vi "UHR-Fleezers Control (host) - 9.1.vi"() -> ()   [LabVIEW 2009]
uses:
  <vilib>/Utility/miscctls.llb/LVPoint32TypeDef.ctl
  <vilib>/Utility/miscctls.llb/LVMinMaxIncTypeDef.ctl
  <vilib>/userDefined/High Color/nirio_resource_hc.ctl
  <vilib>/Instr/_visa.llb/VISA Configure Serial Port (Instr).vi
  <vilib>/Platform/TimedLoop/XDataNode/XDataNode.xnode
  <vilib>/Platform/TimedLoop/XDataNode/loadlvalarms.vi
  <vilib>/Platform/TimedLoop/XDataNode/timing_clust.ctl
  <vilib>/Platform/TimedLoop/XDataNode/nitl_modes.ctl
  <vilib>/Platform/TimedLoop/XDataNode/wakeup.ctl
  <vilib>/rvi/interface/nirviOpenFPGA/nirviOpenFPGA.xnode
  FPGA Bitfiles/UHR-Fleezers Instr~3C_FPGA Target_UHR-Fleezers Contr~E1.lvbitx
  UHR-Fleezers Control (fpga) - 9.0.vi
  <vilib>/FPGAPlugInAG/PCIe-7852R/nirviIntfOpen_PCIe-7852R.vi
  <vilib>/rvi/interface/nirviMethod/nirviMethod.xnode
  <vilib>/Utility/error.llb/Merge Errors.vi
  <vilib>/LabVIEW Targets/FPGA/Rio/nirio_HostInterface/nirio_Reset.vi
  <vilib>/LabVIEW Targets/FPGA/Rio/nirio_HostInterface/nirio_DMAStopAll.vi
  <vilib>/rvi/interface/common/niFpgaNodeNameForErrorReporting.ctl
  <vilib>/rvi/errors/niLvFpgaWhatHappensToTopLevelVI.ctl
  <vilib>/LabVIEW Targets/FPGA/Rio/nirio_HostInterface/nirio_DisableInterrupts.vi
  <vilib>/Utility/error.llb/Error Cluster From Error Code.vi
  <vilib>/rvi/errors/niLvFpgaAdjustHostInterfaceError.vi
  <vilib>/rvi/interface/nirviReadWriteControl/nirviReadWriteControl.xnode
  <vilib>/LabVIEW Targets/FPGA/Rio/nirio_HostInterface/nirio_WriteBig.vi
  <vilib>/LabVIEW Targets/FPGA/Rio/nirio_HostInterface/nirio_DMAConfigure.vi
  <vilib>/LabVIEW Targets/FPGA/Rio/nirio_HostInterface/nirio_DMAStop.vi
  <vilib>/RVI Host/nirviSupport.llb/nirviErrorClusterFromErrorCode.vi
  <vilib>/LabVIEW Targets/FPGA/Rio/nirio_HostInterface/nirio_EnableInterrupts.vi
  <vilib>/rvi/errors/niLvFpgaReportInternalErrorWithAdditionalInfo.vi
  <vilib>/express/express analysis/Spectral/XNode/ExpressSpectralMeasurementsBlockNode.xnode
  <vilib>/express/express analysis/Spectral/Block/exnSpectralBlock spectral measurements PSD poly.vi
  <vilib>/express/express analysis/Spectral/Block/exnSpectralBlock spectral measurements PSD WFM.vi
  <vilib>/Waveform/WDTOps.llb/WDT Append Waveforms DBL.vi
  <vilib>/LabVIEW Targets/FPGA/Rio/nirio_HostInterface/nirio_ReadBig.vi
  <vilib>/vision/Avi1.llb/AviRefnum.ctl
  <vilib>/rvi/interface/nirviCloseFPGA/nirviCloseFPGA.xnode
  <vilib>/FPGAPlugInAG/PCIe-7852R/nirviIntfClose_PCIe-7852R.vi
  <vilib>/Analysis/NI_AALBase.lvlib
  <vilib>/Platform/TimedLoop/XDataNode/XDNodeRunTimeDep.lvlib
  openfpgaref.8.6.ctl
  NiRioSrv.dll
panel:
  in  "Total Volume\nFlushed (uL)":dbl
  in  "Flush Center Channel":bool
  in  "Inject Bottom Channel":bool
  in  "Inject Top Channel":bool
  out "Messages":string
  in  "APD Ave N":dbl=10.0
  out "Int. Time (s)":dbl
  in  "Stop All":bool
  out "sigma/mean":dbl
  out "Rate sigma (Hz)":dbl format="%0.2f"
  out "Current Stage  Position":cluster{dbl, dbl, dbl}
  in  "Index":dbl=1.0 caption="Save File Index" min=1.0 step=1.0
  in  "Tab Control 6":T1(tab)
  out "All Signals":waveform(dbl)[](graph)
  in  "Signals to Plot":i32(listbox)
  out "Trap Disp. Freq. (Hz)":dbl caption="Freq. (Hz)" format="%#_6p"
  out "Display Period (s)":dbl caption="Period (s)" format="%#_6p"
  in  "Trap Disp. Downsample":dbl=5000.0 caption="Downsample"
  in  "APD Disp. Scale":dbl=0.1 caption="Scale (Divide,\nfor above plot only)"
  in  "APD Disp. Downsample":dbl=30.0 caption="Integrate" min=1.0 step=1.0
  out "APD Display Freq. (Hz)":dbl caption="Freq. (Hz)"
  out "APD Display Period (s)":dbl caption="Period (s)"
  out "RMS (Ang)":dbl format="%_2g"
  in  "Bead Sep. Int. Time (s)":dbl=5.0 caption="Int. Time (s)"
  in  "Below (kHz)":dbl=1.0
  in  "Above (kHz)":dbl=4.0
  in  "Adjust Scale\nto Mean":bool
  in  "Rescale on Mean":bool
  in  "Offset (nm)":dbl
  out "Mean":dbl caption="Mean (pN)" format="%#_4g"
  out "Force":waveform(dbl)[](graph)
  out "APD 1 Chart":waveform(dbl)(graph)
  in  "Calibration":u16(ring)=2 items=["None", "Position", "Force"]
  out "T1 X":dbl caption="T1 X (pN)" format="%0.2f"
  out "T2 X":dbl caption="T2 X (pN)" format="%0.2f"
  out "Bead Separation":waveform(dbl)(graph)
  in  "Amplitude (nm)":dbl=1.0
  out "Bead Mean (nm)":dbl caption="Mean (nm)" format="%0.2f"
  out "Difference":dbl caption="Difference (pN)" format="%#_3g"
  out "FFT 1":cluster{"f0":dbl, "df":dbl, "magnitude":dbl[]}[](graph)
  out "FFT 2":cluster{"f0":dbl, "df":dbl, "magnitude":dbl[]}[](graph)
  in  "FFT 1 Choice 1":u16(ring) items=["T1 Y", "T1 X", "T1 Sum", "T2 Y", "T2 X", "T2 Sum", "T1 FB X", "T1 FB Sum", "T2 FB X", "T2 FB Sum", "PSD Y", "PSD X", "PSD Y Sum", "none"]
  in  "FFT 2 Choice 1":u16(ring)=13 items=["T1 Y", "T1 X", "T1 Sum", "T2 Y", "T2 X", "T2 Sum", "T1 FB X", "T1 FB Sum", "T2 FB X", "T2 FB Sum", "PSD Y", "PSD X", "PSD Y Sum", "none"]
  in  "FFT 1 Choice 2":u16(ring)=1 items=["T1 Y", "T1 X", "T1 Sum", "T2 Y", "T2 X", "T2 Sum", "T1 FB X", "T1 FB Sum", "T2 FB X", "T2 FB Sum", "PSD Y", "PSD X", "PSD Y Sum", "none"]
  in  "FFT 2 Choice 2":u16(ring)=13 items=["T1 Y", "T1 X", "T1 Sum", "T2 Y", "T2 X", "T2 Sum", "T1 FB X", "T1 FB Sum", "T2 FB X", "T2 FB Sum", "PSD Y", "PSD X", "PSD Y Sum", "none"]
  in  "Compute FFT":bool
  in  "Reset FFT":bool
  in  "# Spectra to Ave.":dbl=10.0
  out "Ave. Time (s)":dbl
  out "1 Channel":waveform(dbl)(graph)
  out "Slow mean":dbl format="%0.2f"
  in  "Slow mean N ave.":dbl=1.0 min=1.0 step=1.0
  out "Mean Intensity":dbl
  out "Sigma":dbl
  out "Sigma/Mean":dbl
  in  "Subtract mean":bool
  in  "High Res. Display":u16(ring) items=["T1 Y", "T1 X", "T1 Sum", "T2 Y", "T2 X", "T2 Sum", "T1 FB X", "T1 FB Sum", "T2 FB X", "T2 FB Sum", "PSD Y", "PSD X", "PSD Y Sum"]
  out "APD 1 Rate (Hz)":dbl format="%#_3p"
  out "Image":u32[][](graph)
  in  "Tab Control":T2(tab)=enum."Sample Stage"
  in  "Read Cal":bool
  out "Tether":bool
  in  "Tether Alarm?":bool=TRUE
  in  "Move to Delta (MHz)":dbl=15.6
  in  "Then...":string(combo)="2"
  in  "Data Acq. Spot":bool
  out "Fl. High":bool
  out "Waiting":bool
  in  "Yank to Freq. (MHz)":dbl
  in  "Fl. Threshold (kHz)":dbl
  in  "Fl. Triggered...":bool
  in  "Confocal Linescan":bool
  in  "Speed (nm/s)":dbl=100.0
  in  "Stop F (pN)":dbl=4.0
  in  "Furthest Withdraw (MHz)":dbl=15.0
  in  "Closest Delta (MHz)":dbl=10.0 step=0.25
  in  "Fish for Tether":bool
  in  "Confocal Image":bool
  in  "Round T1 X":bool caption="Round"
  in  "T1 offset_x (mV)":dbl=-26.302542012392074 format="%#_2g"
  in  "T1 kappa_x (pN/nm)":dbl=0.22546432407642192 min=0.0 step=0.001 format="%#_2g"
  out "Time (s)":dbl
  out "Total Time (s)":dbl
  in  "Start Saving":bool
  in  "Limits Enable":bool=TRUE caption="Enable"
  in  "Limit Max (MHz)":dbl=16.0 caption="Max (MHz)"
  in  "Limit Min (MHz)":dbl=10.0 caption="Min (MHz)"
  in  "Cal sets to save":u32=50 min=1 step=1
  in  "Comment (data description)":string="testing confocal setup"
  out "Calibrating Trap...":bool
  in  "Trap 2 (ON/OFF)":bool
  in  "Trap 1 (ON/OFF)":bool
  in  "Save Calibration":bool
  in  "N sets to save":u32=200 caption="N Sets"
  in  "Save N Sets":bool
  out "Save file name":path
  in  "Save ave N":dbl=250.0 caption="Averaging Factor"
  out "Saving...":bool
  in  "Stop Saving":bool
  out "Progress":u16(slide) scale=0.0..100.0
  out "Manipulating Trap":bool
  out "Buffer Status":dbl(slide) scale=0.0..1.0
  out "Overflow (data lost)":bool
  in  "Reset":bool
  out "Data Rate (Hz)":dbl caption="Trap Data Rate (Hz)" format="%#_3p"
  out "Data Period (s)":dbl caption="Trap Data Period (s)" format="%#_6p"
  out "Save Data Rate (Hz)":dbl caption="Rate (Hz)" format="%#_6p"
  out "Save Data Period (s)":dbl caption="Period (s)" format="%#_6p"
  in  "T1 alpha_x (nm/V)":dbl=630.439304367558 step=10.0 format="%#_3g"
  in  "T2 alpha_x (nm/V)":dbl=704.7738222964198 step=10.0 format="%#_3g"
  in  "T2 kappa_x (pN/nm)":dbl=0.2030110880477556 min=0.0 step=0.001 format="%#_2g"
  in  "T2 offset_x (mV)":dbl=-26.67973517613748 format="%#_2g"
  in  "BD 1 Frequency 1 (MHz)":dbl=69.4 caption="T1 X (MHz)" min=60.0 max=90.0 step=1.0 format="%#_6p"
  in  "BD 1 Frequency 2 (MHz)":dbl=85.0 caption="T2 X (MHz)" min=60.0 max=90.0 step=1.0 format="%#_6p"
  in  "Green Laser ON/Interlacing":bool
  in  "Round T2 X":bool caption="Round"
  in  "AO1":dbl(slide)=4.8 caption="Confocal Y (V)" min=0.0 max=10.0 step=0.01 scale=0.0..10.0 scale format="%_1f"
  in  "AO2":dbl(slide)=3.2 caption="Confocal X (V)" min=0.0 max=10.0 step=0.01 scale=0.0..10.0 scale format="%_1f"
  in  "Upper Cap.":bool
  in  "Lower Cap.":bool
  in  "Trap Raster Scan":bool
  out "Raster Scanning...":bool
  in  "Trap Delta (MHz)":dbl=15.599999999999994
  in  "Action":string(combo)="Alarm"
  in  "Dump Beads":bool
  out "Duration (s)":dbl
  out "Stage Moving":bool
  in  "Wait Before Save (s)":u32=1
  out "Attempts":dbl
  in  "Attempt Limit":dbl=20.0 caption="Limit"
  in  "z nudge increment (um)":dbl=0.5
  in  "+z":bool
  in  "Saved Stage Positions":T3={"Position 1"={1.03657, -0.89848, 0.0}, "Position 2"={0.0, 0.0, 0.0}, "Position 3"={2.01196, -0.50288, 0.0}, "Position 4"={2.01196, 0.31084, 0.0}} {"Position 1"."?" min=-0.1 max=0.1 step=0.1; "Position 2"."?" min=-0.1 max=0.1 step=0.1; "Position 3"."?" min=-0.1 max=0.1 step=0.1; "Position 4"."?" min=-0.1 max=0.1 step=0.1}
  in  "Position 1 Label":string="Upper capillary"
  in  "Set Position 1":bool
  in  "Set Position 2":bool
  in  "Set Position 3":bool
  in  "Set Position 4":bool
  in  "Move to Position 3":bool
  in  "Move to Position 4":bool
  in  "Move to Position 2":bool
  in  "Move to Position 1":bool
  in  "Position 2 Label":string="Lower capillary"
  in  "Position 3 Label":string="Measurement Spot"
  in  "Position 4 Label":string="Dump beads"
  in  "-z":bool
  in  "Top Ch Inject Rate (ul/h)":dbl=10.0
  in  "Pump write delay (ms)":dbl=300.0
  in  "All Pump Parameters":T4={"Pump 1"={"Diameter (mm)"=4.61, "Units"=3.0, "Volume"=100.0, "Rate"=100.0}, "Pump 2"={"Diameter (mm)"=4.61, "Units"=3.0, "Volume"=100.0, "Rate"=100.0}, "Pump 3"={"Diameter (mm)"=4.61, "Units"=3.0, "Volume"=100.0, "Rate"=100.0}}
  in  "Top Ch Inject Volume (uL)":dbl=100.0
  in  "Pump pause delay (ms)":u32
  in  "Bottom Ch Inject Volume (uL)":dbl=100.0
  in  "Bottom Ch Inject Rate (ul/h)":dbl=10.0
  in  "Flush Center Ch Volume (uL)":dbl=15.0
  in  "Flush Center Ch Rate (ul/m)":dbl=100.0
  in  "Tab Control 2":T5(tab)=enum."Feedback on BD 1 Amp to Control AI2"
  out "Total Counts (ticks)":u32
  in  "Trap ON/OFF X or Y Amp?":bool=TRUE
  in  "Oscillate Set 1":bool
  in  "Trap 1 ON":bool
  in  "Number Interlace Sets":u8=3 min=1 max=3
  in  "DIO count 3 (ticks)":u32=200
  in  "DIO count 2 (ticks)":u32=200
  in  "DIO count 1 (ticks)":u32=200
  in  "BD 2 Amplitude 3 (%)":dbl min=0.0 max=50.0 step=1.0
  in  "BD 2 Amplitude 2 (%)":dbl min=0.0 max=50.0 step=1.0
  in  "BD 2 Amplitude 1 (%)":dbl min=0.0 max=50.0 step=1.0
  in  "BD 1 Amplitude 3 (%)":dbl min=0.0 max=50.0 step=1.0
  in  "BD 1 Amplitude 2 (%)":dbl=35.0 min=0.0 max=50.0 step=1.0
  in  "BD 1 Amplitude 1 (%)":dbl=10.0 min=0.0 max=50.0 step=1.0
  in  "BD 2 Frequency 3 (MHz)":dbl=26.0 min=0.0 max=40.0 step=1.0 format="%#_6p"
  in  "BD 1 Frequency 3 (MHz)":dbl=70.0 min=60.0 max=90.0 step=1.0 format="%#_6p"
  in  "BD 2 Frequency 2 (MHz)":dbl=26.0 min=0.0 max=40.0 step=1.0 format="%#_6p"
  in  "BD 2 Frequency 1 (MHz)":dbl=26.0 min=0.0 max=40.0 step=1.0 format="%#_6p"
  in  "Not-Interlacing Set":enum32{"Set 1", "Set 2", "Set 3"}(radio)
  in  "Interlace":bool=TRUE
  in  "Trap 2 ON":bool
  in  "Trap 3 ON":bool
  in  "Scan axis 2":bool=TRUE
  in  "Osc. freq. (Hz)":dbl=0.25
  in  "Osc. amp. (MHz)":dbl=2.0
  out "Coords":T6
  in  "Manipulation Scaling":cluster{"Horizontal":dbl, "Vertical":dbl}={"Horizontal"=0.075, "Vertical"=0.01}
  in  "Freq or Amp switch first":bool=TRUE
  in  "Swap F1 and F2":bool
  in  "Freq switch delay":u16
  in  "Amp switch delay":u16=5
  in  "MCL Step Increment (V_int)":dbl=3.0
  out "Time to Finish All (min)":dbl format="%#_2p"
  in  "Scan Speed (nm/s)":dbl=100.0
  in  "Scan Range (nm)":dbl=750.0
  in  "Step Size (nm)":dbl=1.0
  in  "MCL/AOM Scale Tweak":dbl=1.0
  in  "MCL Step Position Ratio":dbl=0.5
  in  "Move MCL Also?":bool=TRUE
  out "Final sep (nm)":dbl
  out "Initial sep (nm)":dbl
  out "Save index":dbl
  out "Final delta (MHz)":dbl
  out "Initial delta (MHz)":dbl
  out "Final freq. (MHz)":dbl
  out "Initial freq. (MHz)":dbl
  in  "Saved AOD Raster Scan Parameter Sets":T7(array[cluster])=[{"Scan Range AOD (nm) 2"=500.0, "Step Size AOD (nm) 2"=1.0, "Scan Speed AOD (nm/s) 2"=200.0, "Number of scans (AOD) 2"=1, "Label"=""}, {"Scan Range AOD (nm) 2"=1000.0, "Step Size AOD (nm) 2"=1.0, "Scan Speed AOD (nm/s) 2"=200.0, "Number of scans (AOD) 2"=5, "Label"="wide offset scan"}, {"Scan Range AOD (nm) 2"=20.0, "Step Size AOD (nm) 2"=0.68, "Scan Speed AOD (nm/s) 2"=0.68, "Number of scans (AOD) 2"=1, "Label"="2 bp steps"}]
  in  "Load parameters":bool
  out "Scan Range (MHz)":dbl=10.0
  in  "Restart DMA? (AOD)":bool=TRUE caption="Restart DMA?"
  out "Incr. int (AOD)":i64
  out "Time/Scan (s) (AOD)":dbl format="%#_2p"
  out "Data points/scans":dbl
  out "Data points/scan (f/b)":dbl
  in  "Save scans":bool=TRUE
  out "AOD Scan I":u64 caption="Scan I"
  in  "Continuous AOD Scanning":bool caption="Continuous Scanning"
  in  "Abort AOD Scan":bool caption="Abort Scan"
  in  "Scan BD":bool=TRUE
  out "Cycles/step (AOD)":u64=400 format="%.0p"
  in  "Number of F/B Scans (AOD)":u16=3 min=1
  out "Scan steps (AOD)":u64=1000
  out "Scan Increment (MHz)":dbl=0.2
  out "AOD Scanning":bool caption="Scanning"
  in  "Start AOD Scan":bool caption="Start Scan"
  out "N sets should be saved":dbl
  out "Progress 2":u16(slide) caption="Progress" scale=0.0..100.0
  in  "Abort save 2":bool caption="Abort save"
  in  "Trap 1 Bead Size (nm)":dbl=860.0
  in  "Trap 2 Bead Size (nm)":dbl=790.0
  out "MCL Count":dbl
  in  "All FB On/Off":bool=TRUE
  in  "AI2 to Setpoint":cluster{"Set 1":bool, "Set 2":bool}
  out "AI2 (V)":cluster{"Set 1":dbl, "Set 2":dbl}
  in  "Reset Feedback":cluster{"Set 1":bool, "Set 2":bool}
  in  "PID Gains":T8={"Set 1"={"proportional gain (Kc)"=0, "integral gain (Kc*Ts/Ti)"=5, "derivative gain (Kc*Td/Ts)"=0}, "Set 2"={"proportional gain (Kc)"=0, "integral gain (Kc*Ts/Ti)"=5, "derivative gain (Kc*Td/Ts)"=0}}
  in  "Setpoints (V)":cluster{"Set 1":dbl, "Set 2":dbl}={"Set 1"=7.0, "Set 2"=7.0}
  in  "Feedback On/Off":cluster{"Set 1":bool, "Set 2":bool}={"Set 1"=TRUE, "Set 2"=TRUE}
  in  "Tab Control 3":enum32{"Timing", "MCL Scan", "Analog Out"}(tab)
  out "APD Gate Late Counter":u32
  in  "- phase (APD Gate)":bool
  in  "+ phase (APD Gate)":bool
  out "APD Gate Relative Phase":i16
  in  "Phase Adj. (APD Gate)":i16=20
  in  "Initial Phase Adjustment (APD Gate)":i16=95
  in  "Save APD Data\nwith Trap Data":bool=TRUE
  out "APD FIFO Elements Remaining":u32
  in  "- phase (APD Acq)":bool
  in  "+ phase (APD Acq)":bool
  out "APD Acq Late Counter":u32
  out "APD Acq Relative Phase":i16
  in  "Phase Adj. (APD Acq)":i16=20
  in  "Initial Phase Adjustment (APD Acq)":i16
  in  "Invert APD Gate":bool caption="Invert Gate"
  in  "APD Gate OFF Count":u32=450 caption="Gate OFF Count"
  in  "APD Gate ON Count":u32=150 caption="Gate ON Count"
  in  "APD Gate":enum32{"ON", "OFF", "Interlace"}(radio)=enum."Interlace"
  in  "APD Integration Time (s)":dbl=0.01 caption="Integration Time (s)"
  out "APD Acq Rate (Hz)":dbl=20000000.0 caption="Rate (Hz)"
  out "APD Samples/FIFO Acq.":dbl
  out "APD Elements/DMA read":u32
  out "APD Int. Count":u32 format="%.0p"
  in  "Tab Control 8":enum32{"APD 1 Image", "APD 1 Line Scan"}(tab)
  out "APD 1 map":dbl[][](graph)
  out "Waveform Graph":dbl[](graph)
  in  "Tab Control 5":enum32{"PSD X", "PSD Y", "Other Data Channel"}(tab)
  out "PSD X map":dbl[][](graph)
  out "PSD Y map":dbl[][](graph)
  out "Data map":dbl[][](graph)
  in  "Channel":i32=4
  in  "Abort MCL Scan":bool
  out "MCL Scan I":u64
  out "MCL Scanning":bool
  in  "Start MCL Scan":bool
  out "wait to reset values":bool
  in  "Tab Control 4":enum32{"Scan Settings", "MCL FPGA Loop Timing"}(tab)
  out "Total Time (s)":dbl
  in  "Scan lines":u64=10
  in  "Fast Scan Dir":bool=TRUE
  in  "2D or 1D Scan":bool=TRUE
  out "Initial X":dbl
  out "Initial Y":dbl
  out "Time/f+b scan (s) (MCL)":dbl caption="Time/scan (s)"
  in  "Number of scans (MCL)":u64=1 caption="Scans"
  in  "Scan steps (MCL)":u64=20 caption="Scan steps"
  in  "N APD Samp/step":dbl=6.0
  in  "Scan Range (V)":dbl=3.0
  in  "Restart DMA? (MCL)":bool=TRUE caption="Restart DMA?"
  in  "Continuous MCL Scanning":bool caption="Cont. Scanning"
  in  "Center Scan":bool=TRUE
  in  "Save Data (MCL)":bool=TRUE caption="Save Data"
  out "Incr. int (MCL)":i16 caption="Incr. int"
  out "Actual incr":dbl
  out "Scan Increment (V)":dbl
  out "N sets should be saved (MCL)":dbl caption="N sets should be saved"
  out "Data points/scans (MCL)":dbl caption="Data points/scans"
  out "Data points/scan (f+b)":dbl caption="points/scan (f+b)"
  out "Cycles/step (MCL)":u64 caption="Cycles/step" format="%.0p"
  in  "Phase adjust (MCL)":i16 caption="Phase adjust"
  out "Relative Phase (MCL)":i16 caption="Relative Phase"
  in  "Initial Phase Adj. (MCL)":i16 caption="Initial Phase Adj."
  in  "Update Count (MCL)":u32=800
  in  "+ phase (MCL)":bool
  in  "- phase (MCL)":bool
  out "MCL Late Counter":u32
  in  "APD 1 AO Mult.":i16=1 min=1
  in  "APD 2 AO Mult.":i16=1 min=1
  in  "APD 1 AO offset":i16
  in  "APD 2 AO offset":i16
  in  "Tab Control 7":enum32{"Green FB Signals", "Slow MCL Scan"}(tab)
  out "Green FB Plot":dbl(graph)
  out "MCL Scan 2":cluster{"Begin (V)":dbl, dbl, dbl[]}(graph)
  out "MCL Scan":cluster{"Begin (V)":dbl, dbl, dbl[]}(graph)
  in  "Green laser mode":enum32{"Laser ON", "Laser OFF", "Interlace"}(radio)=enum."Interlace"
  in  "GI Frequency, ON count":u32=150 min=1 step=1
  in  "Invert GI":bool
  out "GI Late Counter":u32
  in  "Phase adj. (GI)":i16=5
  out "GI relative phase":i16
  in  "+ phase (GI)":bool
  in  "Initial Phase Adjustment (GI)":i16=15
  in  "GI Frequency, OFF count":u32=450 min=1 step=1
  in  "- phase (GI)":bool
  out "Green FB Signals (V)":cluster{"Y":dbl, "X":dbl, "Sum":dbl}
  out "Relative phase (Green FB)":i16
  in  "+ phase (Green FB)":bool
  in  "- phase (Green FB)":bool
  in  "Green FB Count":u32=600
  in  "Phase adj. (Green FB)":i16=10
  in  "Initial Phase Adjustment (Green FB)":i16=50
  in  "Green FB On/Off":bool=TRUE
  in  "Current When FB OFF (%)":dbl=65.0 min=0.0 max=100.0 step=1.0
  in  "Green int current ON count adj":u32=150
  in  "Green FB Gains":T9={"proportional gain (Kc)"=10, "integral gain (Kc*Ts/Ti)"=5, "derivative gain (Kc*Td/Ts)"=0}
  in  "Green FB Setpoint (mV)":dbl=125.0
  in  "- phase (GI) 2":bool
  in  "Initial Phase Adjustment (GI) 2":i16=-100
  in  "+ phase (GI) 2":bool
  out "GI relative phase 2":i16
  in  "Phase adj. (GI) 2":i16=20
  out "GI Late Counter 2":u32
  in  "# Samples/trap":dbl=10000.0 format="%#_6p"
  out "Elements/DMA read":u32 format="%.0p"
  out "Ave. Rate (Hz)":dbl format="%#_6p"
  out "FIFO El. Rem.":u32 format="%.0p"
  in  "Phase adj. (AI1)":i16=15
  out "Relative phase (AI1)":i16
  in  "+ phase (AI1)":bool
  in  "- phase (AI1)":bool
  out "Late Counter (AI1)":u32
  in  "Initial Phase Adjustment (AI1)":i16=220
  out "AI rate (Hz)":dbl=50000.0 format="%#_6p"
  in  "AI Count (ticks)":u32=800
  out "# Samples/channel":u32=20000 format="%.0p"
  in  "FIFO Depth":u32=600000 format="%.0p"
  in  "Detector Type":string(combo)="IR-QPD + PSD + FB-QPD X position"
  in  "N Acq Sets (Traps)":i16=3
  in  "Sets to FIFO (Traps)":T10={"Set 1"=TRUE, "Set 2"=TRUE, "Set 3"=FALSE}
  in  "FPGA Ave.":dbl=1.0 min=1.0 step=1.0
  out "Ave. Period (s)":dbl format="%#_6p"
  out "DMA Update Period (s)":dbl
  out "FPGA Averaging":bool
  out "Trap Sets":i16
  out "Counts/DMA":dbl format="%#_6p"
  in  "Video Capture Rate (Hz)":dbl=30.0
  in  "Video Index":dbl=1.0 min=1.0 step=1.0
  in  "New Video File":bool
  in  "Capture Video":bool
  in  "Reset Averaging":bool
  in  "Averaging":bool
  in  "Capture and Save Image":bool
  in  "Image Index":dbl=1.0 min=1.0
  out "Path Out":path
  out "error out":errorcluster
  out "error out 2":errorcluster
  in  "Lost Tether Alarm Threshold (pN)":dbl=0.5
  in  "AOM X Cal (nm/MHz)":dbl=123.0
  in  "MCL X Cal (nm/V)":dbl=1070.0
  out "X RF Amplitude Limits (%)":T11={"Minimum"=0.0, "Maximum"=50.0, "Increment"=1.0}
  out "X RF Frequency Limits (MHz)":T11={"Minimum"=60.0, "Maximum"=90.0, "Increment"=1.0}
  out "Y RF Frequency Limits (MHz)":T11={"Minimum"=60.0, "Maximum"=90.0, "Increment"=1.0}
  out "Y RF Amplitude Limits (%)":T11={"Minimum"=0.0, "Maximum"=50.0, "Increment"=1.0}
  in  "Manip. X?":bool=TRUE
  in  "Manip. Y?":bool
  in  "Force Manip Abort":bool
  out "Read cal error":errorcluster
  in  "DAQ Delay (ms)":u32=1000
  in  "Start Scan":bool
  in  "Scan axis":bool=TRUE
  in  "Osc. amp. (V)":dbl=5.0
  in  "Osc. center (V)":dbl=5.0
  in  "Osc. freq. (Hz) 2":dbl=1.0
  in  "MCL Mode":u16(ring) items=["Manual Positioning", "Sinusoidal Wave", "Linear Scan"]
  in  "Begin (V)":dbl
  in  "End (V)":dbl=10.0
  in  "N Points":dbl=20.0
  in  "Delay to Interlace (s)":dbl
  in  "Delayed Interlace Start":bool
  in  "Read Lateness and Rel Phase":bool
  out "Vec Mean of T1 T2":dbl[](array[numeric])
  in  "Cal read wait (s)":u32=5
  out "Time tether formed":timestamp
  in  "Sample Chamber Stage Serial Port":refnum<visa-resource-name>="COM5"
  in  "Syringe Pump Serial Port":refnum<visa-resource-name>="COM3"
  # "Trap Display:"
  # "APD Display:"
  # "DAQ"
  # "Move Stage and Take Action"
  # "Trap Manipulation"
  # "Data Saving"
  # "Bead Calibration"
  # "Trap Position Difference Limits"
  # "Center channel"
  # "Units: \n1 = ml/m\n2 = ml/h\n3 = ul/m\n4 = ul/h"
  # "Rate param is ul/h\nVolume param is ul"
  # "X"
  # "Y"
  # "Oscillate Set 1 freq. (debugging)"
  # "BD 1"
  # "BD 2"
  # "AOD Raster Scan"
  # "Approx. trap separations"
  # "X"
  # "Y"
  # "Gate"
  # "X"
  # "2D"
  # "Y"
  # "1D"
  # "Green Laser Interlacing"
  # "Green FB Measurement"
  # "Digital Gate"
  # "Current Analog Control"
  # "Total AI Rates (NOT rates/trap)"
  # "(Samples/trap x Trap Sets)"
  # "(Samples/channel x\n8 if averaging (8 channels)\n4 if no averaging)"
  # "Trap 1"
  # "Trap 2"
  # "Flour./Trap 3"
  # "MCL Position Debugging"
  # "Temporary Control Storage\n(these used to be somewhere else, still want to keep them)"
  # "Y"
  # "X"
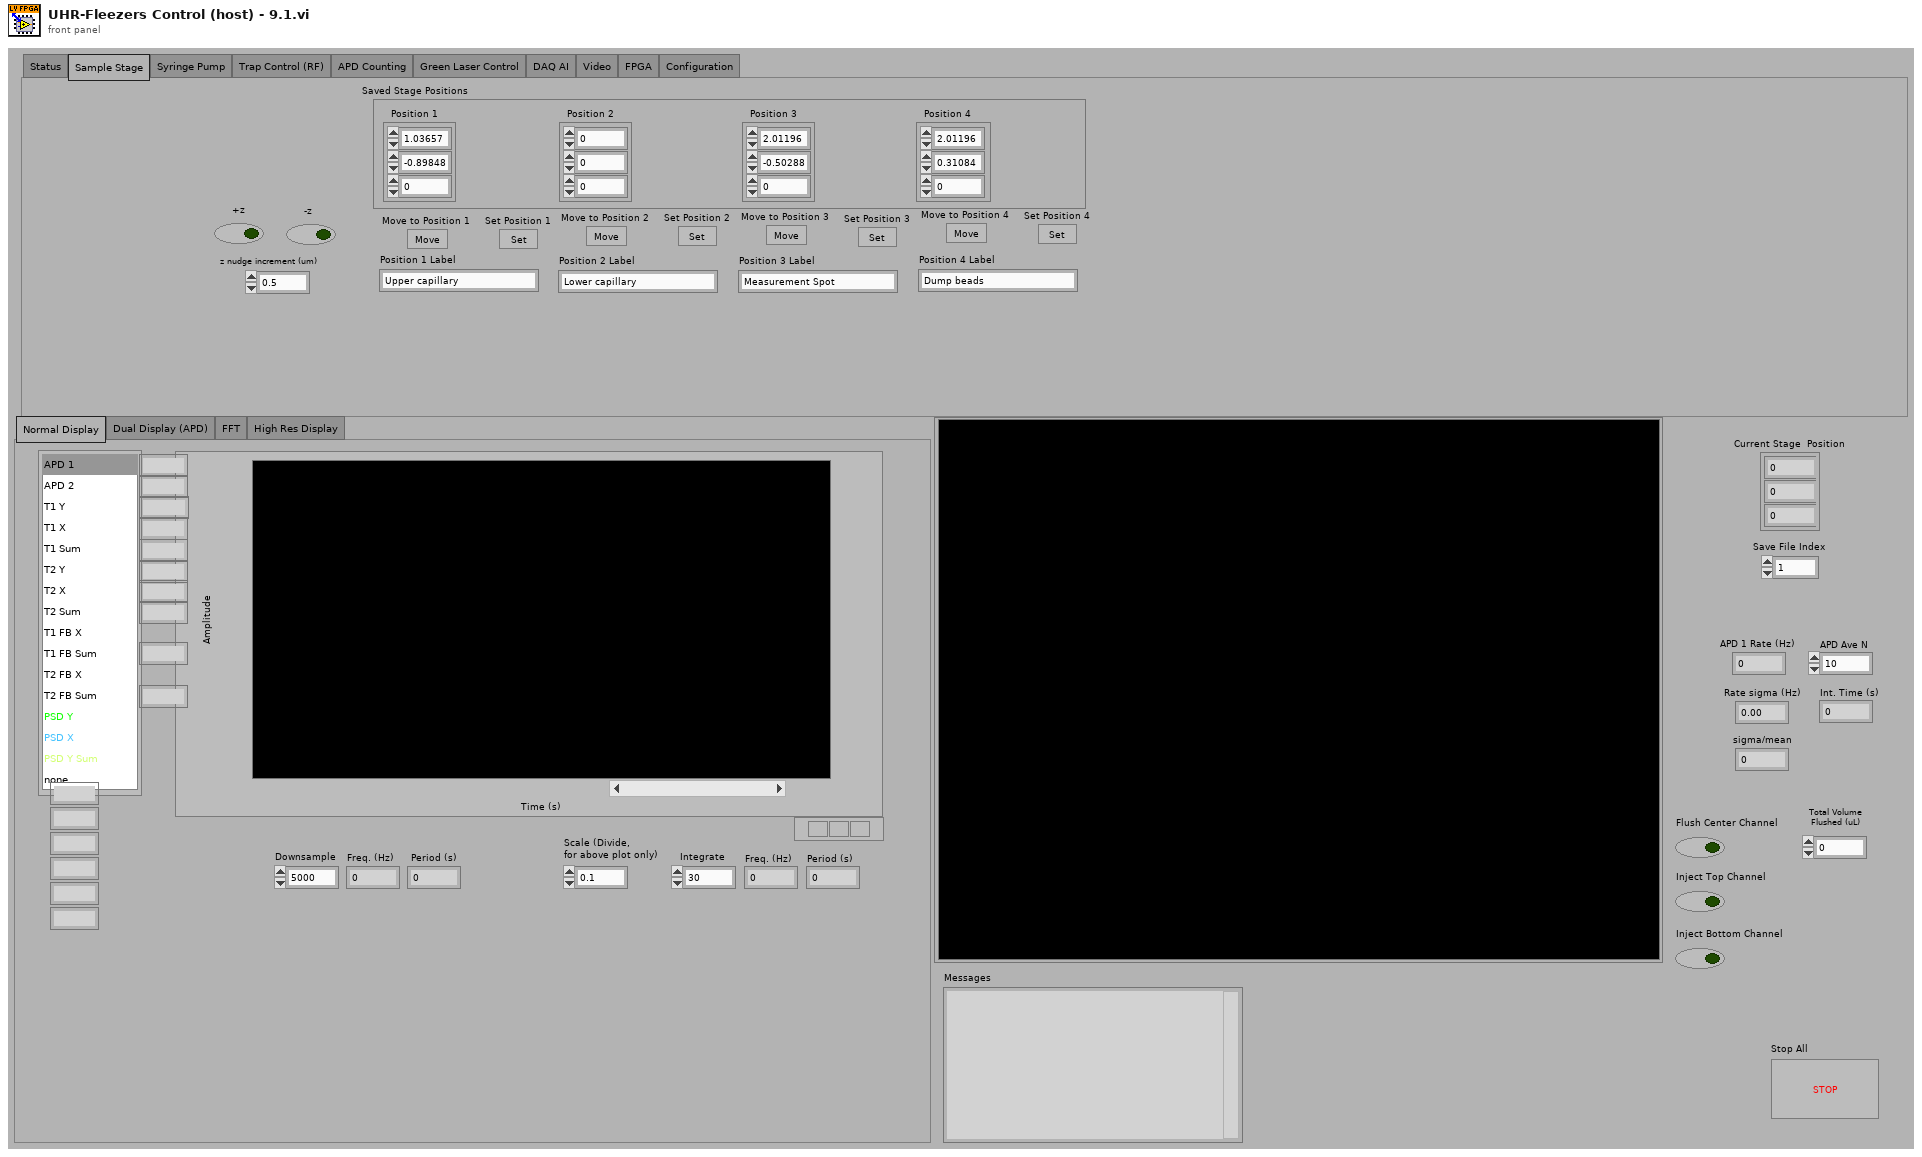
[diagram p1: front panel]
types:
  T1 = enum32{"Normal Display", "Dual Display (APD)", "FFT", "High Res Display"}
  T2 = enum32{"Status", "Sample Stage", "Syringe Pump", "Trap Control (RF)", "APD Counting", "Green Laser Control", "DAQ AI", "Video", "FPGA", "Configuration"}
  T3 = cluster{"Position 1":cluster{dbl, dbl, dbl}, "Position 2":cluster{dbl, dbl, dbl}, "Position 3":cluster{dbl, dbl, dbl}, "Position 4":cluster{dbl, dbl, dbl}}
  T4 = cluster{"Pump 1":cluster{"Diameter (mm)":dbl, "Units":dbl, "Volume":dbl, "Rate":dbl}, "Pump 2":cluster{"Diameter (mm)":dbl, "Units":dbl, "Volume":dbl, "Rate":dbl}, "Pump 3":cluster{"Diameter (mm)":dbl, "Units":dbl, "Volume":dbl, "Rate":dbl}}
  T5 = enum32{"IR Laser Interlacing (Direct RF Board Control Method)", "AOD Raster Scan", "Feedback on BD 1 Amp to Control AI2"}
  T6 = typedef "LVPoint32TypeDef.ctl" = cluster{"Horizontal":i32, "Vertical":i32}
  T7 = cluster{"Scan Range AOD (nm) 2":dbl, "Step Size AOD (nm) 2":dbl, "Scan Speed AOD (nm/s) 2":dbl, "Number of scans (AOD) 2":u16, "Label":string}[]
  T8 = cluster{"Set 1":cluster{"proportional gain (Kc)":i16, "integral gain (Kc*Ts/Ti)":i16, "derivative gain (Kc*Td/Ts)":i16}, "Set 2":cluster{"proportional gain (Kc)":i16, "integral gain (Kc*Ts/Ti)":i16, "derivative gain (Kc*Td/Ts)":i16}}
  T9 = cluster{"proportional gain (Kc)":i16, "integral gain (Kc*Ts/Ti)":i16, "derivative gain (Kc*Td/Ts)":i16}
  T10 = cluster{"Set 1":bool, "Set 2":bool, "Set 3":bool}
  T11 = typedef "LVMinMaxIncTypeDef.ctl" = cluster{"Minimum":dbl, "Maximum":dbl, "Increment":dbl}
  T12 = typedef "nirio_resource_hc.ctl" = tag
  T13 = typedef "openfpgaref.8.6.ctl" = refnum<k20>
  T14 = typedef "niFpgaNodeNameForErrorReporting.ctl" = enum16{"Open FPGA VI Reference", "Read/Write Control", "Invoke Method: Abort", "Invoke Method: Acknowledge IRQ", "Invoke Method: Download", "Invoke Method: FIFO.Configure", "Invoke Method: FIFO.Read", "Invoke Method: FIFO.Start", "Invoke Method: FIFO.Stop", "Invoke Method: FIFO.Write", "Invoke Method: Reset", "Invoke Method: Run", "Invoke Method: Wait on IRQ", "Close FPGA VI Reference"}
  T15 = typedef "niLvFpgaWhatHappensToTopLevelVI.ctl" = enum16{"top level VI scripted behind XNode", "top level VI inlined behind XNode"}
  T16 = typedef "XDNodeRunTimeDep.lvlib/timing_clust.ctl" = cluster{"Expected End [f-1]":u64, "Actual End [f-1]":u64, "Finished Late? [f-1]":bool, "Expected End [i-1]":u64, "Actual End [i-1]":u64, "Finished Late? [i-1]":bool, "Expected Start [i]":u64, "Actual Start [i]":u64, "Expected Start [f]":u64, "Actual Start [f]":u64, "Source Name":string, "Structure Name":string, "Period":i64, "Deadline":i64, "Offset":i64, "Start":i64, "Priority":i32, "Timeout":i32, "Mode":T17, "Wakeup Reason":T18, "Error":errorcluster, "Source Type":string, "Secondary Source Type":string, "Global End Time":u64, "Global Start Time":u64, "Frame Duration":u64, "Iteration Duration":u64, "Assigned CPU":i32, "I/O Scan Engine Mode":u32}
  T17 = typedef "XDNodeRunTimeDep.lvlib/nitl_modes.ctl" = enum32{"No Change", "Process missed periods, maintain original phase", "Discard missed periods, maintain original phase", "Process missed periods, ignore original phase", "Discard missed periods, ignore original phase"}
  T18 = typedef "XDNodeRunTimeDep.lvlib/wakeup.ctl" = enum32{"Normal", "Aborted", "Asynchronous wakeup", "Timing source error", "Timed loop error", "Timeout"}
  T19 = enum16{"big-endian, network order", "native, host order", "little-endian"}
  T20 = enum16{"open", "replace", "create", "open or create", "replace or create", "replace or create with confirmation"}
  T21 = cluster{"Scan Range AOD (nm) 2":dbl, "Step Size AOD (nm) 2":dbl, "Scan Speed AOD (nm/s) 2":dbl, "Number of scans (AOD) 2":u16, "Label":string}
  T22 = cluster{"[0]":dbl, "[1]":dbl, "[2]":dbl, "[3]":dbl, "[4]":dbl, "[5]":dbl}
  T23 = cluster{"Diameter (mm)":dbl, "Units":dbl, "Volume":dbl, "Rate":dbl}
  T24 = enum32{"setting", "request", "request control", "info", "statistics", "system settings", "I/O sub system", "HRT control", "camera descriptions", "device specific data", "event sub system settings", "event sub system results", "image memory manager"}
  T25 = typedef "AviRefnum.ctl" = refnum<k1>
  T26 = typedef "Image Type" = u32
  T27 = typedef "IMAQ Image.ctl" = refnum<image>
  T28 = typedef "imagedata.ctl" = cluster{"image type":i32, "image depth":i32, "image":u8[], "mask":u8[], "colors":u32[], "Rectangle":cluster{"left":i16, "top":i16, "right":i16, "bottom":i16}}
  T29 = cluster{"averaging mode":u16, "weighting mode":u16, "number of averages":u32}
  T30 = cluster{"dB On (F)":bool, "unwrap phase (F)":bool, "convert to degree (F)":bool}
  T31 = cluster{"Green FB Ch 0":i16, "Green FB Ch 1":i16, "Green FB Ch 2":i16}
  T32 = cluster{string, string, string, string, string, string, string, string}
  T33 = cluster{string, string, string, string, string, string, string, string, string, string, string, string}
  T34 = cluster{string, string, string, string, string, string, string, string, string, string, string, string, string}
  T35 = cluster{string, string, string, string, string, string, string, string, string, string, string, string, string, string}
  T36 = cluster{"f0":dbl, "df":dbl, "magnitude":dbl[]}[][]
  T37 = cluster{"Green FB Ch 0":dbl, "Green FB Ch 1":dbl, "Green FB Ch 2":dbl}
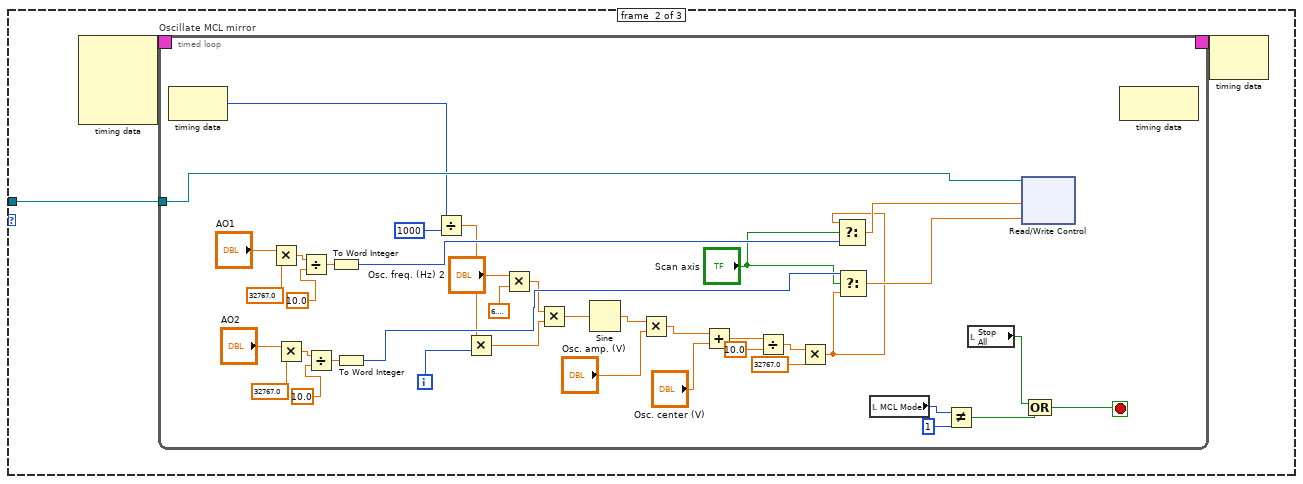
[diagram p2: hidden frame]
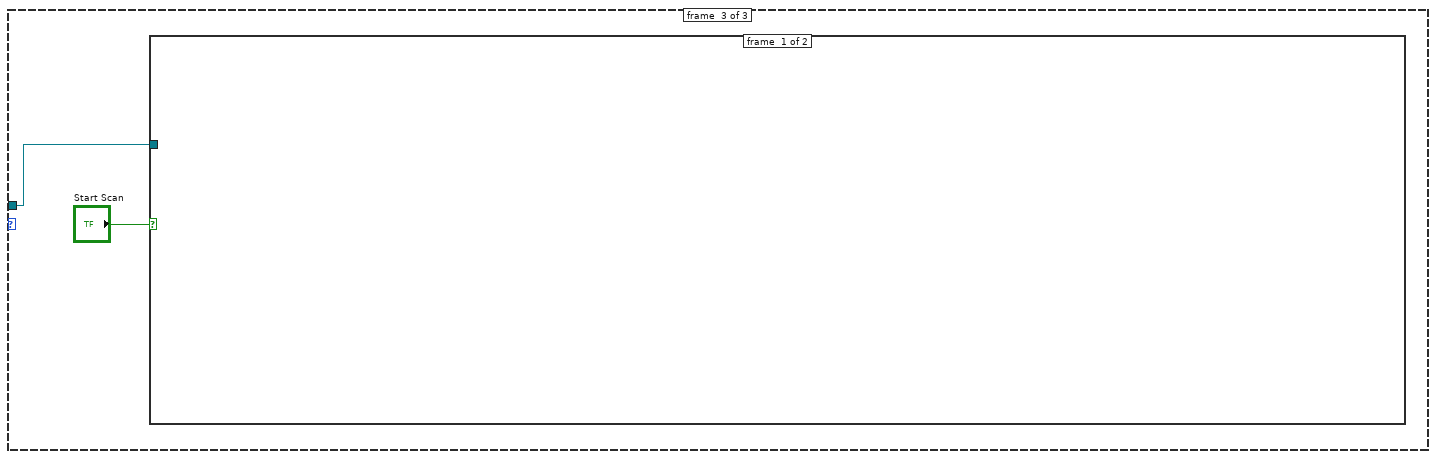
[diagram p3: hidden frame]
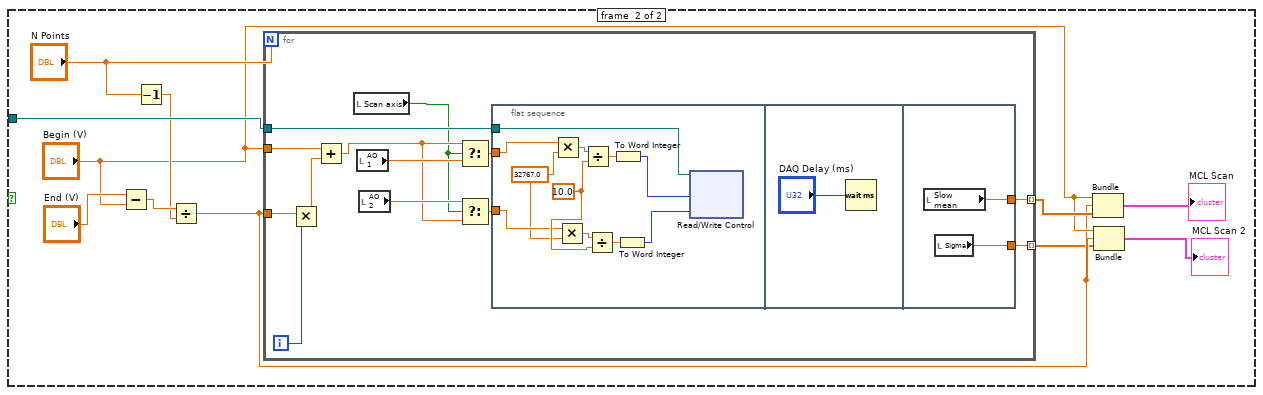
[diagram p4: hidden frame]
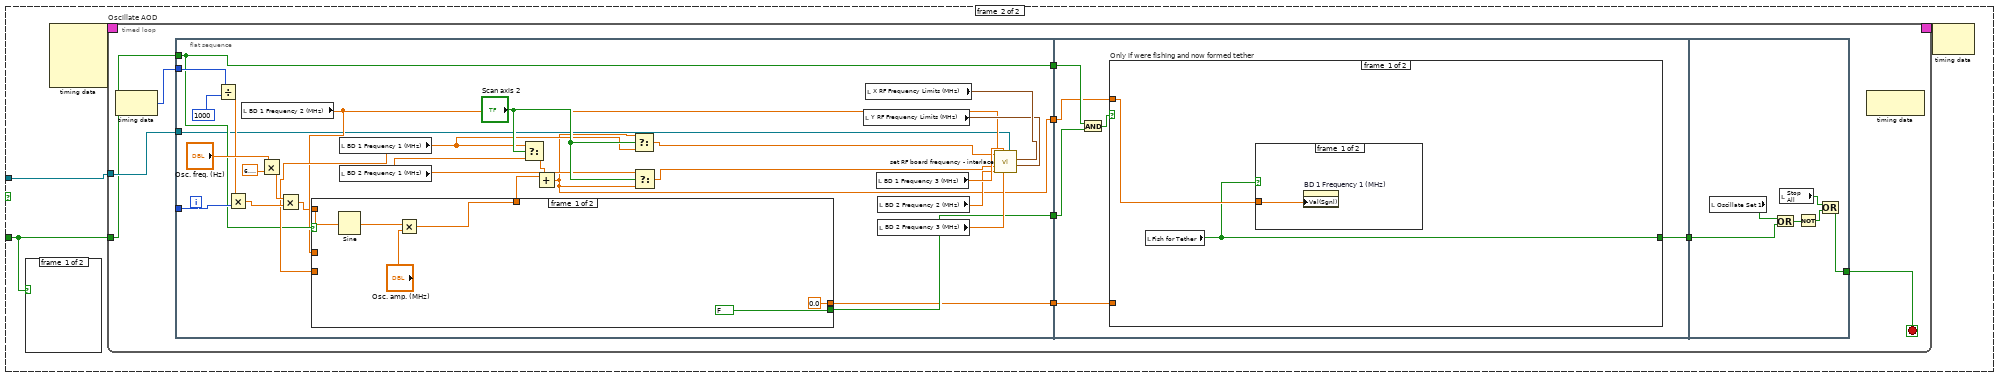
[diagram p5: hidden frame]
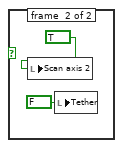
[diagram p6: hidden frame]
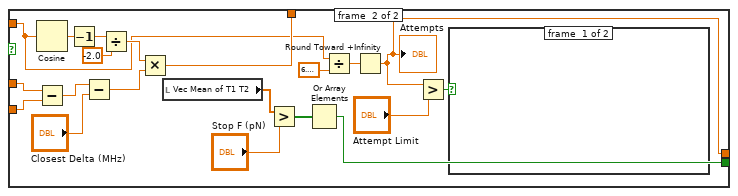
[diagram p7: hidden frame]
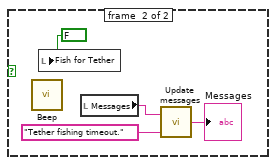
[diagram p8: hidden frame]
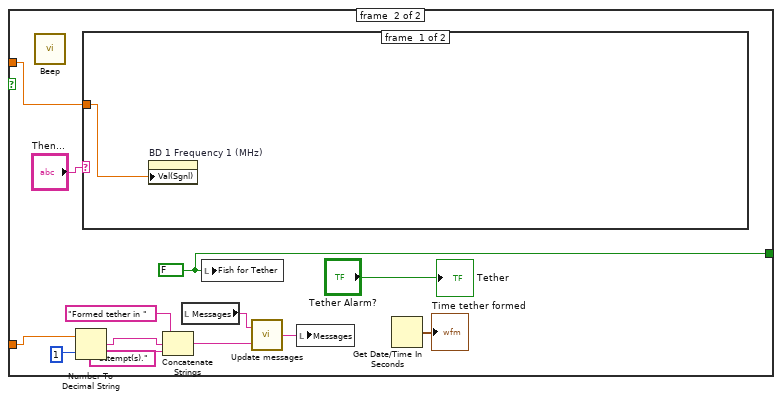
[diagram p10: hidden frame]
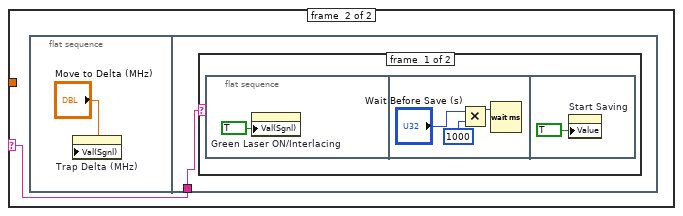
[diagram p11: hidden frame]
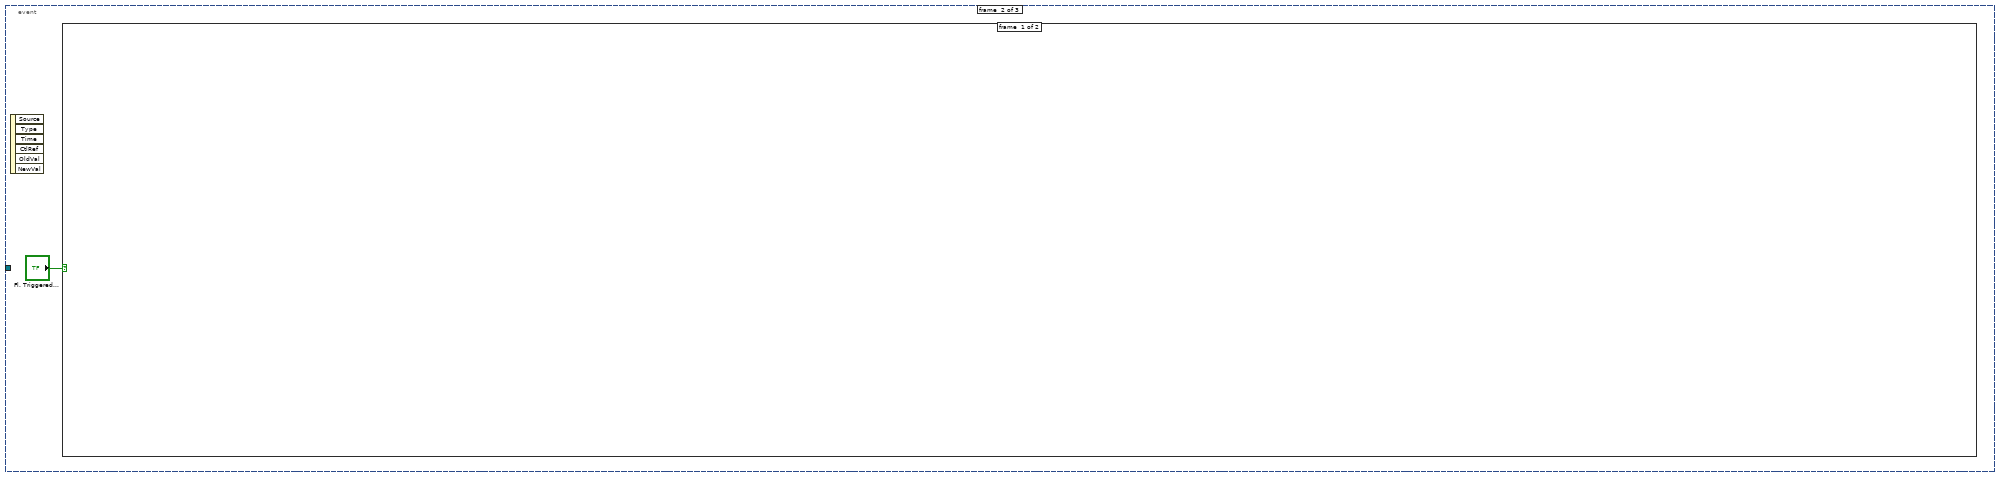
[diagram p13: hidden frame]
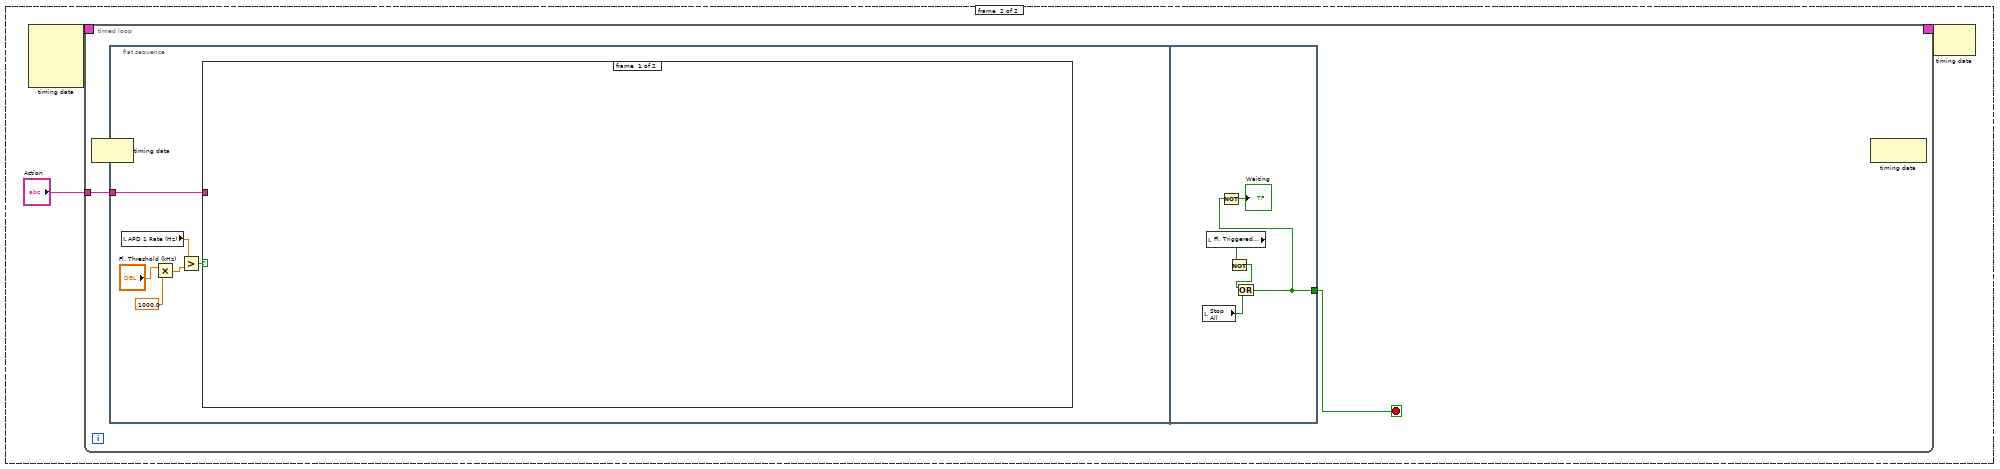
[diagram p14: hidden frame]
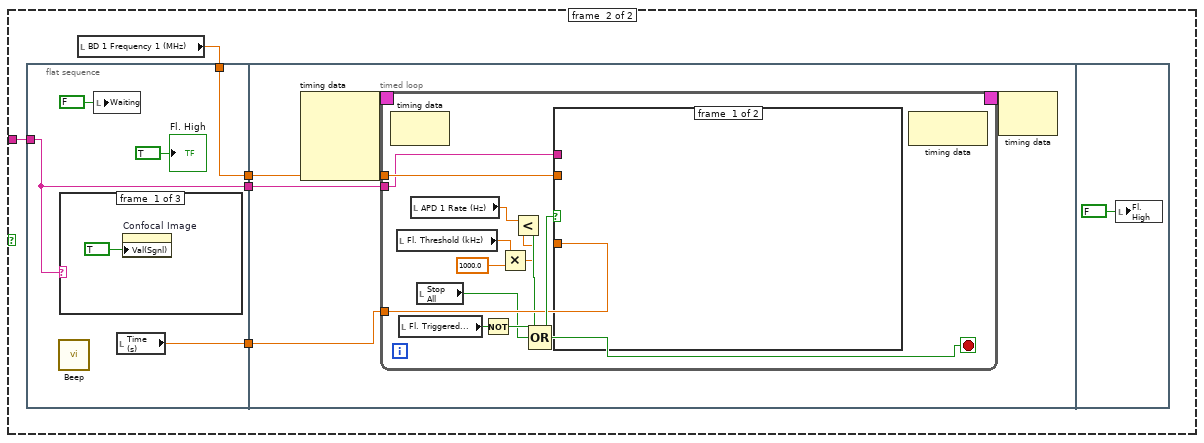
[diagram p15: hidden frame]
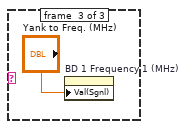
[diagram p17: hidden frame]
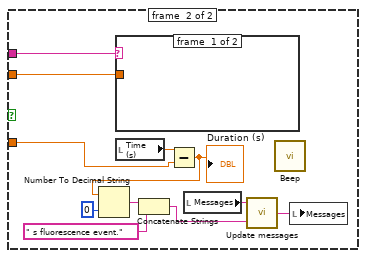
[diagram p18: hidden frame]
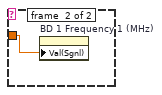
[diagram p19: hidden frame]
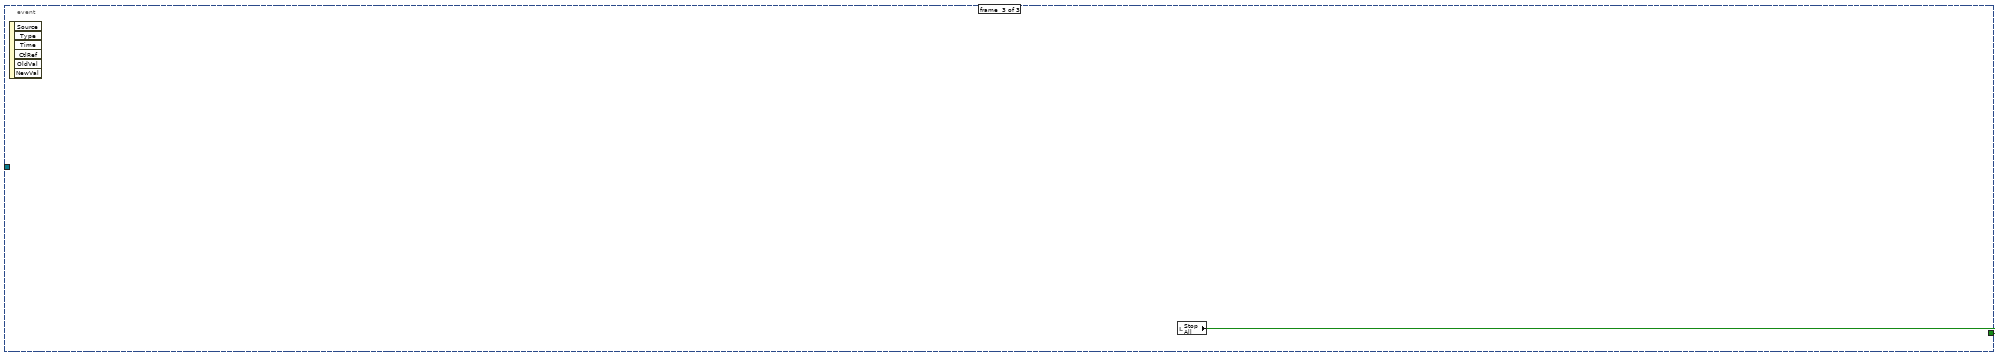
[diagram p20: hidden frame]
diagram:
  w52 = T11 {"Minimum"=-0.1, "Maximum"=0.1, "Increment"=0.1}  # Z Limits
  w65 = cluster{"output high":i16, "output low":i16} {"output high"=3000, "output low"=0} ("FB output range 1")
  w71 = TRUE ("AI to FIFO")
  w156 = 10.0 ("y")
  w155 = 32767.0 ("y")
  w171 = 6.0  # clock mult.
  w172 = 49152000.0  # TCXO frequ.
  n1 = Build Array("DIO count 1 (ticks)", "DIO count 2 (ticks)", "DIO count 3 (ticks)") -> (w47:u32[])
  n2 = Multiply(x="APD Integration Time (s)", y=40000000.0) -> (x*y=w79:dbl)
  n3 = Reciprocal(x="APD Integration Time (s)") -> (1/x=w76:dbl)
  n4 = local write "APD Acq Rate (Hz)"(w76) -> ()
  n5 = local read "AO1"() -> (w150:dbl)
  n6 = local read "AO2"() -> (w149:dbl)
  n7 = To Unsigned Long Integer(number=w79) -> (unsigned 32bit integer=w78:u32)
  "APD Int. Count" <- w78
  n8 = local read "Scan Increment (MHz)"() -> (w167:dbl)
  n9 = local read "Fast Scan Dir"() -> (w136:bool)
  n10 = local read "Continuous MCL Scanning"() -> (w137:bool)
  n11 = Multiply(x=w150, y=w155) -> (x*y=w152:dbl)
  n12 = Multiply(x=w149, y=w155) -> (x*y=w154:dbl)
  n13 = local read "Number of scans (MCL)"() -> (w138:u64)
  n14 = Divide(x=w152, y=w156) -> (x/y=w151:dbl)
  n15 = Divide(x=w154, y=w156) -> (x/y=w153:dbl)
  n16 = To Word Integer(number=w151) -> (16bit integer=w148:i16)
  n17 = To Word Integer(number=w153) -> (16bit integer=w147:i16)
  n18 = Not(x=w136) -> (.not. x?=w131:bool)
  n19 = local read "Cycles/step (MCL)"() -> (w139:u64)
  n20 = Multiply(x=w167, y=1000.0) -> (x*y=w174:dbl)
  n21 = local read "Scan steps (MCL)"() -> (w140:u64)
  n22 = local read "Scan Increment (V)"() -> (w142:dbl)
  n23 = Scale By Power Of 2(n=48, x=w174) -> (x*2^n=w175:dbl)
  n24 = Multiply(x=w172, y=w171) -> (x*y=w170:dbl)
  n25 = Divide(x=w175, y=w170) -> (x/y=w169:dbl)
  n26 = local read "Setpoints (V)"() -> (w195:cluster{"Set 1":dbl, "Set 2":dbl})
  n27 = property on="AI Count (ticks)" class="DigNum (strict)"("Val(Sgnl)"="AI Count (ticks)") -> ()  [unwired: 2 in, 2 out]
  n28 = local read "Number Interlace Sets"() -> (w40:u8)
  n29 = Split 1D Array(array=w47, index=w40) -> (first subarray=w49:u32[])  [unwired: 1 out]
  n30 = Add Array Elements(numeric array=w49) -> (sum=w48:u32)
  n31 = To Quad Integer(1:w169) -> (0:w166:i64)
  n32 = local read "Sets to FIFO (Traps)"() -> (w202:T10)
  n33 = local read "# Samples/channel"() -> (w159:u32)
  n34 = local read "Number of F/B Scans (AOD)"() -> (w160:u16)
  n35 = local read "Not-Interlacing Set"() -> (w39:enum32{"Set 1", "Set 2", "Set 3"})
  n36 = To Unsigned Byte Integer(number=w39) -> (unsigned 8bit integer=w45:u8)
  n37 = Index Array(array=w47, index=w45) -> (element=w46:u32)
  n38 = Divide(x=40000000.0, y="AI Count (ticks)") -> (x/y=w127:dbl)
  n39 = Multiply(x=w142, y=32767.0) -> (x*y=w144:dbl)
  n40 = local read "Feedback On/Off"() -> (w198:cluster{"Set 1":bool, "Set 2":bool})
  n41 = local read "PID Gains"() -> (w190:T8)
  n42 = local read "Scan steps (AOD)"() -> (w165:u64)
  n43 = local read "All FB On/Off"() -> (w199:bool)
  n44 = local write "AI rate (Hz)"(w127) -> ()
  n45 = local read "Cycles/step (AOD)"() -> (w164:u64)
  n46 = Divide(x=w144, y=10.0) -> (x/y=w143:dbl)
  n47 = Multiply(x=w165, y=w164) -> (x*y=w163:u64)
  n48 = Multiply(x=3276.7, y=w195) -> (x*y=w194:cluster{"Set 1":dbl, "Set 2":dbl})
  n49 = To Word Integer(number=w143) -> (16bit integer=w141:i16)
  n50 = Multiply(x=w163, y=u64 2) -> (x*y=w161:u64)
  n51 = Divide(x=w127, y="FPGA Ave.") -> (x/y=w128:dbl)
  n52 = To Word Integer(number=w194) -> (16bit integer=w193:cluster{"Set 1":i16, "Set 2":i16})
  n53 = xnode "Open FPGA VI Reference"("resource name"=T12 "750kHzDAQ") -> ("FPGA VI Reference Out"=w182:T13, "error out"=w181:errorcluster)  [unwired: 1 in]
  n54 = Unbundle By Name(w190) -> ("Set 1"=w189:T9, "Set 2"=w188:T9)
  n55 = Multiply(x=w161, y=w160) -> (x*y=w158:u64)
  n56 = Divide(x=w158, y=w159) -> (x/y=w157:dbl)
  n57 = Unbundle By Name(w193) -> ("Set 1"=w192:i16, "Set 2"=w191:i16)
  n58 = local write "Ave. Rate (Hz)"(w128) -> ()
  n59 = And(x=w198, y=w199) -> (x .and. y?=w197:cluster{"Set 1":bool, "Set 2":bool})
  n60 = local read "2D or 1D Scan"() -> (w68:bool)
  n61 = local write "Data points/scans"(w158) -> ()
  n62 = local read "Scan BD"() -> (w176:bool)
  n63 = Reciprocal(x=w128) -> (1/x=w129:dbl)
  n64 = local write "Data points/scan (f/b)"(w161) -> ()
  n65 = local write "N sets should be saved"(w157) -> ()
  n66 = local read "N Acq Sets (Traps)"() -> (w120:i16)
  n67 = Unbundle By Name(w197) -> ("Set 1"=w201:bool, "Set 2"=w200:bool)
  n68 = xnode "Invoke Method"("FPGA VI Reference In"=w182, "error in"=w181) -> ("FPGA VI Reference Out"=w64:T13, "error out"=w94:errorcluster)
  n69 = local read "Interlace"() -> (w41:bool)
  n70 = Select(t=w48, s=w41, f=w46) -> (s? t:f=w38:u32)
  n71 = local write "Update Count (MCL)"(w38) -> ()
  n72 = local write "Total Counts (ticks)"(w38) -> ()
  n73 = local write "Ave. Period (s)"(w129) -> ()
  n74 = property on="2D or 1D Scan" class="Bool (strict)"("Val(Sgnl)"=w68) -> ()  [unwired: 2 in, 2 out]
  n75 = xnode "Read/Write Control"("FPGA VI Reference In"=w63, "error in"=w94, "ai count"="AI Count (ticks)", "AI Averages"="FPGA Ave.", "DMA buffer timeout"=0, "AI to FIFO"=FALSE, "Interlace ON/OFF"=w41, "Number Interlace Cycles"=w40, "AI1 Sets to FIFO"=w202, "FB On/Off Set 1"=w201, "FB On/Off Set 2"=w200, "Interlace Off Parameters"=w39, "FB Setpoint Set 1"=w192, "FB Setpoint Set 2"=w191, "FB Gains Set 1"=w189, "FB Gains Set 2"=w188, "FB output range 1"=w65, "FB output range 2"=w65, "Cycles per step"=w164, "Scan BD"=w176, "Number of scans"=w160, "Scan steps"=w165, "Scan freq.  increment"=w166, "AO1"=w148, "AO2"=w147, "Scan freq.  increment (MCL)"=w141, "Scan steps (MCL)"=w140, "Cycles per step (MCL)"=w139, "Number of scans (MCL)"=w138, "MCL count"=w38, "Cont. Scan (MCL)"=w137, "MCL Scan Axis"=w131, "1D or 2D Scan?"=w68, "N of AI1 Int Acq Sets"=w120, "Freq or Amp switch first"="Freq or Amp switch first", "Freq switch delay"="Freq switch delay", "Amp switch delay"="Amp switch delay", "Swap F1 and F2"="Swap F1 and F2", "APD Acq Rate Count"=w78, "APD to FIFO"=FALSE, "APD Gate Operating Mode"="APD Gate", "APD Gate ON Count"="APD Gate ON Count", "APD Gate OFF Count"="APD Gate OFF Count", "Invert APD Gate"="Invert APD Gate", "DIO count 1 (ticks)"="DIO count 1 (ticks)", "DIO count 2 (ticks)"="DIO count 2 (ticks)", "DIO count 3 (ticks)"="DIO count 3 (ticks)", "APD 1 AO scale factor"="APD 1 AO Mult.", "APD 2 AO scale factor"="APD 2 AO Mult.", "APD 1 AO offset"="APD 1 AO offset", "APD 2 AO offset"="APD 2 AO offset") -> ("FPGA VI Reference Out"=w33:T13, "error out"=w35:errorcluster)
  n76 = local read "Green Laser ON/Interlacing"() -> (w36:bool)
  n77 = local read "GI Frequency, OFF count"() -> (w29:u32)
  n78 = Multiply(x="Current When FB OFF (%)", y=655.35) -> (x*y=w19:dbl)
  n79 = local read "GI Frequency, ON count"() -> (w28:u32)
  n80 = local read "Green laser mode"() -> (w37:enum32{"Laser ON", "Laser OFF", "Interlace"})
  n81 = local read "Green FB Count"() -> (w27:u32)
  n82 = To Unsigned Word Integer(number=w19) -> (unsigned 16bit integer=w17:u16)
  n83 = local read "Invert GI"() -> (w31:bool)
  n84 = Multiply(x="Green FB Setpoint (mV)", y=3.2767) -> (x*y=w16:dbl)
  n85 = case shown="False" w36 {
    tunnel: w37 -> [_ w229]
    tunnel: [enum32{"Laser ON", "Laser OFF", "Interlace"}."Laser OFF" ("Green laser mode") w229] -> w30
    frame #0 {
    }
    frame #1 {
    }
  }
  n86 = To Word Integer(number=w16) -> (16bit integer=w14:i16)
  n87 = xnode "Read/Write Control"("FPGA VI Reference In"=w33, "error in"=w35, "Green interlace ON count 2"=w28, "Green interlace OFF count 2"=w29, "Invert GI 2"=w31, "Operating Mode 2"=w30, "Green FB Gains"="Green FB Gains", "Green FB Setpoint"=w14, "Green FB On/Off"="Green FB On/Off", "Current Out"=w17, "Green int current ON count adj"="Green int current ON count adj", "Green FB Count"=w27, "Operating Mode"=w30, "Green interlace OFF count"=w29, "Green interlace ON count"=w28, "Invert GI"=w31) -> ("FPGA VI Reference Out"=w32:T13, "error out"=w34:errorcluster)
  n88 = flat-sequence {
    tunnel: w64 -> [w234]
    tunnel: [w234] -> w63
    tunnel: [w233] -> w62
    tunnel: [w232] -> w61
    tunnel: [w230] -> w59
    tunnel: [w231] -> w60
    frame #0 {
      w231 = T11 {"Minimum"=0.0, "Maximum"=40.0, "Increment"=1.0} ("Min Max Inc")
      w230 = T11 {"Minimum"=0.0, "Maximum"=50.0, "Increment"=1.0} ("Data Entry Limits")
      w233 = T11 {"Minimum"=60.0, "Maximum"=90.0, "Increment"=1.0} ("Min Max Inc")
      w232 = T11 {"Minimum"=0.0, "Maximum"=50.0, "Increment"=1.0} ("Data Entry Limits")
      n89 = property on="BD 2 Frequency 1 (MHz)" class="DigNum (strict)"("Data Range"=w231) -> ()  [unwired: 2 in, 2 out]
      n90 = property on="BD 2 Frequency 3 (MHz)" class="DigNum (strict)"("Data Range"=w231) -> ()  [unwired: 2 in, 2 out]
      n91 = property on="BD 2 Frequency 2 (MHz)" class="DigNum (strict)"("Data Range"=w231) -> ()  [unwired: 2 in, 2 out]
      n92 = property on="BD 1 Frequency 1 (MHz)" class="DigNum (strict)"("Data Range"=w233) -> ()  [unwired: 2 in, 2 out]
      n93 = property on="BD 1 Frequency 2 (MHz)" class="DigNum (strict)"("Data Range"=w233) -> ()  [unwired: 2 in, 2 out]
      n94 = property on="BD 1 Frequency 3 (MHz)" class="DigNum (strict)"("Data Range"=w233) -> ()  [unwired: 2 in, 2 out]
      n95 = property on="BD 2 Amplitude 1 (%)" class="DigNum (strict)"("Data Range"=w230) -> ()  [unwired: 2 in, 2 out]
      n96 = property on="BD 2 Amplitude 2 (%)" class="DigNum (strict)"("Data Range"=w230) -> ()  [unwired: 2 in, 2 out]
      n97 = property on="BD 2 Amplitude 3 (%)" class="DigNum (strict)"("Data Range"=w230) -> ()  [unwired: 2 in, 2 out]
      n98 = property on="BD 1 Amplitude 3 (%)" class="DigNum (strict)"("Data Range"=w232) -> ()  [unwired: 2 in, 2 out]
      n99 = property on="BD 1 Amplitude 2 (%)" class="DigNum (strict)"("Data Range"=w232) -> ()  [unwired: 2 in, 2 out]
      n100 = property on="BD 1 Amplitude 1 (%)" class="DigNum (strict)"("Data Range"=w232) -> ()  [unwired: 2 in, 2 out]
      "X RF Frequency Limits (MHz)" <- w233
      "X RF Amplitude Limits (%)" <- w232
      "Y RF Amplitude Limits (%)" <- w230
      "Y RF Frequency Limits (MHz)" <- w231
    }
  }
  n101 = xnode "Invoke Method"("FPGA VI Reference In"=w32, "error in"=w34, "Depth"="FIFO Depth") -> ("FPGA VI Reference Out"=w187:T13, "error out"=w186:errorcluster)
  n102 = xnode "Invoke Method"("FPGA VI Reference In"=w187, "error in"=w186) -> ("FPGA VI Reference Out"=w93:T13, "error out"=w92:errorcluster)
  n103 = xnode "Invoke Method"("FPGA VI Reference In"=w93, "error in"=w92) -> ("FPGA VI Reference Out"=w91:T13, "error out"=w90:errorcluster)  [unwired: 1 out]
  n104 = flat-sequence "Initial FPGA Loop Relative Phase Adjustment" {
    tunnel: "Initial Phase Adjustment (AI1)" -> [w244]
    tunnel: "Initial Phase Adjustment (GI)" -> [w243]
    tunnel: w91 -> [w242]
    tunnel: w90 -> [w241]
    tunnel: "Initial Phase Adj. (MCL)" -> [w240]
    tunnel: [w245] -> w102
    tunnel: [w239] -> w98
    tunnel: "Initial Phase Adjustment (APD Acq)" -> [w238]
    tunnel: "Initial Phase Adjustment (APD Gate)" -> [w237]
    tunnel: "Initial Phase Adjustment (Green FB)" -> [w236]
    tunnel: "Initial Phase Adjustment (GI) 2" -> [w235]
    tunnel: w102 -> [w397]
    tunnel: [w398] -> w99
    tunnel: w98 -> [w398]
    tunnel: [w397] -> w97
    tunnel: w99 -> [w401]
    tunnel: w97 -> [w400]
    tunnel: [w403] -> w96
    tunnel: [w402] -> w95
    tunnel: [w562] -> w100
    tunnel: [w563] -> w101
    tunnel: w96 -> [w563]
    tunnel: w95 -> [w562]
    frame #0 {
      n105 = xnode "Read/Write Control"("FPGA VI Reference In"=w242, "error in"=w241, "Phase count adjustment"=w244, "Phase count adjustment (GI)"=w243, "Phase count adjustment (MCL)"=w240, "Phase Count Adjustment (APD Acq)"=w238, "Phase count adjustment (APD Gate)"=w237, "Phase count adjustment (Green FB)"=w236, "Phase count adjustment (GI) 2"=w235) -> ("FPGA VI Reference Out"=w239:T13, "error out"=w245:errorcluster)
    }
    frame #1 {
      n106 = Wait (ms)(milliseconds to wait=u32 1000) -> ()  [unwired: 1 out]
    }
    frame #2 {
      w399 = TRUE
      n107 = xnode "Read/Write Control"("FPGA VI Reference In"=w401, "error in"=w400, "+ phase"=w399, "+ phase (GI)"=w399, "+ phase (MCL)"=w399, "+ phase (APD Acq)"=w399, "+ phase (APD Gate)"=w399, "+ phase (Green FB)"=w399, "+ phase (GI) 2"=w399) -> ("FPGA VI Reference Out"=w402:T13, "error out"=w403:errorcluster)
    }
    frame #3 {
      n108 = Wait (ms)(milliseconds to wait=u32 1000) -> ()  [unwired: 1 out]
    }
  }
  n109 = local read "Phase adj. (Green FB)"() -> (w50:i16)
  n110 = local read "Phase adj. (GI) 2"() -> (w20:i16)
  n111 = local read "Phase adj. (AI1)"() -> (w134:i16)
  n112 = local read "Phase adj. (GI)"() -> (w133:i16)
  n113 = local read "Phase adjust (MCL)"() -> (w132:i16)
  n114 = xnode "Read/Write Control"("FPGA VI Reference In"=w100, "error in"=w101, "Phase count adjustment"=w134, "Phase count adjustment (GI)"=w133, "Phase count adjustment (MCL)"=w132, "Phase Count Adjustment (APD Acq)"="Phase Adj. (APD Acq)", "Phase count adjustment (APD Gate)"="Phase Adj. (APD Gate)", "Phase count adjustment (Green FB)"=w50, "Phase count adjustment (GI) 2"=w20) -> ("FPGA VI Reference Out"=w1:T13, "error out"=w109:errorcluster)
  n115 = call "Initialize RF boards - interlace 3.vi"("error in"=w109, "FPGA VI Reference In"=w1) -> ("error out"=w107:errorcluster, "FPGA VI Reference Out"=w108:T13)
  n116 = call "set RF board frequency - interlace.vi"("Board 2 Frequency Limits"=w60, "Board 1 Frequency Limits"=w62, "error in"=w107, "FPGA VI Reference In"=w108, "Board 2 Frequency 3 (MHz)"="BD 2 Frequency 3 (MHz)", "Board 1 Frequency 3 (MHz)"="BD 1 Frequency 3 (MHz)", "Board 2 Frequency 2 (MHz)"="BD 2 Frequency 2 (MHz)", "Board 2 Frequency 1 (MHz)"="BD 2 Frequency 1 (MHz)", "Board 1 Frequency 2 (MHz)"="BD 1 Frequency 2 (MHz)", "Board 1 Frequency 1  (MHz)"="BD 1 Frequency 1 (MHz)") -> ("error out"=w218:errorcluster, "FPGA VI Reference Out"=w219:T13)
  n117 = call "set RF board amplitude - interlace.vi"("Board 2 Amplitude Limits"=w59, "Board 1 Amplitude Limits"=w61, "error in"=w218, "FPGA VI Reference In"=w219, "Board 2 Amplitude 3 (%)"="BD 2 Amplitude 3 (%)", "Board 1 Amplitude 3 (%)"="BD 1 Amplitude 3 (%)", "Board 2 Amplitude 2 (%)"="BD 2 Amplitude 2 (%)", "Board 2 Amplitude 1 (%)"="BD 2 Amplitude 1 (%)", "Board 1 Amplitude 2 (%)"="BD 1 Amplitude 2 (%)", "Board 1 Amplitude 1 (%)"="BD 1 Amplitude 1 (%)") -> ("error out"=w206:errorcluster, "FPGA VI Reference Out"=w207:T13)
  n118 = flat-sequence {
    tunnel: w207 -> [w572]
    tunnel: w206 -> [w571]
    tunnel: [w570] -> w211
    tunnel: [w569] -> w210
    tunnel: [w613] -> w209
    tunnel: w211 -> [w613]
    tunnel: [w612] -> w208
    tunnel: w210 -> [w612]
    tunnel: w209 -> [w621]
    tunnel: w208 -> [w620]
    tunnel: [w619] -> w73
    tunnel: [w618] -> w72
    frame #0 {
      n119 = local read "Trap 1 (ON/OFF)"() -> (w564:bool)
      n120 = xnode "Read/Write Control"("FPGA VI Reference In"=w572, "error in"=w571, "Direct RF Box  Communication"=FALSE) -> ("FPGA VI Reference Out"=w570:T13, "error out"=w569:errorcluster)
      n121 = local write "Saving..."(FALSE ("Saving Data")) -> ()
      n122 = local write "Stop All"(FALSE ("Stop All")) -> ()
      n123 = local write "Index"(1.0 ("Index")) -> ()
      n124 = property on="Trap 1 ON" class="Bool (strict)"("Value"=w564) -> ()  [unwired: 2 in, 2 out]
      "Manipulating Trap" <- FALSE ("Manipulating Trap")
    }
    frame #1 {
      n125 = local read "Trap 2 (ON/OFF)"() -> (w611:bool)
      n126 = Wait (ms)(milliseconds to wait=u32 10) -> ()  [unwired: 1 out]
      n127 = property on="Trap 2 ON" class="Bool (strict)"("Val(Sgnl)"=w611) -> ()  [unwired: 2 in, 2 out]
    }
    frame #2 {
      n128 = xnode "Read/Write Control"("FPGA VI Reference In"=w621, "error in"=w620, "FPGA Controls  RF Box"=TRUE ("Direct RF Box  Communication")) -> ("FPGA VI Reference Out"=w619:T13, "error out"=w618:errorcluster)
      n129 = call "Update messages.vi"("Message to add"="UHR-Fleezers ready.", "Old message string"="") -> ("New message string"=w617:string)
      n130 = local write "Messages"(w617) -> ()
    }
  }
  n131 = Subtract(x="BD 1 Frequency 1 (MHz)", y="BD 1 Frequency 2 (MHz)") -> (x-y=w119:dbl)
  n132 = Subtract(x="BD 2 Frequency 1 (MHz)", y="BD 2 Frequency 2 (MHz)") -> (x-y=w118:dbl)
  n133 = Square(x=w118) -> (x^2=w116:dbl)
  n134 = Square(x=w119) -> (x^2=w117:dbl)
  n135 = Add(x=w117, y=w116) -> (x+y=w115:dbl)
  n136 = Square Root(x=w115) -> (sqrt(x)=w114:dbl)
  n137 = local write "Trap Delta (MHz)"(w114) -> ()
  n138 = xnode "Read/Write Control"("FPGA VI Reference In"=w73, "error in"=w72, "AI to FIFO"=w71, "APD to FIFO"=w71) -> ("FPGA VI Reference Out"=w70:T13, "error out"=w69:errorcluster)
  n139 = node-c288() -> (w8:T16)  [unwired: 4 out]
  n140 = call-poly "VISA Configure Serial Port"("VISA resource name"="Sample Chamber Stage Serial Port") -> ("VISA resource name out"=w56:refnum<visa-resource-name>, "error out"=w55:errorcluster)  [unwired: 5 in, 8 out]
  n141 = timed-loop "Control parameters (event loop)" {
    tunnel: w73 -> [w663]
    shift-right: [w662] -> _
    shift-left: errorcluster {"status"=FALSE, "code"=0, "source"=""} ("error out") -> [w661]
    tunnel: [w660] -> w177
    timing: w8 -> [_]
    timing-out: [_] -> w7
    stop <- w660 stop-if-true
    n142 = node-c288() -> ()  [unwired: 2 out]
    n143 = event shown="[31] \"Number of F/B Scans (AOD)\", \"Scan Speed (nm/s)\", \"Scan BD\", \"Initial delta (MHz)\", \"Step Size (nm)\", \"Scan Range (nm)\": Value Change" {
      selector: _ -> [_ _ _ _ _ _ _ _ _ _ _ _ _ _ _ _ _ _ _ _ _ _ _ _ _ _ _ _ _ _ _ _ _ _ _ _ _ _ _ _ _ _ _ _ _]
      dyn-events: _ -> [_ _ _ _ _ _ _ _ _ _ _ _ _ _ _ _ _ _ _ _ _ _ _ _ _ _ _ _ _ _ _ _ _ _ _ _ _ _ _ _ _ _ _ _ _]
      timeout: _ -> [_ _ _ _ _ _ _ _ _ _ _ _ _ _ _ _ _ _ _ _ _ _ _ _ _ _ _ _ _ _ _ _ _ _ _ _ _ _ _ _ _ _ _ _ _]
      tunnel: w663 -> [w704 _ _ w831 _ w926 _ _ _ _ w992 _ _ _ _ _ _ w1108 w1246 w1308 w1351 w1501 w1576 w1687 w1780 w1864 w1948 w2032 w2116 w2209 w2404 w2604 w2697 w2827 _ w2997 w3038 w3085 w3162 w3203 _ w3248 _ _ _]
      tunnel: [w703 _ _ w821 _ w925 _ _ w957 _ w971 _ _ _ _ _ _ w1107 w1242 w1305 w1348 w1500 w1574 w1686 w1774 w1858 w1942 w2026 w2110 w2207 w2403 w2602 w2695 w2825 _ w2995 w3036 w3075 w3160 w3201 _ w3246 _ _ _] -> w662
      tunnel: w661 -> [w702 _ _ w830 _ w924 _ _ w957 _ w991 _ _ _ _ _ _ w1106 w1241 w1304 w1347 w1499 w1575 w1685 w1779 w1863 w1947 w2031 w2115 w2208 w2402 w2603 w2696 w2826 _ w2996 w3037 w3084 w3161 w3202 _ w3247 _ _ _]
      tunnel: [_ _ _ _ _ _ _ _ w956 _ _ _ _ _ _ _ _ _ _ _ _ _ _ _ _ _ _ _ _ _ _ _ _ _ _ _ _ _ _ _ _ _ _ _ _] -> w660
      tunnel: [_ _ _ _ _ _ "Round T1 X" _ _ _ _ _ _ _ _ "Load parameters" _ _ _ _ _ _ _ _ _ _ _ _ _ _ _ _ _ _ _ _ _ _ _ _ _ _ _ _ _] -> _
      tunnel: [_ _ "Adjust Scale\nto Mean" _ _ _ _ _ _ _ _ "Set Position 1" "Set Position 2" "Set Position 3" "Set Position 4" _ _ _ _ _ _ _ _ _ _ _ _ _ _ _ _ _ _ _ _ _ _ _ _ _ _ _ _ _ _] -> _
      tunnel: [_ _ _ _ _ _ _ "Round T2 X" _ "Delayed Interlace Start" _ _ _ _ _ _ _ _ _ _ _ _ _ _ _ _ _ _ _ _ _ _ _ _ _ _ _ _ _ _ _ _ _ _ _] -> _
      tunnel: [_ "Rescale on Mean" _ _ _ _ _ _ _ _ _ _ _ _ _ _ _ _ _ _ _ _ _ _ _ _ _ _ _ _ _ _ _ _ _ _ _ _ _ _ _ _ _ _ _] -> _
      event #0 {
        # "So that if 'Save ave N' is updated, the AOD scanning code updates too."
        n144 = event-data() -> ()  [unwired: 6 out]
        n145 = local read "AI Count (ticks)"() -> (w674:u32)
        n146 = local read "FPGA Ave."() -> (w678:dbl)
        n147 = Boolean To (0,1)(Boolean="Sets to FIFO (Traps)") -> (0, 1=w692:cluster{"Set 1":i16, "Set 2":i16, "Set 3":i16})
        n148 = xnode "Read/Write Control"("FPGA VI Reference In"=w704, "error in"=w702, "ai count"=w674, "AI1 Sets to FIFO"="Sets to FIFO (Traps)", "AI Averages"=w678, "N of AI1 Int Acq Sets"="N Acq Sets (Traps)") -> ("error out"=w703:errorcluster)  [unwired: 1 out]
        n149 = Cluster To Array(cluster=w692) -> (array=w691:i16[])
        n150 = local read "Scan steps (AOD)"() -> (w693:u64)
        n151 = Multiply(x=w674, y="N Acq Sets (Traps)") -> (x*y=w672:u32)
        n152 = Divide(x=40000000.0, y=w674) -> (x/y=w700:dbl)
        "AI rate (Hz)" <- w700
        n153 = Add Array Elements(numeric array=w691) -> (sum=w676:i16)
        "Trap Sets" <- w676
        n154 = Divide(x=w700, y=w678) -> (x/y=w701:dbl)
        "Ave. Rate (Hz)" <- w701
        n155 = Reciprocal(x=w701) -> (1/x=→"Ave. Period (s)":dbl)
        n156 = property on="Scan steps (AOD)" class="DigNum (strict)"("Val(Sgnl)"=w693) -> ()  [unwired: 2 in, 2 out]
        n157 = Divide(x=w701, y="N Acq Sets (Traps)") -> (x/y=w697:dbl)
        "Data Rate (Hz)" <- w697
        n158 = Reciprocal(x=w697) -> (1/x=→"Data Period (s)":dbl)
        n159 = local read "Save ave N"() -> (w696:dbl)
        n160 = Divide(x=w697, y=w696) -> (x/y=w695:dbl)
        "Save Data Rate (Hz)" <- w695
        n161 = Reciprocal(x=w695) -> (1/x=→"Save Data Period (s)":dbl)
        n162 = Multiply(x=w672, y="# Samples/trap") -> (x*y=w668:dbl)
        "Counts/DMA" <- w668
        n163 = Multiply(x=w676, y="# Samples/trap") -> (x*y=w675:dbl)
        "# Samples/channel" <- w675
        n164 = Greater?(x=w678, y=1.0) -> (0:w681:bool)
        "FPGA Averaging" <- w681
        n165 = local read "APD Int. Count"() -> (w670:u32)
        n166 = Divide(x=w675, y=u32 2) -> (x/y=w684:dbl)
        n167 = Select(t=w675, s=w681, f=w684) -> (s? t:f=w689:dbl)
        n168 = Divide(x=w668, y=w670) -> (x/y=w669:dbl)
        "APD Samples/FIFO Acq." <- w669
        n169 = Divide(x=w668, y=40000000.0) -> (x/y=w666:dbl)
        "DMA Update Period (s)" <- w666
        n170 = Multiply(x=w689, y=u32 8) -> (x*y=→"Elements/DMA read":dbl)
        n171 = Multiply(x=2.0, y=w669) -> (x*y=→"APD Elements/DMA read":dbl)
        n172 = local read "N sets to save"() -> (w686:u32)
        n173 = Multiply(x=w666, y=w686) -> (x*y=→"Total Time (s)":dbl)
      }
      event #1 {
        n174 = event-data() -> ()  [unwired: 7 out]
        n175 = local read "Bead Mean (nm)"() -> (w809:dbl)
        n176 = Add(x="Amplitude (nm)", y=w809) -> (x+y=w807:dbl)
        n177 = Subtract(x=w809, y="Amplitude (nm)") -> (x-y=w806:dbl)
        n178 = property on="Bead Separation" class="WFChart (strict)"("YScale.Maximum"=w807) -> ()  [unwired: 2 in, 2 out]
        n179 = property on="Bead Separation" class="WFChart (strict)"("YScale.Minimum"=w806) -> ()  [unwired: 2 in, 2 out]
      }
      event #2 {
        n180 = event-data() -> ()  [unwired: 7 out]
        n181 = local read "APD 1 Rate (Hz)"() -> (w818:dbl)
        n182 = Multiply(x=1000.0, y="Above (kHz)") -> (x*y=w816:dbl)
        n183 = Multiply(x=1000.0, y="Below (kHz)") -> (x*y=w814:dbl)
        n184 = Add(x=w816, y=w818) -> (x+y=w811:dbl)
        n185 = Subtract(x=w818, y=w814) -> (x-y=w812:dbl)
        n186 = property on="APD 1 Chart" class="WFChart (strict)"("YScale.Maximum"=w811) -> ()  [unwired: 2 in, 2 out]
        n187 = property on="APD 1 Chart" class="WFChart (strict)"("YScale.Minimum"=w812) -> ()  [unwired: 2 in, 2 out]
      }
      event #3 {
        n188 = event-data() -> ()  [unwired: 7 out]
        n189 = Negate(x="Phase adj. (AI1)") -> (-x=w828:i16)
        n190 = Select(t=w828, s="- phase (AI1)", f="Phase adj. (AI1)") -> (s? t:f=w827:i16)
        n191 = xnode "Read/Write Control"("FPGA VI Reference In"=w831, "error in"=w830, "Phase count adjustment"=w827) -> ("FPGA VI Reference Out"=w826:T13, "error out"=w825:errorcluster)
        n192 = Or(x="- phase (AI1)", y="+ phase (AI1)") -> (x .or. y?=w822:bool)
        n193 = xnode "Read/Write Control"("FPGA VI Reference In"=w826, "error in"=w825, "+ phase"=w822) -> ("error out"=w821:errorcluster)  [unwired: 1 out]
      }
      event #4 {
        w907 = u32 9868950 ("Color Box")
        n194 = event-data() -> ("Row"=w909:i32)  [unwired: 9 out]
        n195 = property on="All Signals" class="WFChart (strict)"("Active Plot"=w909) -> (error out=w920:errorcluster)  [unwired: 2 in, 1 out]
        n196 = property on="All Signals" class="WFChart (strict)" props=["Plot", "Visible?", "Plot", "Plot Color"](error in=w920) -> (error out=w919:errorcluster, "Plot.Visible?"=w918:bool)  [unwired: 1 in, 2 out]
        n197 = Select(t=FALSE ("Plot.Visible"), s=w918, f=TRUE ("Plot.Visible")) -> (s? t:f=w913:bool)
        n198 = property on="All Signals" class="WFChart (strict)"(error in=w919, "Plot.Visible?"=w913) -> (error out=w915:errorcluster)  [unwired: 1 in, 1 out]
        n199 = property on="All Signals" class="WFChart (strict)"(error in=w915) -> (error out=w910:errorcluster, "Plot.Plot Color"=w914:u32)  [unwired: 1 in, 1 out]
        n200 = property on="Signals to Plot" class="LstBox (strict)"(error in=w910, "Active Row"=w909) -> (error out=w908:errorcluster)  [unwired: 1 in, 1 out]
        n201 = Select(t=w914, s=w913, f=u32 0) -> (s? t:f=w911:u32)
        n202 = property on="Signals to Plot" class="LstBox (strict)"(error in=w908, "CellFontColor"=w911, "SelColor"=w907, "CellBG"=w907, "CellFontSize"=u32 20 ("Active Row:Cell Font:Size"), "CellFontBold"=TRUE ("Active Row:Cell Font:Bold")) -> ()  [unwired: 1 in, 2 out]
      }
      event #5 {
        n203 = event-data() -> ("CtlRef"=w923:refnum<vi>)  [unwired: 6 out]
        n204 = control-ref of="Trap Delta (MHz)"() -> (w922:refnum<vi>)
        n205 = Equal?(x=w922, y=w923) -> (x = y?=w921:bool)
        n206 = case shown="False" "Oscillate Set 1" {
          tunnel: w926 -> [w946 _]
          tunnel: [w945 w949] -> w925
          tunnel: w924 -> [w944 w949]
          tunnel: w921 -> [w929 _]
          frame #0 {
            n207 = local read "BD 1 Frequency 2 (MHz)"() -> (w933:dbl)
            n208 = local read "BD 1 Frequency 1 (MHz)"() -> (w931:dbl)
            n209 = Subtract(x=w933, y="Trap Delta (MHz)") -> (x-y=w930:dbl)
            n210 = Select(t=w930, s=w929, f=w931) -> (s? t:f=w928:dbl)
            n211 = local read "Y RF Frequency Limits (MHz)"() -> (w934:T11)
            n212 = local read "X RF Frequency Limits (MHz)"() -> (w935:T11)
            n213 = local read "BD 1 Frequency 3 (MHz)"() -> (w947:dbl)
            n214 = local write "BD 1 Frequency 1 (MHz)"(w928) -> ()
            n215 = local read "BD 2 Frequency 1 (MHz)"() -> (w938:dbl)
            n216 = local read "BD 2 Frequency 2 (MHz)"() -> (w937:dbl)
            n217 = local read "BD 2 Frequency 3 (MHz)"() -> (w948:dbl)
            n218 = call "set RF board frequency - interlace.vi"("Board 2 Frequency Limits"=w934, "Board 1 Frequency Limits"=w935, "error in"=w944, "FPGA VI Reference In"=w946, "Board 2 Frequency 3 (MHz)"=w948, "Board 1 Frequency 3 (MHz)"=w947, "Board 2 Frequency 2 (MHz)"=w937, "Board 2 Frequency 1 (MHz)"=w938, "Board 1 Frequency 2 (MHz)"=w933, "Board 1 Frequency 1  (MHz)"=w928) -> ("error out"=w945:errorcluster)  [unwired: 1 out]
            n219 = Subtract(x=w938, y=w937) -> (x-y=w942:dbl)
            n220 = Subtract(x=w928, y=w933) -> (x-y=w943:dbl)
            n221 = Square(x=w942) -> (x^2=w940:dbl)
            n222 = Square(x=w943) -> (x^2=w941:dbl)
            n223 = Add(x=w941, y=w940) -> (x+y=w939:dbl)
            n224 = Square Root(x=w939) -> (sqrt(x)=w936:dbl)
            n225 = local write "Trap Delta (MHz)"(w936) -> ()
            n226 = property on="Initial delta (MHz)" class="DigNum (strict)"("Val(Sgnl)"=w936) -> ()  [unwired: 2 in, 2 out]
          }
          frame #1 {
          }
        }
      }
      event #6 {
        n227 = event-data() -> ()  [unwired: 7 out]
        n228 = local read "BD 1 Frequency 1 (MHz)"() -> (w952:dbl)
        n229 = Round To Nearest(number=w952) -> (nearest integer value=w951:dbl)
        n230 = property on="BD 1 Frequency 1 (MHz)" class="DigNum (strict)"("Val(Sgnl)"=w951) -> ()  [unwired: 2 in, 2 out]
      }
      event #7 {
        n231 = event-data() -> ()  [unwired: 7 out]
        n232 = local read "BD 1 Frequency 2 (MHz)"() -> (w954:dbl)
        n233 = Round To Nearest(number=w954) -> (nearest integer value=w953:dbl)
        n234 = property on="BD 1 Frequency 2 (MHz)" class="DigNum (strict)"("Val(Sgnl)"=w953) -> ()  [unwired: 2 in, 2 out]
      }
      event #8 {
        n235 = event-data() -> ()  [unwired: 7 out]
        n236 = local read "Stop All"() -> (w956:bool)
      }
      event #9 {
        n237 = event-data() -> ()  [unwired: 7 out]
        n238 = flat-sequence {
          frame #0 {
            n239 = Multiply(x="Delay to Interlace (s)", y=1000.0) -> (x*y=w959:dbl)
            n240 = Wait (ms)(milliseconds to wait=w959) -> ()  [unwired: 1 out]
          }
          frame #1 {
            n241 = property on="Green laser mode" class="RadioBtnsControl (strict)"("Val(Sgnl)"=enum32{"Laser ON", "Laser OFF", "Interlace"}."Interlace" ("Value (Signaling)")) -> ()  [unwired: 2 in, 2 out]
          }
        }
      }
      event #10 {
        w983 = i16 1 ("f")
        n242 = event-data() -> ()  [unwired: 7 out]
        n243 = local write "Trap 1 (ON/OFF)"("Trap 1 ON") -> ()
        n244 = local write "Trap 2 (ON/OFF)"("Trap 2 ON") -> ()
        n245 = Boolean To (0,1)(Boolean="Trap 3 ON") -> (0, 1=w984:i16)
        n246 = Boolean To (0,1)(Boolean="Trap 1 ON") -> (0, 1=w985:i16)
        n247 = Boolean To (0,1)(Boolean="Trap 2 ON") -> (0, 1=w986:i16)
        n248 = Select(t=w986, s="Trap ON/OFF X or Y Amp?", f=w983) -> (s? t:f=w981:i16)
        n249 = Select(t=w985, s="Trap ON/OFF X or Y Amp?", f=w983) -> (s? t:f=w982:i16)
        n250 = Select(t=w984, s="Trap ON/OFF X or Y Amp?", f=w983) -> (s? t:f=w980:i16)
        n251 = Select(t=w983, s="Trap ON/OFF X or Y Amp?", f=w986) -> (s? t:f=w978:i16)
        n252 = Select(t=w983, s="Trap ON/OFF X or Y Amp?", f=w985) -> (s? t:f=w979:i16)
        n253 = Select(t=w983, s="Trap ON/OFF X or Y Amp?", f=w984) -> (s? t:f=w977:i16)
        n254 = And(x="All FB On/Off", y="Feedback On/Off") -> (x .and. y?=w975:cluster{"Set 1":bool, "Set 2":bool})
        n255 = local read "BD 1 Amplitude 1 (%)"() -> (w995:dbl)
        n256 = local read "BD 1 Amplitude 2 (%)"() -> (w994:dbl)
        n257 = local read "BD 1 Amplitude 3 (%)"() -> (w993:dbl)
        n258 = Unbundle By Name(w975) -> ("Set 1"=w970:bool, "Set 2"=w967:bool)
        n259 = local read "Y RF Amplitude Limits (%)"() -> (w963:T11)
        n260 = local read "X RF Amplitude Limits (%)"() -> (w964:T11)
        n261 = local read "BD 2 Amplitude 1 (%)"() -> (w996:dbl)
        n262 = local read "BD 2 Amplitude 2 (%)"() -> (w997:dbl)
        n263 = local read "BD 2 Amplitude 3 (%)"() -> (w998:dbl)
        n264 = And(x="Trap 2 ON", y=w967) -> (x .and. y?=w965:bool)
        n265 = And(x="Trap 1 ON", y=w970) -> (x .and. y?=w968:bool)
        n266 = Multiply(x=w982, y=w995) -> (x*y=w990:dbl)
        n267 = Multiply(x=w994, y=w981) -> (x*y=w988:dbl)
        n268 = Multiply(x=w993, y=w980) -> (x*y=w989:dbl)
        n269 = Multiply(x=w996, y=w979) -> (x*y=w999:dbl)
        n270 = Multiply(x=w997, y=w978) -> (x*y=w1000:dbl)
        n271 = Multiply(x=w998, y=w977) -> (x*y=w1001:dbl)
        n272 = call "set RF board amplitude - interlace.vi"("Board 2 Amplitude Limits"=w963, "Board 1 Amplitude Limits"=w964, "error in"=w991, "FPGA VI Reference In"=w992, "Board 2 Amplitude 3 (%)"=w1001, "Board 1 Amplitude 3 (%)"=w989, "Board 2 Amplitude 2 (%)"=w1000, "Board 2 Amplitude 1 (%)"=w999, "Board 1 Amplitude 2 (%)"=w988, "Board 1 Amplitude 1 (%)"=w990) -> ("error out"=w972:errorcluster, "FPGA VI Reference Out"=w973:T13)
        n273 = xnode "Read/Write Control"("FPGA VI Reference In"=w973, "error in"=w972, "FB On/Off Set 1"=w968, "FB On/Off Set 2"=w965) -> ("error out"=w971:errorcluster)  [unwired: 1 out]
      }
      event #11 {
        n274 = event-data() -> ()  [unwired: 7 out]
        n275 = local read "Current Stage  Position"() -> (w1062:cluster{dbl, dbl, dbl})
        n276 = local read "Saved Stage Positions"() -> (w1061:T3)
        n277 = Bundle By Name(cluster=w1061, "Position 1"=w1062) -> (w1060:T3)
        n278 = local write "Saved Stage Positions"(w1060) -> ()
      }
      event #12 {
        n279 = event-data() -> ()  [unwired: 7 out]
        n280 = local read "Current Stage  Position"() -> (w1066:cluster{dbl, dbl, dbl})
        n281 = local read "Saved Stage Positions"() -> (w1065:T3)
        n282 = Bundle By Name(cluster=w1065, "Position 2"=w1066) -> (w1064:T3)
        n283 = local write "Saved Stage Positions"(w1064) -> ()
      }
      event #13 {
        n284 = event-data() -> ()  [unwired: 7 out]
        n285 = local read "Saved Stage Positions"() -> (w1070:T3)
        n286 = local read "Current Stage  Position"() -> (w1069:cluster{dbl, dbl, dbl})
        n287 = Bundle By Name(cluster=w1070, "Position 3"=w1069) -> (w1068:T3)
        n288 = local write "Saved Stage Positions"(w1068) -> ()
      }
      event #14 {
        n289 = event-data() -> ()  [unwired: 7 out]
        n290 = local read "Current Stage  Position"() -> (w1073:cluster{dbl, dbl, dbl})
        n291 = local read "Saved Stage Positions"() -> (w1074:T3)
        n292 = Bundle By Name(cluster=w1074, "Position 4"=w1073) -> (w1072:T3)
        n293 = local write "Saved Stage Positions"(w1072) -> ()
      }
      event #15 {
        n294 = event-data() -> ()  [unwired: 7 out]
        n295 = property on="Saved AOD Raster Scan Parameter Sets" class="Arr (strict)"() -> ("Index Values"=w1084:u32[])  [unwired: 2 in, 2 out]
        n296 = Index Array(array=w1084, index=0) -> (element=w1081:u32)
        n297 = Index Array(array="Saved AOD Raster Scan Parameter Sets", index=w1081) -> (element=w1080:T21)
        n298 = Unbundle By Name(w1080) -> ("Scan Range AOD (nm) 2"=w1079:dbl, "Step Size AOD (nm) 2"=w1078:dbl, "Scan Speed AOD (nm/s) 2"=w1077:dbl, "Number of scans (AOD) 2"=w1076:u16)
        n299 = flat-sequence {
          tunnel: w1079 -> [w1088]
          tunnel: w1078 -> [w1087]
          tunnel: w1077 -> [w1086]
          tunnel: w1076 -> [w1089]
          frame #0 {
            n300 = local write "Scan Speed (nm/s)"(w1086) -> ()
            n301 = local write "Scan Range (nm)"(w1088) -> ()
            n302 = local write "Step Size (nm)"(w1087) -> ()
          }
          frame #1 {
            n303 = property on="Number of F/B Scans (AOD)" class="DigNum (strict)"("Val(Sgnl)"=w1089) -> ()  [unwired: 2 in, 2 out]
          }
        }
      }
      event #16 {
        n304 = event-data() -> ()  [unwired: 7 out]
        n305 = property on="Trap 2 ON" class="Bool (strict)"("Val(Sgnl)"="Trap 2 (ON/OFF)") -> ()  [unwired: 2 in, 2 out]
        n306 = property on="Trap 1 ON" class="Bool (strict)"("Val(Sgnl)"="Trap 1 (ON/OFF)") -> ()  [unwired: 2 in, 2 out]
      }
      event #17 {
        n307 = event-data() -> ()  [unwired: 7 out]
        n308 = local read "DIO count 3 (ticks)"() -> (w1102:u32)
        n309 = local read "DIO count 1 (ticks)"() -> (w1104:u32)
        n310 = local read "DIO count 2 (ticks)"() -> (w1103:u32)
        n311 = To Unsigned Byte Integer(number="Not-Interlacing Set") -> (unsigned 8bit integer=w1093:u8)
        n312 = Add(x=w1093, y=u8 1) -> (x+y=w1097:u8)
        n313 = xnode "Read/Write Control"("FPGA VI Reference In"=w1108, "error in"=w1106, "DIO count 1 (ticks)"=w1104, "DIO count 2 (ticks)"=w1103, "DIO count 3 (ticks)"=w1102, "Interlace ON/OFF"="Interlace", "Number Interlace Cycles"="Number Interlace Sets", "Interlace Off Parameters"=w1097) -> ("error out"=w1107:errorcluster)  [unwired: 1 out]
        n314 = Build Array(w1104, w1103, w1102) -> (w1095:u32[])
        n315 = Split 1D Array(array=w1095, index="Number Interlace Sets") -> (first subarray=w1105:u32[])  [unwired: 1 out]
        n316 = Index Array(array=w1095, index=w1093) -> (element=w1094:u32)
        n317 = Add Array Elements(numeric array=w1105) -> (sum=w1099:u32)
        n318 = Select(t=w1099, s="Interlace", f=w1094) -> (s? t:f=→"Total Counts (ticks)":u32)
      }
      event #18 {
        n319 = event-data() -> ()  [unwired: 7 out]
        n320 = Unbundle By Name("Reset Feedback") -> ("Set 1"=w1244:bool, "Set 2"=w1243:bool)
        n321 = xnode "Read/Write Control"("FPGA VI Reference In"=w1246, "error in"=w1241, "FB Reset Set 1"=w1244, "FB Reset Set 2"=w1243) -> ("error out"=w1242:errorcluster)  [unwired: 1 out]
      }
      event #19 {
        n322 = event-data() -> ()  [unwired: 7 out]
        n323 = Unbundle By Name("PID Gains") -> ("Set 1"=w1307:T9, "Set 2"=w1306:T9)
        n324 = xnode "Read/Write Control"("FPGA VI Reference In"=w1308, "error in"=w1304, "FB Gains Set 1"=w1307, "FB Gains Set 2"=w1306) -> ("error out"=w1305:errorcluster)  [unwired: 1 out]
      }
      event #20 {
        n325 = event-data() -> ()  [unwired: 7 out]
        n326 = xnode "Read/Write Control"("FPGA VI Reference In"=w1351, "error in"=w1347) -> ("FPGA VI Reference Out"=w1350:T13, "error out"=w1349:errorcluster, "AI2 Y Sum Set 1"=w1358:i16, "AI2 Y Sum Set 2"=w1357:i16)
        n327 = Cluster To Array(cluster="AI2 to Setpoint") -> (array=w1361:bool[])
        n328 = local read "AI2 (V)"() -> (w1359:cluster{"Set 1":dbl, "Set 2":dbl})
        n329 = Or Array Elements(Boolean array=w1361) -> (logical OR=w1362:bool)
        n330 = Bundle By Name(cluster=w1359, "Set 1"=w1358, "Set 2"=w1357) -> (w1356:cluster{"Set 1":dbl, "Set 2":dbl})
        n331 = Divide(x=w1356, y=3276.7) -> (x/y=w1355:cluster{"Set 1":dbl, "Set 2":dbl})
        "AI2 (V)" <- w1355
        n332 = case shown="True" w1362 {
          tunnel: [w1424 w1441] -> w1354
          tunnel: "AI2 to Setpoint" -> [_ w1437]
          tunnel: "Setpoints (V)" -> [w1425 w1440]
          tunnel: w1355 -> [_ w1434]
          frame #0 {
            n333 = Multiply(x=3276.7, y=w1425) -> (x*y=w1426:cluster{"Set 1":dbl, "Set 2":dbl})
            n334 = To Word Integer(number=w1426) -> (16bit integer=w1424:cluster{"Set 1":i16, "Set 2":i16})
          }
          frame #1 {
            n335 = Unbundle By Name(w1434) -> ("Set 1"=w1433:dbl, "Set 2"=w1432:dbl)
            n336 = Unbundle By Name(w1440) -> ("Set 1"=w1439:dbl, "Set 2"=w1438:dbl)
            n337 = Unbundle By Name(w1437) -> ("Set 1"=w1436:bool, "Set 2"=w1435:bool)
            n338 = Select(t=w1433, s=w1436, f=w1439) -> (s? t:f=w1431:dbl)
            n339 = Select(t=w1432, s=w1435, f=w1438) -> (s? t:f=w1430:dbl)
            n340 = Bundle By Name(cluster=w1440, "Set 1"=w1431, "Set 2"=w1430) -> (w1428:cluster{"Set 1":dbl, "Set 2":dbl})
            n341 = Multiply(x=3276.7, y=w1428) -> (x*y=w1429:cluster{"Set 1":dbl, "Set 2":dbl})
            n342 = local write "Setpoints (V)"(w1428) -> ()
            n343 = To Word Integer(number=w1429) -> (16bit integer=w1441:cluster{"Set 1":i16, "Set 2":i16})
          }
        }
        n344 = Unbundle By Name(w1354) -> ("Set 1"=w1353:i16, "Set 2"=w1352:i16)
        n345 = xnode "Read/Write Control"("FPGA VI Reference In"=w1350, "error in"=w1349, "FB Setpoint Set 1"=w1353, "FB Setpoint Set 2"=w1352) -> ("error out"=w1348:errorcluster)  [unwired: 1 out]
      }
      event #21 {
        n346 = event-data() -> ()  [unwired: 7 out]
        n347 = xnode "Read/Write Control"("FPGA VI Reference In"=w1501, "error in"=w1499, "Invert GI"="Invert GI", "Invert GI 2"="Invert GI") -> ("error out"=w1500:errorcluster)  [unwired: 1 out]
      }
      event #22 {
        n348 = event-data() -> ()  [unwired: 7 out]
        n349 = local read "Green FB Setpoint (mV)"() -> (w1565:dbl)
        n350 = local read "Current When FB OFF (%)"() -> (w1568:dbl)
        n351 = Multiply(x=w1565, y=3.2767) -> (x*y=w1564:dbl)
        n352 = Multiply(x=w1568, y=655.35) -> (x*y=w1569:dbl)
        n353 = To Unsigned Word Integer(number=w1569) -> (unsigned 16bit integer=w1567:u16)
        n354 = local read "Green int current ON count adj"() -> (w1572:u32)
        n355 = local read "Green FB Gains"() -> (w1571:T9)
        n356 = local read "Green Laser ON/Interlacing"() -> (w1562:bool)
        n357 = local read "Green laser mode"() -> (w1561:enum32{"Laser ON", "Laser OFF", "Interlace"})
        n358 = local read "Green FB On/Off"() -> (w1573:bool)
        n359 = Equal?(x=w1561, y=enum32{"Laser ON", "Laser OFF", "Interlace"}."Interlace") -> (x = y?=w1559:bool)
        n360 = Compound Arithmetic op=AND(w1559, w1573, w1562) -> (w1563:bool)
        n361 = xnode "Read/Write Control"("FPGA VI Reference In"=w1576, "error in"=w1575, "Green FB Setpoint"=w1564, "Green FB On/Off"=w1563, "Current Out"=w1567, "Green int current ON count adj"=w1572, "Green FB Gains"=w1571) -> ("error out"=w1574:errorcluster)  [unwired: 1 out]
      }
      event #23 {
        n362 = event-data() -> ()  [unwired: 7 out]
        n363 = case shown="True" "Green Laser ON/Interlacing" {
          tunnel: "Green laser mode" -> [_ w1694]
          tunnel: [enum32{"Laser ON", "Laser OFF", "Interlace"}."Laser OFF" ("Green laser mode") w1694] -> w1682
          tunnel: [FALSE w1690] -> w1681
          frame #0 {
          }
          frame #1 {
            n364 = local read "Green FB On/Off"() -> (w1691:bool)
            n365 = Equal?(x=w1694, y=enum32{"Laser ON", "Laser OFF", "Interlace"}."Interlace") -> (x = y?=w1692:bool)
            n366 = And(x=w1692, y=w1691) -> (x .and. y?=w1690:bool)
          }
        }
        n367 = xnode "Read/Write Control"("FPGA VI Reference In"=w1687, "error in"=w1685, "Operating Mode"=w1682, "Operating Mode 2"=w1682, "Green FB On/Off"=w1681) -> ("error out"=w1686:errorcluster)  [unwired: 1 out]
      }
      event #24 {
        n368 = event-data() -> ()  [unwired: 7 out]
        n369 = local read "Phase Adj. (APD Gate)"() -> (w1770:i16)
        n370 = Negate(x=w1770) -> (-x=w1778:i16)
        n371 = Select(t=w1778, s="- phase (APD Gate)", f=w1770) -> (s? t:f=w1777:i16)
        n372 = Or(x="- phase (APD Gate)", y="+ phase (APD Gate)") -> (x .or. y?=w1773:bool)
        n373 = xnode "Read/Write Control"("FPGA VI Reference In"=w1780, "error in"=w1779, "Phase count adjustment (APD Gate)"=w1777) -> ("FPGA VI Reference Out"=w1775:T13, "error out"=w1776:errorcluster)
        n374 = xnode "Read/Write Control"("FPGA VI Reference In"=w1775, "error in"=w1776, "+ phase (APD Gate)"=w1773) -> ("error out"=w1774:errorcluster)  [unwired: 1 out]
      }
      event #25 {
        n375 = event-data() -> ()  [unwired: 7 out]
        n376 = local read "Phase Adj. (APD Acq)"() -> (w1856:i16)
        n377 = Negate(x=w1856) -> (-x=w1862:i16)
        n378 = Select(t=w1862, s="+ phase (APD Acq)", f=w1856) -> (s? t:f=w1861:i16)
        n379 = Or(x="+ phase (APD Acq)", y="- phase (APD Acq)") -> (x .or. y?=w1857:bool)
        n380 = xnode "Read/Write Control"("FPGA VI Reference In"=w1864, "error in"=w1863, "Phase Count Adjustment (APD Acq)"=w1861) -> ("FPGA VI Reference Out"=w1859:T13, "error out"=w1860:errorcluster)
        n381 = xnode "Read/Write Control"("FPGA VI Reference In"=w1859, "error in"=w1860, "+ phase (APD Acq)"=w1857) -> ("error out"=w1858:errorcluster)  [unwired: 1 out]
      }
      event #26 {
        n382 = event-data() -> ()  [unwired: 7 out]
        n383 = Negate(x="Phase adj. (GI)") -> (-x=w1946:i16)
        n384 = Select(t=w1946, s="+ phase (GI)", f="Phase adj. (GI)") -> (s? t:f=w1945:i16)
        n385 = Or(x="+ phase (GI)", y="- phase (GI)") -> (x .or. y?=w1941:bool)
        n386 = xnode "Read/Write Control"("FPGA VI Reference In"=w1948, "error in"=w1947, "Phase count adjustment (GI)"=w1945) -> ("FPGA VI Reference Out"=w1943:T13, "error out"=w1944:errorcluster)
        n387 = xnode "Read/Write Control"("FPGA VI Reference In"=w1943, "error in"=w1944, "+ phase (GI)"=w1941) -> ("error out"=w1942:errorcluster)  [unwired: 1 out]
      }
      event #27 {
        n388 = event-data() -> ()  [unwired: 7 out]
        n389 = Negate(x="Phase adj. (GI) 2") -> (-x=w2030:i16)
        n390 = Select(t=w2030, s="+ phase (GI) 2", f="Phase adj. (GI) 2") -> (s? t:f=w2029:i16)
        n391 = Or(x="+ phase (GI) 2", y="- phase (GI) 2") -> (x .or. y?=w2025:bool)
        n392 = xnode "Read/Write Control"("FPGA VI Reference In"=w2032, "error in"=w2031, "Phase count adjustment (GI) 2"=w2029) -> ("FPGA VI Reference Out"=w2027:T13, "error out"=w2028:errorcluster)
        n393 = xnode "Read/Write Control"("FPGA VI Reference In"=w2027, "error in"=w2028, "+ phase (GI) 2"=w2025) -> ("error out"=w2026:errorcluster)  [unwired: 1 out]
      }
      event #28 {
        n394 = event-data() -> ()  [unwired: 7 out]
        n395 = Negate(x="Phase adj. (Green FB)") -> (-x=w2114:i16)
        n396 = Select(t=w2114, s="+ phase (Green FB)", f="Phase adj. (Green FB)") -> (s? t:f=w2113:i16)
        n397 = Or(x="+ phase (Green FB)", y="- phase (Green FB)") -> (x .or. y?=w2109:bool)
        n398 = xnode "Read/Write Control"("FPGA VI Reference In"=w2116, "error in"=w2115, "Phase count adjustment (Green FB)"=w2113) -> ("FPGA VI Reference Out"=w2111:T13, "error out"=w2112:errorcluster)
        n399 = xnode "Read/Write Control"("FPGA VI Reference In"=w2111, "error in"=w2112, "+ phase (Green FB)"=w2109) -> ("error out"=w2110:errorcluster)  [unwired: 1 out]
      }
      event #29 {
        n400 = event-data() -> ()  [unwired: 7 out]
        n401 = local read "Invert APD Gate"() -> (w2206:bool)
        n402 = local read "APD Gate ON Count"() -> (w2205:u32)
        n403 = local read "APD Gate OFF Count"() -> (w2204:u32)
        n404 = local read "APD Integration Time (s)"() -> (w2190:dbl)
        n405 = local read "APD Gate"() -> (w2203:enum32{"ON", "OFF", "Interlace"})
        n406 = Multiply(x=w2190, y=40000000.0) -> (x*y=w2201:dbl)
        n407 = Reciprocal(x=w2190) -> (1/x=→"APD Acq Rate (Hz)":dbl)
        n408 = To Unsigned Long Integer(number=w2201) -> (unsigned 32bit integer=w2200:u32)
        n409 = local read "DMA Update Period (s)"() -> (w2191:dbl)
        n410 = Divide(x=w2191, y=w2190) -> (x/y=w2194:dbl)
        n411 = local read "APD 1 AO offset"() -> (w2196:i16)
        n412 = local read "APD 2 AO offset"() -> (w2195:i16)
        n413 = local read "APD 1 AO Mult."() -> (w2198:i16)
        n414 = local read "APD 2 AO Mult."() -> (w2197:i16)
        n415 = Multiply(x=2.0, y=w2194) -> (x*y=w2193:dbl)
        n416 = local write "APD Samples/FIFO Acq."(w2194) -> ()
        n417 = local write "APD Elements/DMA read"(w2193) -> ()
        n418 = xnode "Read/Write Control"("FPGA VI Reference In"=w2209, "error in"=w2208, "Invert APD Gate"=w2206, "APD Gate ON Count"=w2205, "APD Gate OFF Count"=w2204, "APD Acq Rate Count"=w2200, "APD Gate Operating Mode"=w2203, "APD 1 AO scale factor"=w2198, "APD 2 AO scale factor"=w2197, "APD 1 AO offset"=w2196, "APD 2 AO offset"=w2195) -> ("error out"=w2207:errorcluster)  [unwired: 1 out]
      }
      event #30 {
        n419 = event-data() -> ()  [unwired: 7 out]
        n420 = xnode "Read/Write Control"("FPGA VI Reference In"=w2404, "error in"=w2402, "Green interlace ON count"="GI Frequency, ON count", "Green interlace OFF count"="GI Frequency, OFF count", "Green interlace ON count 2"="GI Frequency, ON count", "Green interlace OFF count 2"="GI Frequency, OFF count", "Green FB Count"="Green FB Count") -> ("error out"=w2403:errorcluster)  [unwired: 1 out]
      }
      event #31 {
        w2572 = 123.0  # AOM cal (nm/MHz)
        n421 = event-data() -> ()  [unwired: 7 out]
        n422 = local read "BD 1 Frequency 1 (MHz)"() -> (w2555:dbl)
        n423 = local read "BD 2 Frequency 1 (MHz)"() -> (w2561:dbl)
        n424 = local read "X RF Frequency Limits (MHz)"() -> (w2559:T11)
        n425 = local read "Y RF Frequency Limits (MHz)"() -> (w2556:T11)
        n426 = local read "AOM X Cal (nm/MHz)"() -> (w2547:dbl)
        n427 = Negate(x="Scan Range (nm)") -> (-x=w2524:dbl)
        n428 = Divide(x=w2524, y=w2547) -> (x/y=w2528:dbl)
        n429 = Select(t=w2559, s="Scan BD", f=w2556) -> (s? t:f=w2558:T11)
        n430 = Select(t=w2555, s="Scan BD", f=w2561) -> (s? t:f=w2560:dbl)
        n431 = Unbundle By Name(w2558) -> ("Maximum"=w2567:dbl, "Minimum"=w2566:dbl)
        n432 = Add(x=w2528, y=w2560) -> (x+y=w2564:dbl)
        n433 = Divide(x=w2524, y="Step Size (nm)") -> (x/y=w2544:dbl)
        n434 = Divide(x="Step Size (nm)", y=w2547) -> (x/y=w2553:dbl)
        n435 = Absolute Value(x=w2544) -> (abs(x)=w2527:dbl)
        n436 = Sign(1:w2524) -> (0:w2525:dbl)
        n437 = In Range and Coerce(upper limit=w2567, x=w2564, lower limit=w2566) -> (coerced(x)=w2563:dbl, In Range?=w2565:bool)
        n438 = To Unsigned Quad Integer(1:w2527) -> (0:w2543:u64)
        "Scan steps (AOD)" <- w2543
        n439 = call "IR AOM freq to word.vi"("Frequency In (MHz)"=w2553) -> ("Frequency Word Out (double)"=w2550:dbl)
        n440 = Multiply(x=w2525, y=w2550) -> (x*y=w2526:dbl)
        n441 = Subtract(x=w2564, y=w2563) -> (x-y=w2562:dbl)
        n442 = To Quad Integer(1:w2526) -> (0:w2549:i64)
        "Incr. int (AOD)" <- w2549
        n443 = Subtract(x=w2528, y=w2562) -> (x-y=w2548:dbl)
        "Scan Range (MHz)" <- w2548
        n444 = Select(t=w2528, s=w2565, f=w2548) -> (s? t:f=w2568:dbl)
        n445 = Multiply(x=w2548, y=w2547) -> (x*y=w2546:dbl)
        n446 = Decrement(x=w2543) -> (x-1=w2596:u64)
        n447 = Negate(x=w2546) -> (-x=w2542:dbl)
        n448 = local write "Scan Range (nm)"(w2542) -> ()
        n449 = Divide(x=w2568, y=w2596) -> (x/y=w2552:dbl)
        "Scan Increment (MHz)" <- w2552
        n450 = call "IR AOM freq to word.vi"("Frequency In (MHz)"=w2552) -> ("Frequency Word Out (double)"=w2551:dbl)
        n451 = Divide(x="Step Size (nm)", y="Scan Speed (nm/s)") -> (x/y=w2539:dbl)
        n452 = To Quad Integer(1:w2551) -> ()  [unwired: 1 out]
        n453 = local read "Number Interlace Sets"() -> (w2522:u8)
        n454 = local read "AI Count (ticks)"() -> (w2523:u32)
        n455 = local read "Total Counts (ticks)"() -> (w2521:u32)
        n456 = local read "# Samples/trap"() -> (w2554:dbl)
        n457 = Multiply(x=w2523, y=w2522) -> (x*y=w2520:u32)
        n458 = Divide(x=w2521, y=w2520) -> (x/y=w2519:dbl)
        n459 = Select(t=w2555, s="Scan BD", f=w2561) -> (s? t:f=w2593:dbl)
        "Initial freq. (MHz)" <- w2593
        n460 = Add(x=w2568, y=w2593) -> (x+y=→"Final freq. (MHz)":dbl)
        n461 = Divide(x=w2521, y=40000000.0) -> (x/y=w2538:dbl)
        n462 = Divide(x=w2539, y=w2538) -> (x/y=w2537:dbl)
        n463 = To Unsigned Quad Integer(1:w2537) -> (0:w2536:u64)
        "Cycles/step (AOD)" <- w2536
        n464 = xnode "Read/Write Control"("FPGA VI Reference In"=w2604, "error in"=w2603, "Scan steps"=w2543, "Number of scans"="Number of F/B Scans (AOD)", "Cycles per step"=w2536, "Scan freq.  increment"=w2549, "Scan BD"="Scan BD") -> ("error out"=w2602:errorcluster)  [unwired: 1 out]
        n465 = Multiply(x=w2543, y=w2536) -> (x*y=w2597:u64)
        n466 = Multiply(x=w2597, y=u64 2) -> (x*y=w2518:u64)
        n467 = Multiply(x=w2519, y=w2518) -> (x*y=w2517:dbl)
        "Data points/scan (f/b)" <- w2517
        n468 = Multiply(x=w2517, y="Number of F/B Scans (AOD)") -> (x*y=w2600:dbl)
        "Data points/scans" <- w2600
        n469 = Divide(x=w2600, y=w2554) -> (x/y=→"N sets should be saved":dbl)
        n470 = Multiply(x=w2597, y=w2538) -> (x*y=w2535:dbl)
        "Time/Scan (s) (AOD)" <- w2535
        n471 = Select(t=w2568, s="Scan BD", f=0.0) -> (s? t:f=w2594:dbl)
        n472 = Select(t=0.0, s="Scan BD", f=w2568) -> (s? t:f=w2590:dbl)
        n473 = local read "BD 2 Frequency 2 (MHz)"() -> (w2586:dbl)
        n474 = local read "BD 1 Frequency 2 (MHz)"() -> (w2589:dbl)
        n475 = Add(x=w2590, y=w2561) -> (x+y=w2587:dbl)
        n476 = Add(x=w2555, y=w2594) -> (x+y=w2588:dbl)
        n477 = Multiply(x=w2535, y=2.0) -> (x*y=w2534:dbl)
        n478 = Multiply(x=w2534, y="Number of F/B Scans (AOD)") -> (x*y=w2531:dbl)
        n479 = Divide(x=w2531, y=60.0) -> (x/y=→"Time to Finish All (min)":dbl)
        n480 = Add(x="Trap 2 Bead Size (nm)", y="Trap 1 Bead Size (nm)") -> (x+y=w2576:dbl)
        n481 = Divide(x=w2576, y=2.0) -> (x/y=w2570:dbl)
        n482 = Subtract(x=w2587, y=w2586) -> (x-y=w2584:dbl)
        n483 = Subtract(x=w2588, y=w2589) -> (x-y=w2585:dbl)
        n484 = local read "Initial delta (MHz)"() -> (w2573:dbl)
        n485 = Square(x=w2584) -> (x^2=w2583:dbl)
        n486 = Square(x=w2585) -> (x^2=w2582:dbl)
        n487 = Add(x=w2582, y=w2583) -> (x+y=w2581:dbl)
        n488 = Square Root(x=w2581) -> (sqrt(x)=w2580:dbl)
        "Final delta (MHz)" <- w2580
        n489 = Multiply(x=w2572, y=w2580) -> (x*y=w2579:dbl)
        n490 = Multiply(x=w2573, y=w2572) -> (x*y=w2571:dbl)
        n491 = Subtract(x=w2571, y=w2570) -> (x-y=→"Initial sep (nm)":dbl)
        n492 = Subtract(x=w2579, y=w2570) -> (x-y=→"Final sep (nm)":dbl)
      }
      event #32 {
        n493 = event-data() -> ()  [unwired: 7 out]
        n494 = local read "Freq or Amp switch first"() -> (w2691:bool)
        n495 = local read "Freq switch delay"() -> (w2694:u16)
        n496 = local read "Amp switch delay"() -> (w2692:u16)
        n497 = local read "Swap F1 and F2"() -> (w2693:bool)
        n498 = xnode "Read/Write Control"("FPGA VI Reference In"=w2697, "error in"=w2696, "Freq switch delay"=w2694, "Swap F1 and F2"=w2693, "Amp switch delay"=w2692, "Freq or Amp switch first"=w2691) -> ("error out"=w2695:errorcluster)  [unwired: 1 out]
      }
      event #33 {
        n499 = event-data() -> ()  [unwired: 7 out]
        n500 = Select(t="Scan lines", s="2D or 1D Scan", f="Number of scans (MCL)") -> (s? t:f=w2794:u64)
        n501 = Decrement(x="Scan steps (MCL)") -> (x-1=w2811:u64)
        n502 = Divide(x="Scan Range (V)", y=w2811) -> (x/y=w2810:dbl)
        "Scan Increment (V)" <- w2810
        n503 = local read "APD Integration Time (s)"() -> (w2802:dbl)
        n504 = Multiply(x=w2810, y=32767.0) -> (x*y=w2819:dbl)
        n505 = Divide(x=w2819, y=10.0) -> (x/y=w2808:dbl)
        "Actual incr" <- w2808
        n506 = local read "Update Count (MCL)"() -> (w2815:u32)
        n507 = Round Toward -Infinity(1:w2808) -> (0:w2818:dbl)
        n508 = Multiply(x=w2802, y=40000000.0) -> (x*y=w2816:dbl)
        n509 = To Word Integer(number=w2818) -> (16bit integer=w2809:i16)
        "Incr. int (MCL)" <- w2809
        n510 = Divide(x=w2816, y=w2815) -> (x/y=w2814:dbl)
        n511 = Multiply(x="N APD Samp/step", y=w2814) -> (x*y=w2813:dbl)
        "Cycles/step (MCL)" <- w2813
        n512 = Multiply(x="N APD Samp/step", y="Scan steps (MCL)") -> (x*y=w2804:dbl)
        n513 = local read "APD Samples/FIFO Acq."() -> (w2801:dbl)
        n514 = Multiply(x=w2804, y=u64 2) -> (x*y=w2803:dbl)
        "Data points/scan (f+b)" <- w2803
        n515 = Multiply(x=w2803, y=w2794) -> (x*y=w2823:dbl)
        "Data points/scans (MCL)" <- w2823
        n516 = Multiply(x=w2802, y=w2803) -> (x*y=w2795:dbl)
        "Time/f+b scan (s) (MCL)" <- w2795
        n517 = Divide(x=w2823, y=w2801) -> (x/y=→"N sets should be saved (MCL)":dbl)
        n518 = Multiply(x=w2795, y=w2794) -> (x*y=→"Total Time (s)":dbl)
        n519 = Not(x="Fast Scan Dir") -> (.not. x?=w2799:bool)
        n520 = xnode "Read/Write Control"("FPGA VI Reference In"=w2827, "error in"=w2826, "Scan steps (MCL)"="Scan steps (MCL)", "Number of scans (MCL)"=w2794, "Cycles per step (MCL)"=w2813, "Scan freq.  increment (MCL)"=w2809, "1D or 2D Scan?"="2D or 1D Scan", "MCL Scan Axis"=w2799, "Cont. Scan (MCL)"="Continuous MCL Scanning") -> ("error out"=w2825:errorcluster)  [unwired: 1 out]
      }
      event #34 {
        w2964 = 1000.0 ("y")
        n521 = event-data() -> ()  [unwired: 7 out]
        n522 = local read "Save file name"() -> (w2989:path)
        n523 = local write "Read Cal"(FALSE ("Read Cal")) -> ()
        n524 = Strip Path(path=w2989) -> (stripped path=w2988:path)  [unwired: 1 out]
        n525 = Path To String(path=w2988) -> (string=w2987:string)
        n526 = Concatenate Strings(w2987, "\\current.cal" ("string")) -> (w2985:string)
        n527 = String To Path(string=w2985) -> (path=w2984:path)
        n528 = Open/Create/Replace File(file path (use dialog)=w2984, operation (0:open)=T20."open", access (0:read/write)=enum16{"read/write", "read-only", "write-only"}."read-only") -> (refnum out=w2992:refnum<file>, error out=w2978:errorcluster)  [unwired: 1 in, 3 out]
        n529 = Deny Access(4:w2978, 7:w2992) -> (0:w2977:errorcluster, 3:w2983:refnum<file>)  [unwired: 1 out]
        n530 = Read from Binary File(5:0.0, 8:w2977, 9:T19."big-endian, network order" ("byte order (0:big-endian, network order)"), 10:-1 ("count (1)"), 11:w2983) -> (0:w2976:errorcluster, 2:w2974:dbl[], 3:w2979:refnum<file>)  [unwired: 2 out]
        n531 = Array To Cluster(array=w2974) -> (cluster=w2973:T22)
        n532 = Unbundle(w2973) -> ("[0]"=w2972:dbl, "[1]"=w2971:dbl, "[2]"=w2970:dbl, "[3]"=w2969:dbl, "[4]"=w2968:dbl, "[5]"=w2967:dbl)
        n533 = Close File(refnum=w2979, error in=w2976) -> (error out=→"Read cal error":errorcluster)  [unwired: 1 out]
        n534 = Multiply(x=w2967, y=w2964) -> (x*y=w2965:dbl)
        n535 = local write "T2 kappa_x (pN/nm)"(w2969) -> ()
        n536 = local write "T1 kappa_x (pN/nm)"(w2970) -> ()
        n537 = local write "T1 alpha_x (nm/V)"(w2972) -> ()
        n538 = local write "T2 alpha_x (nm/V)"(w2971) -> ()
        n539 = Multiply(x=w2968, y=w2964) -> (x*y=w2966:dbl)
        n540 = local write "T1 offset_x (mV)"(w2966) -> ()
        n541 = local write "T2 offset_x (mV)"(w2965) -> ()
      }
      event #35 {
        n542 = event-data() -> ()  [unwired: 7 out]
        n543 = local write "MCL Scanning"(FALSE ("MCL Scanning")) -> ()
        n544 = xnode "Read/Write Control"("FPGA VI Reference In"=w2997, "error in"=w2996, "Abort scan (MCL)"="Abort MCL Scan") -> ("error out"=w2995:errorcluster)  [unwired: 1 out]
      }
      event #36 {
        n545 = event-data() -> ()  [unwired: 7 out]
        n546 = xnode "Read/Write Control"("FPGA VI Reference In"=w3038, "error in"=w3037, "MCL count"="Update Count (MCL)") -> ("error out"=w3036:errorcluster)  [unwired: 1 out]
      }
      event #37 {
        n547 = event-data() -> ()  [unwired: 7 out]
        n548 = Negate(x="Phase adjust (MCL)") -> (-x=w3083:i16)
        n549 = Select(t=w3083, s="- phase (MCL)", f="Phase adjust (MCL)") -> (s? t:f=w3081:i16)
        n550 = Or(x="- phase (MCL)", y="+ phase (MCL)") -> (x .or. y?=w3076:bool)
        n551 = xnode "Read/Write Control"("FPGA VI Reference In"=w3085, "error in"=w3084, "Phase count adjustment (MCL)"=w3081) -> ("FPGA VI Reference Out"=w3077:T13, "error out"=w3078:errorcluster)
        n552 = xnode "Read/Write Control"("FPGA VI Reference In"=w3077, "error in"=w3078, "+ phase (MCL)"=w3076) -> ("error out"=w3075:errorcluster)  [unwired: 1 out]
      }
      event #38 {
        n553 = event-data() -> ()  [unwired: 7 out]
        n554 = xnode "Read/Write Control"("FPGA VI Reference In"=w3162, "error in"=w3161, "Abort scan"="Abort AOD Scan") -> ("error out"=w3160:errorcluster)  [unwired: 1 out]
      }
      event #39 {
        n555 = event-data() -> ()  [unwired: 7 out]
        n556 = xnode "Read/Write Control"("FPGA VI Reference In"=w3203, "error in"=w3202, "Cont. Scan"="Continuous AOD Scanning") -> ("error out"=w3201:errorcluster)  [unwired: 1 out]
      }
      event #40 {
        n557 = event-data() -> ()  [unwired: 7 out]
        n558 = call "Create new save file.vi"("Insert"="", "Ext"=".dat" ("string"), "Index In"="Index") -> ("Path Out"=→"Save file name":path, "Index Out"=w3241:dbl)
        "Save index" <- w3241
        n559 = local write "Index"(w3241) -> ()
      }
      event #41 {
        w3256 = 10.0 ("y")
        w3255 = 32767.0 ("y")
        n560 = event-data() -> ()  [unwired: 7 out]
        n561 = local read "AO2"() -> (w3254:dbl)
        n562 = local read "AO1"() -> (w3251:dbl)
        n563 = Multiply(x=w3251, y=w3255) -> (x*y=w3250:dbl)
        n564 = Multiply(x=w3254, y=w3255) -> (x*y=w3253:dbl)
        n565 = Divide(x=w3250, y=w3256) -> (x/y=w3249:dbl)
        n566 = Divide(x=w3253, y=w3256) -> (x/y=w3252:dbl)
        n567 = To Word Integer(number=w3249) -> (16bit integer=w3257:i16)
        n568 = To Word Integer(number=w3252) -> (16bit integer=w3258:i16)
        n569 = xnode "Read/Write Control"("FPGA VI Reference In"=w3248, "error in"=w3247, "AO1"=w3257, "AO2"=w3258) -> ("error out"=w3246:errorcluster)  [unwired: 1 out]
      }
      event #42 {
        n570 = event-data() -> ()  [unwired: 7 out]
        n571 = local read "Syringe Pump Serial Port"() -> (w3314:refnum<visa-resource-name>)
        n572 = local read "Pump write delay (ms)"() -> (w3315:dbl)
        n573 = case shown="True" "Inject Top Channel" {
          tunnel: w3315 -> [w3320 w3328]
          tunnel: w3314 -> [w3317 w3327]
          frame #0 {
            n574 = flat-sequence {
              tunnel: w3317 -> [w3321]
              tunnel: [w3321] -> w3318
              tunnel: w3320 -> [_]
              tunnel: [w3324] -> w3319
              tunnel: w3318 -> [w3324]
              tunnel: w3319 -> [w3325]
              frame #0 {
                n575 = call "Write to pump.vi"("string"="enter pump1", "VISA resource name"=w3321) -> ()  [unwired: 1 out]
              }
              frame #1 {
                n576 = Wait (ms)(milliseconds to wait="Pump pause delay (ms)") -> ()  [unwired: 1 out]
              }
              frame #2 {
                n577 = call "Write to pump.vi"("string"="stop", "VISA resource name"=w3325) -> ()  [unwired: 1 out]
              }
            }
          }
          frame #1 {
            n578 = flat-sequence {
              tunnel: w3327 -> [w3337]
              tunnel: w3328 -> [w3332]
              tunnel: w3328 -> [w3339]
              tunnel: w3327 -> [w3340]
              frame #0 {
                n579 = local read "All Pump Parameters"() -> (w3331:T4)
                n580 = Unbundle By Name(w3331) -> ("Pump 1"=w3338:T23)
                n581 = call "Set pump parameters.vi"("Pump write delay (ms)"=w3332, "Volume (uL)"="Top Ch Inject Volume (uL)", "Rate (uL/h)"="Top Ch Inject Rate (ul/h)", "Units"=4.0, "Pump #"=1.0, "Pump Parameters In"=w3338, "VISA resource name"=w3337) -> ("Pump Parameters Out"=w3330:T23)  [unwired: 3 in]
                n582 = Bundle By Name(cluster=w3331, "Pump 1"=w3330) -> (w3329:T4)
                n583 = local write "All Pump Parameters"(w3329) -> ()
              }
              frame #1 {
                n584 = Wait (ms)(milliseconds to wait=w3339) -> ()  [unwired: 1 out]
              }
              frame #2 {
                n585 = call "Write to pump.vi"("string"="start", "VISA resource name"=w3340) -> ()  [unwired: 1 out]
              }
            }
          }
        }
      }
      event #43 {
        n586 = event-data() -> ()  [unwired: 7 out]
        n587 = local read "Pump write delay (ms)"() -> (w3343:dbl)
        n588 = case shown="False" "Inject Bottom Channel" {
          tunnel: w3343 -> [w3348 w3356]
          tunnel: "Syringe Pump Serial Port" -> [w3345 w3355]
          frame #0 {
            n589 = flat-sequence {
              tunnel: w3345 -> [w3349]
              tunnel: [w3349] -> w3346
              tunnel: w3348 -> [_]
              tunnel: [w3352] -> w3347
              tunnel: w3346 -> [w3352]
              tunnel: w3347 -> [w3353]
              frame #0 {
                n590 = call "Write to pump.vi"("string"="enter pump3", "VISA resource name"=w3349) -> ()  [unwired: 1 out]
              }
              frame #1 {
                n591 = local read "Pump pause delay (ms)"() -> (w3351:u32)
                n592 = Wait (ms)(milliseconds to wait=w3351) -> ()  [unwired: 1 out]
              }
              frame #2 {
                n593 = call "Write to pump.vi"("string"="stop", "VISA resource name"=w3353) -> ()  [unwired: 1 out]
              }
            }
          }
          frame #1 {
            n594 = flat-sequence {
              tunnel: w3355 -> [w3365]
              tunnel: w3356 -> [w3360]
              tunnel: w3356 -> [w3367]
              tunnel: w3355 -> [w3368]
              frame #0 {
                n595 = local read "All Pump Parameters"() -> (w3359:T4)
                n596 = Unbundle By Name(w3359) -> ("Pump 3"=w3366:T23)
                n597 = call "Set pump parameters.vi"("Pump write delay (ms)"=w3360, "Volume (uL)"="Bottom Ch Inject Volume (uL)", "Rate (uL/h)"="Bottom Ch Inject Rate (ul/h)", "Units"=4.0, "Pump #"=3.0, "Pump Parameters In"=w3366, "VISA resource name"=w3365) -> ("Pump Parameters Out"=w3358:T23)  [unwired: 3 in]
                n598 = Bundle By Name(cluster=w3359, "Pump 3"=w3358) -> (w3357:T4)
                n599 = local write "All Pump Parameters"(w3357) -> ()
              }
              frame #1 {
                n600 = Wait (ms)(milliseconds to wait=w3367) -> ()  [unwired: 1 out]
              }
              frame #2 {
                n601 = call "Write to pump.vi"("string"="start", "VISA resource name"=w3368) -> ()  [unwired: 1 out]
              }
            }
          }
        }
      }
      event #44 {
        n602 = event-data() -> ()  [unwired: 7 out]
        n603 = local read "Pump write delay (ms)"() -> (w3372:dbl)
        n604 = flat-sequence {
          tunnel: w3370 -> [w3385]
          tunnel: w3372 -> [w3381]
          tunnel: "Flush Center Channel" -> [_]
          tunnel: w3372 -> [w3387]
          tunnel: w3370 -> [w3388]
          frame #0 {
            n605 = local read "All Pump Parameters"() -> (w3380:T4)
            n606 = Multiply(x=60.0, y="Flush Center Ch Rate (ul/m)") -> (x*y=w3377:dbl)
            n607 = Unbundle By Name(w3380) -> ("Pump 2"=w3386:T23)
            n608 = call "Set pump parameters.vi"("Pump write delay (ms)"=w3381, "Volume (uL)"="Flush Center Ch Volume (uL)", "Rate (uL/h)"=w3377, "Units"=3.0, "Pump #"=2.0, "Pump Parameters In"=w3386, "VISA resource name"=w3385) -> ("Pump Parameters Out"=w3379:T23)  [unwired: 3 in]
            n609 = Bundle By Name(cluster=w3380, "Pump 2"=w3379) -> (w3378:T4)
            n610 = Add(x="Flush Center Ch Volume (uL)", y="Total Volume\nFlushed (uL)") -> (x+y=w3374:dbl)
            n611 = local write "All Pump Parameters"(w3378) -> ()
            n612 = local write "Total Volume\nFlushed (uL)"(w3374) -> ()
          }
          frame #1 {
            n613 = Wait (ms)(milliseconds to wait=w3387) -> ()  [unwired: 1 out]
          }
          frame #2 {
            n614 = call "Write to pump.vi"("string"="start", "VISA resource name"=w3388) -> ()  [unwired: 1 out]
          }
        }
        n615 = local read "Syringe Pump Serial Port"() -> (w3370:refnum<visa-resource-name>)
      }
    }
    "error out 2" <- w662
    n616 = node-c288() -> ()  [unwired: 2 out]
  }
  n617 = property on="pos 1 z" class="DigNum (strict)"("Data Range"=w52) -> ()  [unwired: 2 in, 2 out]
  n618 = property on="pos 2 z" class="DigNum (strict)"("Data Range"=w52) -> ()  [unwired: 2 in, 2 out]
  n619 = property on="pos 3 z" class="DigNum (strict)"("Data Range"=w52) -> ()  [unwired: 2 in, 2 out]
  n620 = property on="pos 4 z" class="DigNum (strict)"("Data Range"=w52) -> ()  [unwired: 2 in, 2 out]
  n621 = node-c288() -> (w4:T16)  [unwired: 4 out]
  n622 = node-c288() -> (w12:T16)  [unwired: 4 out]
  n623 = node-c288(i64 1 ("Period")) -> (w123:T16)  [unwired: 3 out]
  n624 = node-c288() -> (w6:T16)  [unwired: 4 out]
  n625 = node-c288() -> (w10:T16)  [unwired: 4 out]
  n626 = timed-loop "Rough control of MCL mirror stage (debugging)" {
    tunnel: w73 -> [w3392]
    tunnel: [w3391] -> w179
    timing: w4 -> [_]
    timing-out: [_] -> w3
    stop <- w3391 stop-if-true
    n627 = node-c288() -> ()  [unwired: 2 out]
    n628 = case shown="1" "MCL Mode" {
      tunnel: w3392 -> [_ w3395 w3497]
      frame #0 {
      }
      frame #1 {
        n629 = node-c288() -> (w3397:T16)  [unwired: 4 out]
        n630 = timed-loop "Oscillate MCL mirror" {
          timing: w3397 -> [_]
          timing-out: [_] -> w3396
          tunnel: w3395 -> [w3436]
          i -> [w3435]
          stop <- w3398 stop-if-true
          n631 = node-c288() -> (w3434:i64)  [unwired: 1 out]
          n632 = Multiply(x="AO1", y=32767.0) -> (x*y=w3430:dbl)
          n633 = Multiply(x="AO2", y=32767.0) -> (x*y=w3425:dbl)
          n634 = Divide(x=w3430, y=10.0) -> (x/y=w3431:dbl)
          n635 = Divide(x=w3425, y=10.0) -> (x/y=w3426:dbl)
          n636 = To Word Integer(number=w3431) -> (16bit integer=w3423:i16)
          n637 = To Word Integer(number=w3426) -> (16bit integer=w3422:i16)
          n638 = Divide(x=w3434, y=i64 1000) -> (x/y=w3405:dbl)
          n639 = Multiply(x=w3405, y=w3435) -> (x*y=w3416:dbl)
          n640 = Multiply(x="Osc. freq. (Hz) 2", y=6.283185307179586) -> (x*y=w3417:dbl)
          n641 = Multiply(x=w3417, y=w3416) -> (x*y=w3415:dbl)
          n642 = Sine(x=w3415) -> (sin(x)=w3414:dbl)
          n643 = Multiply(x=w3414, y="Osc. amp. (V)") -> (x*y=w3412:dbl)
          n644 = Add(x=w3412, y="Osc. center (V)") -> (x+y=w3410:dbl)
          n645 = Divide(x=w3410, y=10.0) -> (x/y=w3408:dbl)
          n646 = Multiply(x=w3408, y=32767.0) -> (x*y=w3403:dbl)
          n647 = Select(t=w3403, s="Scan axis", f=w3423) -> (s? t:f=w3421:dbl)
          n648 = Select(t=w3422, s="Scan axis", f=w3403) -> (s? t:f=w3420:dbl)
          n649 = local read "MCL Mode"() -> (w3402:u16)
          n650 = Not Equal?(x=w3402, y=u16 1) -> (x != y?=w3399:bool)
          n651 = local read "Stop All"() -> (w3400:bool)
          n652 = xnode "Read/Write Control"("FPGA VI Reference In"=w3436, "AO1"=w3421, "AO2"=w3420) -> ()  [unwired: 1 in, 2 out]
          n653 = Compound Arithmetic op=OR(w3400, w3399) -> (w3398:bool)
          n654 = node-c288() -> ()  [unwired: 2 out]
        }
        n655 = node-c288(w3396) -> ()  [unwired: 1 out]
      }
      frame #2 {
        n656 = case shown="True" "Start Scan" {
          tunnel: w3497 -> [_ w3509]
          frame #0 {
          }
          frame #1 {
            n657 = Subtract(x="End (V)", y="Begin (V)") -> (x-y=w3505:dbl)
            n658 = Decrement(x="N Points") -> (x-1=w3504:dbl)
            n659 = Divide(x=w3505, y=w3504) -> (x/y=w3502:dbl)
            n660 = for {
              N: "N Points" -> [_]
              tunnel: "Begin (V)" -> [w3522]
              tunnel: w3509 -> [w3514]
              tunnel: [w3513] -> w3508 mode=indexing
              tunnel: w3502 -> [w3512]
              tunnel: [w3510] -> w3501 mode=indexing
              i -> [w3521]
              n661 = Multiply(x=w3512, y=w3521) -> (x*y=w3520:dbl)
              n662 = Add(x=w3522, y=w3520) -> (x+y=w3517:dbl)
              n663 = local read "Scan axis"() -> (w3511:bool)
              n664 = local read "AO1"() -> (w3519:dbl)
              n665 = local read "AO2"() -> (w3518:dbl)
              n666 = Select(t=w3517, s=w3511, f=w3519) -> (s? t:f=w3516:dbl)
              n667 = Select(t=w3518, s=w3511, f=w3517) -> (s? t:f=w3515:dbl)
              n668 = flat-sequence {
                tunnel: w3516 -> [w3526]
                tunnel: w3515 -> [w3525]
                tunnel: w3514 -> [w3523]
                tunnel: [w3591] -> w3513
                tunnel: [w3590] -> w3510
                frame #0 {
                  w3529 = 10.0 ("y")
                  w3524 = 32767.0 ("y")
                  n669 = Multiply(x=w3526, y=w3524) -> (x*y=w3532:dbl)
                  n670 = Multiply(x=w3525, y=w3524) -> (x*y=w3530:dbl)
                  n671 = Divide(x=w3532, y=w3529) -> (x/y=w3533:dbl)
                  n672 = Divide(x=w3530, y=w3529) -> (x/y=w3531:dbl)
                  n673 = To Word Integer(number=w3533) -> (16bit integer=w3527:i16)
                  n674 = To Word Integer(number=w3531) -> (16bit integer=w3528:i16)
                  n675 = xnode "Read/Write Control"("FPGA VI Reference In"=w3523, "AO1"=w3527, "AO2"=w3528) -> ()  [unwired: 1 in, 2 out]
                }
                frame #1 {
                  n676 = Wait (ms)(milliseconds to wait="DAQ Delay (ms)") -> ()  [unwired: 1 out]
                }
                frame #2 {
                  n677 = local read "Slow mean"() -> (w3591:dbl)
                  n678 = local read "Sigma"() -> (w3590:dbl)
                }
              }
            }
            n679 = Bundle("Begin (V)"="Begin (V)", w3502, w3508) -> (→"MCL Scan":cluster{"Begin (V)":dbl, dbl, dbl[]})  [unwired: 1 out]
            n680 = Bundle("Begin (V)"="Begin (V)", w3502, w3501) -> (→"MCL Scan 2":cluster{"Begin (V)":dbl, dbl, dbl[]})  [unwired: 1 out]
          }
        }
      }
    }
    n681 = local read "Stop All"() -> (w3391:bool)
    n682 = node-c288() -> ()  [unwired: 2 out]
  }
  n683 = timed-loop "Mouse control trap position (AOD deflection)" {
    tunnel: [w3593] -> w130
    tunnel: w73 -> [w3592]
    timing: w12 -> [_]
    timing-out: [_] -> w11
    stop <- w3593 stop-if-true
    n684 = node-c288() -> ()  [unwired: 2 out]
    n685 = event shown="[0] \"Pane\": Mouse Down" {
      selector: _ -> [_ _]
      dyn-events: _ -> [_ _]
      timeout: _ -> [_ _]
      tunnel: w3592 -> [w3596 _]
      event #0 {
        n686 = event-data() -> ("Time"=w3598:u32, "Coords"=w3597:T6, "Button"=w3599:u16)  [unwired: 6 out]
        n687 = case shown="3" w3599 {
          tunnel: w3598 -> [_ w3606]
          tunnel: w3597 -> [_ w3604]
          tunnel: w3596 -> [_ w3602]
          frame #0 {
          }
          frame #1 {
            n688 = local read "BD 2 Frequency 1 (MHz)"() -> (w3600:dbl)
            n689 = local read "BD 1 Frequency 1 (MHz)"() -> (w3601:dbl)
            n690 = local write "Manipulating Trap"(TRUE ("Manipulating Trap")) -> ()
            n691 = local write "Coords"(T6 {"Horizontal"=0, "Vertical"=0} ("Coords")) -> ()
            n692 = while {
              tunnel: w3606 -> [w3611]
              tunnel: w3604 -> [w3610]
              tunnel: w3602 -> [w3609]
              tunnel: w3601 -> [w3608]
              tunnel: w3600 -> [w3607]
              stop <- w3612 stop-if-true
              n693 = event shown="[0] \"Pane\": Mouse Move" {
                selector: _ -> [_ _]
                dyn-events: _ -> [_ _]
                timeout: _ -> [_ _]
                tunnel: ["Force Manip Abort" w3676] -> w3612
                tunnel: w3611 -> [w3619 _]
                tunnel: w3610 -> [w3617 _]
                tunnel: w3609 -> [w3616 _]
                tunnel: w3608 -> [w3615 _]
                tunnel: w3607 -> [w3614 _]
                event #0 {
                  n694 = event-data() -> ("Time"=w3620:u32, "Coords"=w3621:T6)  [unwired: 3 out]
                  n695 = Less?(x=w3620, y=w3619) -> (x < y?=w3618:bool)
                  n696 = case "Makes sure old motion events prior to mouse click aren't used" shown="False" w3618 {
                    tunnel: w3621 -> [w3663 _]
                    tunnel: w3617 -> [w3664 _]
                    tunnel: w3616 -> [w3641 _]
                    tunnel: w3615 -> [w3637 _]
                    tunnel: w3614 -> [w3636 _]
                    frame #0 {
                      n697 = Subtract(x=w3663, y=w3664) -> (x-y=w3662:T6)
                      "Coords" <- w3662
                      n698 = local read "Y RF Frequency Limits (MHz)"() -> (w3622:T11)
                      n699 = To Double Precision Float(number=w3662) -> (double precision float=w3661:cluster{"Horizontal":dbl, "Vertical":dbl})
                      n700 = Multiply(x=cluster{"Horizontal":dbl, "Vertical":dbl} {"Horizontal"=-1.0, "Vertical"=1.0}, y="Manipulation Scaling") -> (x*y=w3657:cluster{"Horizontal":dbl, "Vertical":dbl})
                      n701 = Multiply(x=w3661, y=w3657) -> (x*y=w3659:cluster{"Horizontal":dbl, "Vertical":dbl})
                      n702 = local read "X RF Frequency Limits (MHz)"() -> (w3623:T11)
                      n703 = Unbundle By Name(w3659) -> ("Horizontal"=w3654:dbl, "Vertical"=w3658:dbl)
                      n704 = Boolean To (0,1)(Boolean="Manip. X?") -> (0, 1=w3652:i16)
                      n705 = Unbundle By Name(w3622) -> ("Maximum"=w3625:dbl, "Minimum"=w3624:dbl)
                      n706 = Boolean To (0,1)(Boolean="Manip. Y?") -> (0, 1=w3649:i16)
                      n707 = Multiply(x=w3658, y=w3649) -> (x*y=w3651:dbl)
                      n708 = Multiply(x=w3652, y=w3654) -> (x*y=w3655:dbl)
                      n709 = local read "BD 1 Frequency 2 (MHz)"() -> (w3639:dbl)
                      n710 = Unbundle By Name(w3623) -> ("Maximum"=w3627:dbl, "Minimum"=w3626:dbl)
                      n711 = local read "BD 2 Frequency 2 (MHz)"() -> (w3638:dbl)
                      n712 = Add(x=w3636, y=w3651) -> (x+y=w3629:dbl)
                      n713 = Add(x=w3637, y=w3655) -> (x+y=w3631:dbl)
                      n714 = In Range and Coerce(upper limit=w3627, x=w3631, lower limit=w3626) -> (coerced(x)=w3630:dbl)  [unwired: 1 out]
                      n715 = In Range and Coerce(upper limit=w3625, x=w3629, lower limit=w3624) -> (coerced(x)=w3628:dbl)  [unwired: 1 out]
                      n716 = Subtract(x=w3630, y=w3639) -> (x-y=w3648:dbl)
                      n717 = Subtract(x=w3628, y=w3638) -> (x-y=w3647:dbl)
                      n718 = Square(x=w3648) -> (x^2=w3646:dbl)
                      n719 = Square(x=w3647) -> (x^2=w3645:dbl)
                      n720 = Add(x=w3646, y=w3645) -> (x+y=w3644:dbl)
                      n721 = Square Root(x=w3644) -> (sqrt(x)=w3640:dbl)
                      n722 = In Range and Coerce(upper limit="Limit Max (MHz)", x=w3640, lower limit="Limit Min (MHz)") -> (In Range?=w3633:bool)  [unwired: 1 out]
                      n723 = Not(x="Limits Enable") -> (.not. x?=w3632:bool)
                      n724 = Or(x=w3633, y=w3632) -> (x .or. y?=w3634:bool)
                      n725 = case shown="True" w3634 {
                        tunnel: w3641 -> [_ w3674]
                        tunnel: w3640 -> [_ w3665]
                        tunnel: w3630 -> [_ w3672]
                        tunnel: w3639 -> [_ w3671]
                        tunnel: w3628 -> [_ w3670]
                        tunnel: w3638 -> [_ w3669]
                        tunnel: w3623 -> [_ w3667]
                        tunnel: w3622 -> [_ w3666]
                        frame #0 {
                        }
                        frame #1 {
                          n726 = local read "BD 1 Frequency 3 (MHz)"() -> (w3673:dbl)
                          n727 = local read "BD 2 Frequency 3 (MHz)"() -> (w3668:dbl)
                          n728 = local write "Trap Delta (MHz)"(w3665) -> ()
                          n729 = property on="Initial delta (MHz)" class="DigNum (strict)"("Val(Sgnl)"=w3665) -> ()  [unwired: 2 in, 2 out]
                          n730 = call "set RF board frequency - interlace.vi"("Board 2 Frequency Limits"=w3666, "Board 1 Frequency Limits"=w3667, "FPGA VI Reference In"=w3674, "Board 2 Frequency 3 (MHz)"=w3668, "Board 1 Frequency 3 (MHz)"=w3673, "Board 2 Frequency 2 (MHz)"=w3669, "Board 2 Frequency 1 (MHz)"=w3670, "Board 1 Frequency 2 (MHz)"=w3671, "Board 1 Frequency 1  (MHz)"=w3672) -> ()  [unwired: 1 in, 2 out]
                          n731 = local write "BD 2 Frequency 1 (MHz)"(w3670) -> ()
                          n732 = local write "BD 1 Frequency 1 (MHz)"(w3672) -> ()
                        }
                      }
                    }
                    frame #1 {
                    }
                  }
                }
                event #1 {
                  n733 = event-data() -> ("Button"=w3675:u16)  [unwired: 8 out]
                  n734 = case shown="3" w3675 {
                    tunnel: [FALSE TRUE] -> w3676
                    frame #0 {
                    }
                    frame #1 {
                      n735 = local write "Manipulating Trap"(FALSE ("Manipulating Trap")) -> ()
                    }
                  }
                }
              }
            }
          }
        }
      }
      event #1 {
        n736 = event-data() -> ()  [unwired: 6 out]
      }
    }
    n737 = local read "Stop All"() -> (w3593:bool)
    n738 = node-c288() -> ()  [unwired: 2 out]
  }
  n739 = flat-sequence "Video" {
    tunnel: [w3688] -> w185
    tunnel: w185 -> [w3724]
    tunnel: w183 -> [w3722]
    frame #0 {
      n740 = while {
        stop <- w3681 continue-if-true
        n741 = call "Close Video Capture.vi"() -> ("error code OUT"=w3683:i32)
        n742 = Equal?(x=w3683, y=0) -> (x = y?=w3681:bool)
      }
      n743 = local write "Stop All"(FALSE ("Stop All")) -> ()
    }
    frame #1 {
      n744 = call "DMR_Init.vi"() -> ()  [unwired: 3 out]
    }
    frame #2 {
      # "Setting the destination format to Mono8 makes sure that the image can be displayed in the intensity plot."
      n745 = call "DMR_GetDevice.vi"("search string IN"="DE019116701") -> ("device handle OUT"=w3706:i32)  [unwired: 4 in, 2 out]
      n746 = call "DMR_OpenDevice.vi"("device handle IN"=w3706) -> ("driver handle OUT"=w3689:i32)  [unwired: 4 out]
      n747 = call "DMR_FindList.vi"("flags IN"=u32 0 ("flags"), "list name IN"="" ("String"), "list type IN"=T24."camera descriptions", "driver handle IN"=w3689) -> ("list handle OUT"=w3692:i32)  [unwired: 2 out]
      n748 = call "DMR_FindList.vi"("flags IN"=u32 0 ("flags"), "list name IN"="Base", "list type IN"=T24."setting", "driver handle IN"=w3689) -> ("list handle OUT"=w3690:i32)  [unwired: 2 out]
      n749 = call "OBJ_GetHandle.vi"("object name IN"="VideoStandard", "list handle IN"=w3692) -> ("object handle OUT"=w3686:i32)  [unwired: 3 out]
      n750 = call "OBJ_GetHandle.vi"("object name IN"="PixelFormat", "list handle IN"=w3690) -> ("object handle OUT"=w3700:i32)  [unwired: 3 out]
      n751 = call "OBJ_SetS.vi"("value index IN"=0, "value IN"="NTSC M", "object handle IN"=w3686) -> ()  [unwired: 2 out]
      n752 = call "OBJ_SetS.vi"("value index IN"=0, "value IN"="Mono8" ("value"), "object handle IN"=w3700) -> ()  [unwired: 2 out]
      n753 = call "OBJ_GetHandle.vi"("object name IN"="VideoChannel", "list handle IN"=w3690) -> ("object handle OUT"=w3696:i32)  [unwired: 3 out]
      n754 = while {
        tunnel: [w3711] -> w3688
        tunnel: w3689 -> [w3708]
        stop <- w3709 continue-if-true
        n755 = call "DMR_ImageRequestSingle.vi"("request control IN"=0, "driver handle IN"=w3708) -> ("error code OUT"=w3710:i32, "driver handle OUT"=w3711:i32)  [unwired: 2 out]
        n756 = Equal To 0?(x=w3710) -> (x = 0?=w3709:bool)
      }
      n757 = call "OBJ_SetI.vi"("value index IN"=0, "value IN"=3 ("Video channel"), "object handle IN"=w3696) -> ()  [unwired: 2 out]
    }
    frame #3 {
      w3719 = T26 0 items=["Grayscale (U8)", "Grayscale (I16)", "Grayscale (SGL)", "Complex (CSG)", "RGB (U32)", "HSL (U32)", "RGB (U64)"] ("Image Type")
      n758 = call "IMAQ Create"("Image Name"="untitled", "Image Type"=w3719) -> ("New Image"=w3720:T27)  [unwired: 2 in, 2 out]
      n759 = node-c288() -> (w3718:T16)  [unwired: 4 out]
      n760 = Initialize Array(u32 0 ("Window Number (0...15)"), 480 ("dimension size"), 640 ("dimension size")) -> (w3713:u32[][])
      n761 = timed-loop {
        tunnel: w3724 -> [w3742]
        tunnel: [w3741] -> w3723
        tunnel: w3722 -> [w3740]
        tunnel: w3720 -> [w3739]
        timing: w3718 -> [_]
        timing-out: [_] -> w3717
        tunnel: w3713 -> [w3725]
        stop <- w3728 stop-if-true
        # "This block performs the \nactual image capture."
        n762 = node-c288() -> ()  [unwired: 2 out]
        n763 = local read "Stop All"() -> (w3729:bool)
        n764 = Reciprocal(x="Video Capture Rate (Hz)") -> (1/x=w3731:dbl)
        n765 = Or(x=FALSE, y=w3729) -> (x .or. y?=w3728:bool)
        n766 = Multiply(x=w3731, y=1000.0) -> (x*y=w3726:dbl)
        n767 = call "DMR_ImageRequestWaitFor.vi"("queue number IN"=0, "timeout(ms) IN"=500, "driver handle IN"=w3742) -> ("error code OUT"=w3746:i32, "request number OUT"=w3743:i32, "driver handle OUT"=w3744:i32)
        n768 = feedback #1(T25 refnum ("Avi Refnum")) -> (w3733:T25)
        n769 = case shown="True" "New Video File" {
          tunnel: [T25 refnum ("Avi Refnum") w3763] -> w3735
          tunnel: [FALSE TRUE] -> w3736
          tunnel: w3733 -> [_ w3759]
          frame #0 {
          }
          frame #1 {
            n770 = call "Create new save file.vi"("Ext"=".avi" ("string"), "Index In"="Video Index") -> ("Path Out"=w3755:path, "Index Out"=w3756:dbl)  [unwired: 1 in]
            "Path Out" <- w3755
            n771 = Not Equal?(x=w3759, y=T25 refnum ("Avi Refnum")) -> (x != y?=w3760:bool)
            n772 = Increment(x=w3756) -> (x+1=w3765:dbl)
            n773 = case shown="True" w3760 {
              tunnel: w3759 -> [_ w3766]
              frame #0 {
              }
              frame #1 {
                n774 = call "IMAQ AVI Close"("Avi Refnum"=w3766) -> ()  [unwired: 1 in, 10 out]
              }
            }
            n775 = call "IMAQ AVI Create"("Frames Per Second"=u32 30, "AVI Path"=w3755) -> ("Avi Refnum"=w3763:T25)  [unwired: 5 in, 4 out]
            n776 = local write "Video Index"(w3765) -> ()
          }
        }
        n777 = Equal To 0?(x=w3746) -> (x = 0?=w3745:bool)
        n778 = Select(t=w3735, s=w3736, f=w3733) -> (s? t:f=w3734:T25)
        n779 = case shown="True" w3745 {
          tunnel: w3744 -> [w3767 w3789]
          tunnel: w3743 -> [_ w3788]
          tunnel: [w3767 w3785] -> w3741
          tunnel: w3740 -> [_ w3775]
          tunnel: w3739 -> [_ w3768]
          tunnel: w3725 -> [_ w3772]
          tunnel: w3734 -> [_ w3770]
          frame #0 {
          }
          frame #1 {
            w3779 = u32 0 ("X-offset IN")
            n780 = call "DMR_GetImageRequestBufferData.vi"("driver handle IN"=w3789, "request number IN"=w3788) -> ("width OUT"=w3778:i32, "height OUT"=w3777:i32, "driver handle OUT"=w3784:i32, "request number OUT"=w3783:i32, "bytes per pixel OUT"=w3780:i32)  [unwired: 13 out]
            n781 = call "DMR_GetImageRequestBufferImageData.vi"("driver handle IN"=w3784, "request number IN"=w3783, "bytes per pixel IN"=w3780, "X-offset IN"=w3779, "Y-offset IN"=w3779, "height IN"=w3777, "width IN"=w3778) -> ("driver handle OUT"=w3782:u32, "request number OUT"=w3781:u32, "image OUT"=w3773:u32[][])  [unwired: 10 out]
            n782 = call "DMR_ImageRequestUnlock.vi"("request number IN"=w3781, "driver handle IN"=w3782) -> ("driver handle OUT"=w3787:i32)  [unwired: 1 in, 2 out]
            n783 = case shown="True" "Averaging" {
              tunnel: w3773 -> [w3795 w3800]
              tunnel: [w3795 w3799] -> w3769
              tunnel: w3772 -> [_ w3797]
              frame #0 {
              }
              frame #1 {
                (unwired) 1
                w3805 = 1
                n784 = feedback #2(w3797) -> (w3796:u32[][])
                n785 = Add(x=w3800, y=w3796) -> (x+y=w3801:u32[][])
                n786 = Select(t=w3797, s="Reset Averaging", f=w3801) -> (s? t:f=w3803:u32[][])
                n787 = feedback #3(w3805) -> (w3798:i32)
                n788 = Divide(x=w3801, y=w3798) -> (x/y=w3802:dbl[][])
                n789 = Increment(x=w3798) -> (x+1=w3806:i32)
                n790 = To Unsigned Long Integer(number=w3802) -> (unsigned 32bit integer=w3799:u32[][])
                n791 = Select(t=w3805, s="Reset Averaging", f=w3806) -> (s? t:f=w3804:i32)
              }
            }
            "Image" <- w3769
            n792 = case shown="True" "Capture and Save Image" {
              tunnel: w3769 -> [_ w3817]
              tunnel: w3775 -> [_ w3816]
              frame #0 {
              }
              frame #1 {
                n793 = To Unsigned Byte Integer(number=w3817) -> (unsigned 8bit integer=w3813:u8[][])
                n794 = call <vilib>:"Flatten Pixmap.vi"("colors"=w3816, "8-bit pixmap"=w3813) -> ("image data"=w3814:T28)  [unwired: 4 in, 5 out]
                n795 = call "Create new save file.vi"("Insert"="video_frame_" ("string"), "Ext"=".bmp" ("string"), "Index In"="Image Index") -> ("Path Out"=w3809:path, "Index Out"=w3815:dbl)
                n796 = call <vilib>:"Write BMP File.vi"("image data"=w3814, "path to BMP file"=w3809) -> ()  [unwired: 1 in, 9 out]
                n797 = Increment(x=w3815) -> (x+1=w3808:dbl)
                n798 = local write "Image Index"(w3808) -> ()
              }
            }
            n799 = case shown="True" "Capture Video" {
              tunnel: w3770 -> [_ w3794]
              tunnel: w3769 -> [_ w3792]
              tunnel: w3768 -> [_ w3791]
              frame #0 {
              }
              frame #1 {
                n800 = To Unsigned Byte Integer(number=w3792) -> (unsigned 8bit integer=w3793:u8[][])
                n801 = call "IMAQ ArrayToImage"("Image Pixels (U8)"=w3793, "Image"=w3791) -> ("Image Out"=w3790:T27)  [unwired: 4 in, 5 out]
                n802 = call "IMAQ AVI Write Frame"("Image"=w3790, "Avi Refnum"=w3794) -> ()  [unwired: 2 in, 8 out]
              }
            }
            n803 = call "DMR_ImageRequestSingle.vi"("request control IN"=0, "driver handle IN"=w3787) -> ("driver handle OUT"=w3785:i32)  [unwired: 3 out]
          }
        }
        n804 = node-c288(w3726) -> ()  [unwired: 1 out]
      }
      n805 = node-c288(w3717) -> ()  [unwired: 1 out]
      n806 = call "DMR_CloseDevice.vi"("driver handle IN"=w3723) -> ()  [unwired: 1 in, 4 out]
    }
    frame #4 {
      n807 = call "DMR_Close.vi"() -> ()  [unwired: 1 out]
    }
  }
  n808 = timed-loop "Acquire Data" {
    tunnel: w70 -> [w3991]
    tunnel: w69 -> [w3990]
    tunnel: [w4028] -> w226
    tunnel: [w4022] -> w224
    timing: w123 -> [_]
    timing-out: [_] -> w122
    stop <- "Stop All" stop-if-true
    w3871 = "NI_ChannelName" ("name")
    n809 = node-c288() -> ()  [unwired: 2 out]
    n810 = case "Reset data stream" shown="True" "Reset" {
      tunnel: w3991 -> [w6164 w6171]
      tunnel: w3990 -> [w6163 w6170]
      tunnel: [w6164 w6166] -> w3986
      tunnel: [w6163 w6165] -> w3985
      frame #0 {
      }
      frame #1 {
        w6169 = TRUE ("AI to FIFO")
        w6176 = FALSE ("AI to FIFO")
        n811 = local write "Overflow (data lost)"(FALSE ("Overflow (data lost)")) -> ()
        n812 = xnode "Read/Write Control"("FPGA VI Reference In"=w6171, "error in"=w6170, "AI to FIFO"=w6176, "APD to FIFO"=w6176) -> ("FPGA VI Reference Out"=w6174:T13, "error out"=w6175:errorcluster)
        n813 = xnode "Invoke Method"("FPGA VI Reference In"=w6174, "error in"=w6175) -> ("FPGA VI Reference Out"=w6172:T13, "error out"=w6173:errorcluster)
        n814 = xnode "Invoke Method"("FPGA VI Reference In"=w6172, "error in"=w6173) -> ("FPGA VI Reference Out"=w6168:T13, "error out"=w6167:errorcluster)
        n815 = xnode "Read/Write Control"("FPGA VI Reference In"=w6168, "error in"=w6167, "AI to FIFO"=w6169, "APD to FIFO"=w6169) -> ("FPGA VI Reference Out"=w6166:T13, "error out"=w6165:errorcluster)
      }
    }
    n816 = Or(x="Start AOD Scan", y="Trap Raster Scan") -> (x .or. y?=w3933:bool)
    n817 = And(x="Save scans", y=w3933) -> (x .and. y?=w3982:bool)
    n818 = case "Start AOM raster scan" shown="True" w3933 {
      tunnel: w3986 -> [w5403 w5412]
      tunnel: w3985 -> [w5402 w5411]
      tunnel: [w5403 w5405] -> w3984
      tunnel: [w5402 w5404] -> w3983
      frame #0 {
      }
      frame #1 {
        n819 = case shown="True" "Restart DMA? (AOD)" {
          tunnel: [w5778 w5779] -> w5406
          tunnel: [w5777 w5780] -> w5407
          tunnel: w5412 -> [w5778 w5786]
          tunnel: w5411 -> [w5777 w5785]
          frame #0 {
          }
          frame #1 {
            w5782 = FALSE ("AI to FIFO")
            n820 = xnode "Read/Write Control"("FPGA VI Reference In"=w5786, "error in"=w5785, "AI to FIFO"=w5782, "APD to FIFO"=w5782) -> ("FPGA VI Reference Out"=w5784:T13, "error out"=w5783:errorcluster)
            n821 = xnode "Invoke Method"("FPGA VI Reference In"=w5784, "error in"=w5783) -> ("FPGA VI Reference Out"=w5788:T13, "error out"=w5787:errorcluster)
            n822 = xnode "Invoke Method"("FPGA VI Reference In"=w5788, "error in"=w5787) -> ("FPGA VI Reference Out"=w5779:T13, "error out"=w5780:errorcluster)
            n823 = local write "Overflow (data lost)"(FALSE ("Overflow (data lost)")) -> ()
          }
        }
        n824 = case shown="True" "Move MCL Also?" {
          tunnel: w5407 -> [w5415 w5521]
          tunnel: w5406 -> [w5416 w5522]
          tunnel: [w5414 w5525] -> w5405
          tunnel: [w5413 w5524] -> w5404
          frame #0 {
            w5417 = TRUE ("AI to FIFO")
            n825 = xnode "Read/Write Control"("FPGA VI Reference In"=w5416, "error in"=w5415, "AI to FIFO"=w5417, "APD to FIFO"=w5417, "Start scan"=w5417) -> ("FPGA VI Reference Out"=w5414:T13, "error out"=w5413:errorcluster)
          }
          frame #1 {
            w5518 = FALSE ("1D or 2D Scan?")
            w5523 = TRUE ("AI to FIFO")
            # "Count for MCL loop"
            # "N total cycles"
            # "N steps"
            # "V_int"
            n826 = local read "Scan Range (nm)"() -> (w5500:dbl)
            n827 = local read "Number of F/B Scans (AOD)"() -> (w5517:u16)
            n828 = Sign(1:w5500) -> (0:w5499:dbl)
            n829 = Compound Arithmetic op=MULTIPLY(w5500, "MCL Step Position Ratio", "MCL/AOM Scale Tweak") -> (w5504:dbl)
            n830 = Negate(x=w5499) -> (-x=w5496:dbl)
            n831 = Multiply(x=w5496, y="MCL Step Increment (V_int)") -> (x*y=w5498:dbl)
            n832 = Divide(x=w5504, y="MCL X Cal (nm/V)") -> (x/y=w5510:dbl)
            n833 = Multiply(x=32767.0 ("y"), y=w5510) -> (x*y=w5516:dbl)
            n834 = local read "Total Counts (ticks)"() -> (w5501:u32)
            n835 = local read "Cycles/step (AOD)"() -> (w5512:u64)
            n836 = local read "Scan steps (AOD)"() -> (w5513:u64)
            n837 = Divide(x=w5516, y=10.0) -> (x/y=w5509:dbl)
            n838 = Divide(x=w5509, y="MCL Step Increment (V_int)") -> (x/y=w5507:dbl)
            n839 = Absolute Value(x=w5507) -> (abs(x)=w5495:dbl)
            n840 = Compound Arithmetic op=MULTIPLY(w5513, w5512, w5501) -> (w5508:u64)
            n841 = local write "wait to reset values"(w5523) -> ()
            n842 = local write "MCL Scanning"(w5523) -> ()
            n843 = Divide(x=w5508, y=w5495) -> (x/y=w5505:dbl)
            "MCL Count" <- w5505
            n844 = xnode "Read/Write Control"("FPGA VI Reference In"=w5522, "error in"=w5521, "Scan steps (MCL)"=w5495, "Number of scans (MCL)"=w5517, "Cycles per step (MCL)"=u64 1, "Scan freq.  increment (MCL)"=w5498, "1D or 2D Scan?"=w5518, "MCL Scan Axis"=w5518, "Cont. Scan (MCL)"=w5518, "MCL count"=w5505) -> ("FPGA VI Reference Out"=w5520:T13, "error out"=w5519:errorcluster)
            n845 = xnode "Read/Write Control"("FPGA VI Reference In"=w5520, "error in"=w5519, "AI to FIFO"=w5523, "APD to FIFO"=w5523, "Start scan"=w5523, "Start scan (MCL)"=w5523) -> ("FPGA VI Reference Out"=w5525:T13, "error out"=w5524:errorcluster)
          }
        }
        "Raster Scanning..." <- TRUE ("Scanning...")
      }
    }
    n846 = Compound Arithmetic op=OR("Start MCL Scan", "Confocal Image", "Confocal Linescan") -> (w3931:bool)
    n847 = And(x="Save Data (MCL)", y=w3931) -> (x .and. y?=w3981:bool)
    n848 = case "Start MCL raster scan" shown="True" w3931 {
      tunnel: w3984 -> [w4589 w4604]
      tunnel: w3983 -> [w4588 w4603]
      tunnel: [w4589 w4599] -> w3865
      tunnel: [w4588 w4598] -> w3864
      tunnel: [FALSE w4597] -> w3967
      tunnel: "Start MCL Scan" -> [_ w4592]
      tunnel: "Confocal Image" -> [_ w4591]
      tunnel: "Confocal Linescan" -> [_ _]
      frame #0 {
      }
      frame #1 {
        w4597 = TRUE
        n849 = case shown="True" "Restart DMA? (MCL)" {
          tunnel: [w4839 w4842] -> w4602
          tunnel: [w4838 w4841] -> w4601
          tunnel: w4604 -> [w4839 w4847]
          tunnel: w4603 -> [w4838 w4846]
          frame #0 {
          }
          frame #1 {
            w4843 = FALSE ("AI to FIFO")
            n850 = xnode "Read/Write Control"("FPGA VI Reference In"=w4847, "error in"=w4846, "AI to FIFO"=w4843, "APD to FIFO"=w4843) -> ("FPGA VI Reference Out"=w4845:T13, "error out"=w4844:errorcluster)
            n851 = xnode "Invoke Method"("FPGA VI Reference In"=w4845, "error in"=w4844) -> ("FPGA VI Reference Out"=w4849:T13, "error out"=w4848:errorcluster)
            n852 = xnode "Invoke Method"("FPGA VI Reference In"=w4849, "error in"=w4848) -> ("FPGA VI Reference Out"=w4842:T13, "error out"=w4841:errorcluster)
            n853 = local write "Overflow (data lost)"(FALSE ("Overflow (data lost)")) -> ()
          }
        }
        n854 = case shown="False" w4592 {
          selector: w4592 -> [_ w4608]
          tunnel: w4591 -> [w4607 _]
          tunnel: [w4607 w4608] -> w4590
          frame #0 {
            n855 = property on="2D or 1D Scan" class="Bool (strict)"("Val(Sgnl)"=w4607) -> ()  [unwired: 2 in, 2 out]
            n856 = property on="Confocal Image" class="Bool (strict)"("Value"=FALSE ("Start Confocal Map")) -> ()  [unwired: 2 in, 2 out]
          }
          frame #1 {
          }
        }
        n857 = local write "MCL Scanning"(w4597) -> ()
        n858 = local read "AO1"() -> (w4594:dbl)
        n859 = local read "AO2"() -> (w4593:dbl)
        n860 = case shown="True" "Center Scan" {
          tunnel: w4602 -> [w4615 w4722]
          tunnel: w4601 -> [w4614 w4721]
          tunnel: [w4613 w4720] -> w4599
          tunnel: [w4612 w4719] -> w4598
          tunnel: [w4610 w4701] -> w4596
          tunnel: [w4609 w4700] -> w4595
          tunnel: w4594 -> [w4610 w4711]
          tunnel: w4593 -> [w4609 w4714]
          tunnel: w4590 -> [_ _]
          frame #0 {
            w4611 = TRUE ("AI to FIFO")
            n861 = xnode "Read/Write Control"("FPGA VI Reference In"=w4615, "error in"=w4614, "AI to FIFO"=w4611, "APD to FIFO"=w4611, "Start scan (MCL)"=w4611) -> ("FPGA VI Reference Out"=w4613:T13, "error out"=w4612:errorcluster)
          }
          frame #1 {
            w4718 = TRUE ("AI to FIFO")
            n862 = local read "Scan steps (MCL)"() -> (w4707:u64)
            n863 = local read "Fast Scan Dir"() -> (w4699:bool)
            n864 = local read "Scan Range (V)"() -> (w4703:dbl)
            n865 = local read "Scan lines"() -> (w4706:u64)
            n866 = Divide(x=w4706, y=w4707) -> (x/y=w4705:dbl)
            n867 = Multiply(x=w4703, y=w4705) -> (x*y=w4704:dbl)
            n868 = Divide(x=w4704, y=2.0) -> (x/y=w4696:dbl)
            n869 = Divide(x=w4703, y=2.0) -> (x/y=w4695:dbl)
            n870 = Select(t=w4695, s=w4699, f=w4696) -> (s? t:f=w4694:dbl)
            n871 = Select(t=w4696, s=w4699, f=w4695) -> (s? t:f=w4698:dbl)
            n872 = Subtract(x=w4711, y=w4698) -> (x-y=w4697:dbl)
            n873 = Subtract(x=w4714, y=w4694) -> (x-y=w4693:dbl)
            n874 = local read "2D or 1D Scan"() -> (w4716:bool)
            n875 = Not(x=w4699) -> (.not. x?=w4710:bool)
            n876 = Not(x=w4716) -> (.not. x?=w4712:bool)
            n877 = And(x=w4699, y=w4712) -> (x .and. y?=w4713:bool)
            n878 = And(x=w4712, y=w4710) -> (x .and. y?=w4715:bool)
            n879 = Select(t=w4714, s=w4715, f=w4693) -> (s? t:f=w4700:dbl)
            n880 = Select(t=w4711, s=w4713, f=w4697) -> (s? t:f=w4701:dbl)
            n881 = call "Volt to I16.vi"("Voltage In"=w4701) -> ("I16 Voltage Out"=w4709:i16)
            n882 = call "Volt to I16.vi"("Voltage In"=w4700) -> ("I16 Voltage Out"=w4708:i16)
            n883 = xnode "Read/Write Control"("FPGA VI Reference In"=w4722, "error in"=w4721, "AI to FIFO"=w4718, "APD to FIFO"=w4718, "Start scan (MCL)"=w4718, "AO1"=w4709, "AO2"=w4708) -> ("FPGA VI Reference Out"=w4720:T13, "error out"=w4719:errorcluster)
          }
        }
        "Initial Y" <- w4596
        "Initial X" <- w4595
        "wait to reset values" <- w4597
      }
    }
    n884 = local read "APD Elements/DMA read"() -> (w3833:u32)
    n885 = local read "Elements/DMA read"() -> (w3889:u32)
    n886 = xnode "Get APD Data"("FPGA VI Reference In"=w3865, "error in"=w3864, "Number of Elements"=w3833, "Timeout (ms)"=-1) -> ("Data"=w3832:u32[], "Elements Remaining"=→"APD FIFO Elements Remaining":u32)  [unwired: 2 out]
    n887 = xnode "Get Trap Data"("FPGA VI Reference In"=w3865, "error in"=w3864, "Number of Elements"=w3889, "Timeout (ms)"=-1 ("Timeout")) -> ("FPGA VI Reference Out"=w3867:T13, "error out"=w3866:errorcluster, "Data"=w4007:u32[], "Elements Remaining"=w4037:u32)
    "FIFO El. Rem." <- w4037
    n888 = local read "FIFO Depth"() -> (w4039:u32)
    n889 = Subtract(x=w4039, y=w3889) -> (x-y=w4038:u32)
    n890 = Divide(x=w4037, y=w4038) -> (x/y=w4036:dbl)
    "Buffer Status" <- w4036
    n891 = Equal?(x=w4036, y=1.0) -> (x = y?=w4034:bool)
    n892 = case "Alert buffer overflow" shown="True" w4034 {
      frame #0 {
      }
      frame #1 {
        n893 = call <vilib>:"Beep.vi"() -> ()  [unwired: 3 in, 9 out]
        "Overflow (data lost)" <- TRUE ("Overflow (data lost)")
      }
    }
    n894 = local read "FPGA Averaging"() -> (w3888:bool)
    n895 = case "Special unpacking case if no averaging done by FPGA" shown="False" w3888 {
      tunnel: w4007 -> [w4999 w5025]
      tunnel: [w4970 w5000] -> w4006
      frame #0 {
        n896 = Decimate 1D Array(w4999) -> (w4998:u32[], w4997:u32[], w4996:u32[], w4995:u32[])
        n897 = Split Number(x=w4998) -> (hi(x)=w4994:u16[], lo(x)=w4993:u16[])
        n898 = Split Number(x=w4997) -> (hi(x)=w4992:u16[], lo(x)=w4991:u16[])
        n899 = Split Number(x=w4996) -> (hi(x)=w4990:u16[], lo(x)=w4989:u16[])
        n900 = Split Number(x=w4995) -> (hi(x)=w4988:u16[], lo(x)=w4987:u16[])
        n901 = To Word Integer(number=w4994) -> (16bit integer=w4986:i16[])
        n902 = To Word Integer(number=w4993) -> (16bit integer=w4985:i16[])
        n903 = To Word Integer(number=w4992) -> (16bit integer=w4984:i16[])
        n904 = To Word Integer(number=w4991) -> (16bit integer=w4983:i16[])
        n905 = To Word Integer(number=w4990) -> (16bit integer=w4982:i16[])
        n906 = To Word Integer(number=w4989) -> (16bit integer=w4981:i16[])
        n907 = To Word Integer(number=w4988) -> (16bit integer=w4980:i16[])
        n908 = To Word Integer(number=w4987) -> (16bit integer=w4979:i16[])
        n909 = To Double Precision Float(number=w4986) -> (double precision float=w4978:dbl[])
        n910 = To Double Precision Float(number=w4985) -> (double precision float=w4977:dbl[])
        n911 = To Double Precision Float(number=w4984) -> (double precision float=w4976:dbl[])
        n912 = To Double Precision Float(number=w4983) -> (double precision float=w4975:dbl[])
        n913 = To Double Precision Float(number=w4982) -> (double precision float=w4974:dbl[])
        n914 = To Double Precision Float(number=w4981) -> (double precision float=w4973:dbl[])
        n915 = To Double Precision Float(number=w4980) -> (double precision float=w4972:dbl[])
        n916 = To Double Precision Float(number=w4979) -> (double precision float=w4971:dbl[])
        n917 = Interleave 1D Arrays(w4978, w4977, w4976, w4975, w4974, w4973, w4972, w4971) -> (w4970:dbl[])
      }
      frame #1 {
        n918 = Decimate 1D Array(w5025) -> (w5016:u32[], w5014:u32[], w5012:u32[], w5010:u32[], w5008:u32[], w5006:u32[], w5004:u32[], w5002:u32[])
        n919 = To Long Integer(number=w5016) -> (32bit integer=w5024:i32[])
        n920 = To Long Integer(number=w5014) -> (32bit integer=w5023:i32[])
        n921 = To Long Integer(number=w5012) -> (32bit integer=w5022:i32[])
        n922 = To Long Integer(number=w5010) -> (32bit integer=w5021:i32[])
        n923 = To Long Integer(number=w5008) -> (32bit integer=w5020:i32[])
        n924 = To Long Integer(number=w5006) -> (32bit integer=w5019:i32[])
        n925 = To Long Integer(number=w5004) -> (32bit integer=w5018:i32[])
        n926 = To Long Integer(number=w5002) -> (32bit integer=w5017:i32[])
        n927 = To Double Precision Float(number=w5024) -> (double precision float=w5015:dbl[])
        n928 = To Double Precision Float(number=w5023) -> (double precision float=w5013:dbl[])
        n929 = To Double Precision Float(number=w5022) -> (double precision float=w5011:dbl[])
        n930 = To Double Precision Float(number=w5021) -> (double precision float=w5009:dbl[])
        n931 = To Double Precision Float(number=w5020) -> (double precision float=w5007:dbl[])
        n932 = To Double Precision Float(number=w5019) -> (double precision float=w5005:dbl[])
        n933 = To Double Precision Float(number=w5018) -> (double precision float=w5003:dbl[])
        n934 = To Double Precision Float(number=w5017) -> (double precision float=w5001:dbl[])
        n935 = Interleave 1D Arrays(w5015, w5013, w5011, w5009, w5007, w5005, w5003, w5001) -> (w5000:dbl[])
      }
    }
    n936 = local read "FPGA Ave."() -> (w3887:dbl)
    n937 = feedback #4(i16 -1 ("Trap Sets")) -> (w3885:i16)
    n938 = feedback #5("" ("Detector Type")) -> (w3882:string)
    n939 = Not Equal?(x=w3882, y="Detector Type") -> (x != y?=w3880:bool)
    n940 = local read "Trap Sets"() -> (w3884:i16)
    n941 = Not Equal?(x=w3885, y=w3884) -> (x != y?=w3879:bool)
    n942 = Or(x=w3880, y=w3879) -> (x .or. y?=w3878:bool)
    n943 = Divide(x=w4006, y=w3887) -> (x/y=w4014:dbl[])
    n944 = case "Deinterlace trap data, average down PSD" shown="1, Default" w3884 {
      tunnel: w4014 -> [w5044 w5109]
      tunnel: [w5041 w5106] -> w3872
      tunnel: [w5044 w5108] -> w4013
      tunnel: "Detector Type" -> [w5043 w5104]
      tunnel: [w5042 w5107] -> w3869
      tunnel: [w5040 w5105] -> w4005
      frame #0 {
        n945 = Divide(x=w5044, y=3276.7) -> (x/y=w5045:dbl[])
        n946 = Decimate 1D Array(w5045) -> (w5054:dbl[], w5053:dbl[], w5052:dbl[], w5051:dbl[], w5050:dbl[], w5049:dbl[], w5048:dbl[], w5047:dbl[])
        n947 = case shown="\"IR-QPD + PSD + FB-QPD position\"" w5043 {
          tunnel: w5054 -> [w5078 w5103]
          tunnel: w5053 -> [w5077 w5102]
          tunnel: w5052 -> [w5062 w5080]
          tunnel: w5051 -> [w5063 w5090]
          tunnel: w5050 -> [w5076 w5101]
          tunnel: w5049 -> [w5075 w5100]
          tunnel: w5048 -> [w5059 w5081]
          tunnel: w5047 -> [w5058 w5079]
          tunnel: [w5057 w5087] -> w5042
          tunnel: [w5056 w5086] -> w5041
          tunnel: [w5055 w5085] -> w5040
          frame #0 {
            w5055 = 0  # Channel pattern
            n948 = Divide(x=w5078, y=w5063) -> (x/y=w5065:dbl[])
            n949 = Divide(x=w5077, y=w5063) -> (x/y=w5064:dbl[])
            n950 = Divide(x=w5076, y=w5059) -> (x/y=w5061:dbl[])
            n951 = Divide(x=w5075, y=w5058) -> (x/y=w5060:dbl[])
            n952 = Build Array(w5065, w5064, w5063, w5062, w5061, w5060, w5059, w5058) -> (w5056:dbl[][])
            n953 = Bundle("T1 Y", "T1 X", "T1 Sum", "FB Sum", "PSD Y", "PSD X", "PSD Y Sum", "PSD X Sum") -> (w5074:T32)  [unwired: 1 out]
            n954 = Cluster To Array(cluster=w5074) -> (array=w5057:string[])
          }
          frame #1 {
            w5085 = 3  # Channel pattern
            n955 = Negate(x=w5081) -> (-x=w5082:dbl[])
            n956 = Divide(x=w5103, y=w5090) -> (x/y=w5092:dbl[])
            n957 = Divide(x=w5102, y=w5090) -> (x/y=w5091:dbl[])
            n958 = Divide(x=w5101, y=w5081) -> (x/y=w5089:dbl[])
            n959 = Divide(x=w5100, y=w5082) -> (x/y=w5088:dbl[])
            n960 = Build Array(w5092, w5091, w5090, w5079, w5080, w5089, w5088, w5081) -> (w5086:dbl[][])
            n961 = Bundle("T1 Y", "T1 X", "T1 Sum", "FB X", "FB Sum", "PSD Y", "PSD X", "PSD Y Sum") -> (w5099:T32)  [unwired: 1 out]
            n962 = Cluster To Array(cluster=w5099) -> (array=w5087:string[])
          }
        }
      }
      frame #1 {
        n963 = case shown="\"IR-QPD + PSD + FB-QPD X position\"" w5104 {
          tunnel: w5109 -> [w5170 w5237 w5307]
          tunnel: [w5150 w5222 w5294] -> w5108
          tunnel: [w5136 w5213 w5285] -> w5107
          tunnel: [w5135 w5173 w5252] -> w5106
          tunnel: [w5129 w5211 w5283] -> w5105
          frame #0 {
            w5129 = 1  # Channel pattern
            # "time average x2 the 4th signal and the 4 psd signals (detection laser)"
            # "deinterlace 3 signals from qpd"
            n964 = Decimate 1D Array(w5170) -> (w5169:dbl[], w5168:dbl[], w5134:dbl[], w5167:dbl[], w5157:dbl[], w5155:dbl[], w5154:dbl[], w5152:dbl[])
            n965 = Decimate 1D Array(w5134) -> (w5133:dbl[], w5132:dbl[])
            n966 = Decimate 1D Array(w5169) -> (w5166:dbl[], w5138:dbl[])
            n967 = Decimate 1D Array(w5168) -> (w5165:dbl[], w5163:dbl[])
            n968 = Decimate 1D Array(w5167) -> (w5164:dbl[], w5162:dbl[])
            n969 = call "downsample 1D array - double.vi"("Ave N"=2.0, "Array In"=w5157) -> ("Array Out"=w5156:dbl[])  [unwired: 1 out]
            n970 = call "downsample 1D array - double.vi"("Ave N"=2.0, "Array In"=w5155) -> ("Array Out"=w5137:dbl[])  [unwired: 1 out]
            n971 = call "downsample 1D array - double.vi"("Ave N"=2.0, "Array In"=w5154) -> ("Array Out"=w5153:dbl[])  [unwired: 1 out]
            n972 = call "downsample 1D array - double.vi"("Ave N"=2.0, "Array In"=w5152) -> ("Array Out"=w5151:dbl[])  [unwired: 1 out]
            n973 = Interleave 1D Arrays(w5166, w5165, w5164, w5138, w5163, w5162, w5133, w5132, w5156, w5137, w5153, w5151) -> (w5150:dbl[])
            n974 = Divide(x=w5150, y=3276.7) -> (x/y=w5149:dbl[])
            n975 = Decimate 1D Array(w5149) -> (w5148:dbl[], w5147:dbl[], w5146:dbl[], w5145:dbl[], w5144:dbl[], w5143:dbl[], w5131:dbl[], w5130:dbl[], w5142:dbl[], w5141:dbl[], w5140:dbl[], w5139:dbl[])
            n976 = Divide(x=w5148, y=w5146) -> (x/y=w5116:dbl[])
            n977 = Divide(x=w5147, y=w5146) -> (x/y=w5115:dbl[])
            n978 = Divide(x=w5145, y=w5143) -> (x/y=w5114:dbl[])
            n979 = Divide(x=w5144, y=w5143) -> (x/y=w5113:dbl[])
            n980 = Divide(x=w5142, y=w5140) -> (x/y=w5112:dbl[])
            n981 = Divide(x=w5141, y=w5139) -> (x/y=w5111:dbl[])
            n982 = Build Array(w5116, w5115, w5146, w5114, w5113, w5143, w5131, w5130, w5112, w5111, w5140, w5139) -> (w5135:dbl[][])
            n983 = Bundle("T1 Y", "T1 X", "T1 Sum", "T2 Y", "T2 X", "T2 Sum", "T1 FB Sum", "T2 FB Sum", "PSD Y", "PSD X", "PSD Y Sum", "PSD X Sum") -> (w5117:T33)  [unwired: 1 out]
            n984 = Cluster To Array(cluster=w5117) -> (array=w5136:string[])
          }
          frame #1 {
            w5211 = 2  # Channel pattern
            # "time average x2 the 3 psd signals (detection laser)"
            # "deinterlace 3 signals from qpds"
            n985 = Decimate 1D Array(w5237) -> (w5236:dbl[], w5235:dbl[], w5212:dbl[], w5234:dbl[], w5225:dbl[], w5224:dbl[], w5223:dbl[], w5199:dbl[])
            n986 = Decimate 1D Array(w5212) -> (w5194:dbl[], w5192:dbl[])
            n987 = Decimate 1D Array(w5236) -> (w5233:dbl[], w5214:dbl[])
            n988 = Decimate 1D Array(w5235) -> (w5232:dbl[], w5230:dbl[])
            n989 = Decimate 1D Array(w5234) -> (w5231:dbl[], w5229:dbl[])
            n990 = Decimate 1D Array(w5199) -> (w5195:dbl[], w5193:dbl[])
            n991 = call "downsample 1D array - double.vi"("Ave N"=2.0, "Array In"=w5225) -> ("Array Out"=w5198:dbl[])  [unwired: 1 out]
            n992 = call "downsample 1D array - double.vi"("Ave N"=2.0, "Array In"=w5224) -> ("Array Out"=w5197:dbl[])  [unwired: 1 out]
            n993 = call "downsample 1D array - double.vi"("Ave N"=2.0, "Array In"=w5223) -> ("Array Out"=w5196:dbl[])  [unwired: 1 out]
            n994 = Interleave 1D Arrays(w5233, w5232, w5231, w5214, w5230, w5229, w5195, w5194, w5193, w5192, w5198, w5197, w5196) -> (w5222:dbl[])
            n995 = Divide(x=w5222, y=3276.7) -> (x/y=w5221:dbl[])
            n996 = Decimate 1D Array(w5221) -> (w5220:dbl[], w5219:dbl[], w5218:dbl[], w5217:dbl[], w5216:dbl[], w5215:dbl[], w5184:dbl[], w5182:dbl[], w5181:dbl[], w5179:dbl[], w5178:dbl[], w5177:dbl[], w5174:dbl[])
            n997 = Negate(x=w5174) -> (-x=w5172:dbl[])
            n998 = Divide(x=w5178, y=w5174) -> (x/y=w5176:dbl[])
            n999 = Divide(x=w5177, y=w5172) -> (x/y=w5175:dbl[])
            n1000 = Divide(x=w5220, y=w5218) -> (x/y=w5203:dbl[])
            n1001 = Divide(x=w5219, y=w5218) -> (x/y=w5202:dbl[])
            n1002 = Divide(x=w5217, y=w5215) -> (x/y=w5201:dbl[])
            n1003 = Divide(x=w5216, y=w5215) -> (x/y=w5200:dbl[])
            n1004 = Divide(x=w5184, y=w5182) -> (x/y=w5183:dbl[])
            n1005 = Divide(x=w5181, y=w5179) -> (x/y=w5180:dbl[])
            n1006 = Build Array(w5203, w5202, w5218, w5201, w5200, w5215, w5183, w5182, w5180, w5179, w5176, w5175, w5174) -> (w5173:dbl[][])
            n1007 = Bundle("T1 Y", "T1 X", "T1 Sum", "T2 Y", "T2 X", "T2 Sum", "T1 FB X", "T1 FB Sum", "T2 FB X", "T2 FB Sum", "PSD Y", "PSD X", "PSD Y Sum") -> (w5204:T34)  [unwired: 1 out]
            n1008 = Cluster To Array(cluster=w5204) -> (array=w5213:string[])
          }
          frame #2 {
            w5283 = 4  # Channel pattern
            # "time average x2 the 3 psd signals (detection laser)"
            # "deinterlace 3 signals from qpds"
            n1009 = Decimate 1D Array(w5307) -> (w5306:dbl[], w5305:dbl[], w5284:dbl[], w5304:dbl[], w5250:dbl[], w5296:dbl[], w5295:dbl[], w5272:dbl[])
            n1010 = Decimate 1D Array "Feedback Sum"(w5284) -> (w5268:dbl[], w5266:dbl[])
            n1011 = Decimate 1D Array "QPD Y"(w5306) -> (w5303:dbl[], w5286:dbl[])
            n1012 = Decimate 1D Array "QPD X"(w5305) -> (w5302:dbl[], w5300:dbl[])
            n1013 = Decimate 1D Array "Feedback Y"(w5250) -> (w5249:dbl[], w5248:dbl[])
            n1014 = Decimate 1D Array "QPD Sum"(w5304) -> (w5301:dbl[], w5299:dbl[])
            n1015 = Decimate 1D Array "Feedback X"(w5272) -> (w5269:dbl[], w5267:dbl[])
            n1016 = call "downsample 1D array - double.vi"("Ave N"=2.0, "Array In"=w5296) -> ("Array Out"=w5271:dbl[])  [unwired: 1 out]
            n1017 = call "downsample 1D array - double.vi"("Ave N"=2.0, "Array In"=w5295) -> ("Array Out"=w5270:dbl[])  [unwired: 1 out]
            n1018 = Interleave 1D Arrays(w5303, w5302, w5301, w5286, w5300, w5299, w5249, w5269, w5268, w5248, w5267, w5266, w5271, w5270) -> (w5294:dbl[])
            n1019 = Divide(x=w5294, y=3276.7) -> (x/y=w5293:dbl[])
            n1020 = Decimate 1D Array(w5293) -> (w5292:dbl[], w5291:dbl[], w5290:dbl[], w5289:dbl[], w5288:dbl[], w5287:dbl[], w5245:dbl[], w5259:dbl[], w5243:dbl[], w5244:dbl[], w5257:dbl[], w5241:dbl[], w5255:dbl[], w5253:dbl[])
            n1021 = Negate(x=w5253) -> (-x=w5251:dbl[])
            n1022 = Divide(x=w5255, y=w5251) -> (x/y=w5254:dbl[])
            n1023 = Divide(x=w5244, y=w5241) -> (x/y=w5240:dbl[])
            n1024 = Divide(x=w5245, y=w5243) -> (x/y=w5242:dbl[])
            n1025 = Divide(x=w5292, y=w5290) -> (x/y=w5276:dbl[])
            n1026 = Divide(x=w5291, y=w5290) -> (x/y=w5275:dbl[])
            n1027 = Divide(x=w5289, y=w5287) -> (x/y=w5274:dbl[])
            n1028 = Divide(x=w5288, y=w5287) -> (x/y=w5273:dbl[])
            n1029 = Divide(x=w5259, y=w5243) -> (x/y=w5258:dbl[])
            n1030 = Divide(x=w5257, y=w5241) -> (x/y=w5256:dbl[])
            n1031 = Build Array(w5276, w5275, w5290, w5274, w5273, w5287, w5242, w5258, w5243, w5240, w5256, w5241, w5254, w5253) -> (w5252:dbl[][])
            n1032 = Bundle("T1 Y", "T1 X", "T1 Sum", "T2 Y", "T2 X", "T2 Sum", "T1 FB Y", "T1 FB X", "T1 FB Sum", "T2 FB Y", "T2 FB X", "T2 FB Sum", "PSD X", "PSD Y Sum") -> (w5239:T35)  [unwired: 1 out]
            n1033 = Cluster To Array(cluster=w5239) -> (array=w5285:string[])
          }
        }
      }
    }
    n1034 = case "Update these things only if detector type or number of traps changes" shown="True" w3878 {
      tunnel: w3869 -> [_ w4160]
      frame #0 {
      }
      frame #1 {
        n1035 = property on="High Res. Display" class="Ring (strict)"("Strings []"=w4160) -> ()  [unwired: 2 in, 2 out]
        n1036 = Build Array (concatenate)(w4160, "none") -> (w4153:string[])
        n1037 = property on="FFT 1 Choice 1" class="Ring (strict)"("Strings []"=w4153) -> ()  [unwired: 2 in, 2 out]
        n1038 = property on="FFT 1 Choice 2" class="Ring (strict)"("Strings []"=w4153) -> ()  [unwired: 2 in, 2 out]
        n1039 = property on="FFT 2 Choice 1" class="Ring (strict)"("Strings []"=w4153) -> ()  [unwired: 2 in, 2 out]
        n1040 = property on="FFT 2 Choice 2" class="Ring (strict)"("Strings []"=w4153) -> ()  [unwired: 2 in, 2 out]
        n1041 = Bundle("APD 1", "APD 2") -> (w4156:cluster{string, string})  [unwired: 1 out]
        n1042 = Cluster To Array(cluster=w4156) -> (array=w4154:string[])
        n1043 = Build Array (concatenate)(w4154, w4153) -> (w4158:string[])
        n1044 = Array Size(array=w4158) -> (size(s)=w4159:i32)
        n1045 = property on="Signals to Plot" class="LstBox (strict)"("Item Names"=w4158) -> ()  [unwired: 2 in, 2 out]
        n1046 = property on="Signals to Plot" class="LstBox (strict)"("Number of Rows"=w4159) -> ()  [unwired: 2 in, 2 out]
        n1047 = property on="All Signals" class="WFChart (strict)"("LegNumRows"=w4159) -> ()  [unwired: 2 in, 2 out]
      }
    }
    n1048 = local read "Data points/scans (MCL)"() -> (w3976:dbl)
    n1049 = Increment(x=w3976) -> (x+1=w3977:dbl)
    n1050 = feedback #6(w3977) -> (w3980:dbl)
    n1051 = Select(t=0, s=w3967, f=w3980) -> (s? t:f=w3973:dbl)
    n1052 = To Word Integer(number=w4013) -> (16bit integer=w4040:i16[])
    n1053 = Decimate 1D Array(w3832) -> (w3863:u32[], w4003:u32[])
    n1054 = To Double Precision Float(number=w3863) -> (double precision float=w3862:dbl[])
    n1055 = Array Size(array=w3862) -> (size(s)=w3979:i32)
    n1056 = Add(x=w3979, y=w3973) -> (x+y=w3974:dbl)
    n1057 = Greater?(x=w3974, y=w3976) -> (0:w3975:bool)
    n1058 = local read "DMA Update Period (s)"() -> (w3891:dbl)
    n1059 = Select(t=w3973, s=w3975, f=w3974) -> (s? t:f=w3972:dbl)
    n1060 = Build Array(w3863, w4003) -> (w3964:u32[][])
    n1061 = local read "MCL Scanning"() -> (w3970:bool)
    n1062 = local read "Data Period (s)"() -> (w3848:dbl)
    n1063 = To Double Precision Float(number=w3964) -> (double precision float=w3965:dbl[][])
    n1064 = Not(x=w3975) -> (.not. x?=w3969:bool)
    n1065 = local read "APD Integration Time (s)"() -> (w3890:dbl)
    n1066 = And(x=w3969, y=w3970) -> (x .and. y?=w3971:bool)
    n1067 = feedback #7(0.0) -> (w4000:dbl)
    n1068 = Add(x=w3891, y=w4000) -> (x+y=w4009:dbl)
    n1069 = Or(x=w3971, y=w3967) -> (x .or. y?=w3968:bool)
    n1070 = Multiply(x=w3848, y="Trap Disp. Downsample") -> (x*y=w3846:dbl)
    "Display Period (s)" <- w3846
    n1071 = Equal?(x="Tab Control 6", y=T1."High Res Display") -> (x = y?=w3875:bool)
    n1072 = for {
      tunnel: [w5039] -> w3999 mode=indexing
      tunnel: w4000 -> [w5038]
      tunnel: "Trap Disp. Downsample" -> [w5035]
      tunnel: w3872 -> [w5033] mode=indexing
      tunnel: w3848 -> [w5032]
      tunnel: w3869 -> [w5031] mode=indexing
      tunnel: w3871 -> [w5030]
      tunnel: [w5029] -> w3870 mode=indexing
      tunnel: w3846 -> [w5028]
      n1073 = Bundle By Name("Y"=w5033, "dt"=w5032) -> (w5034:waveform(dbl))  [unwired: 1 out]
      n1074 = Set Waveform Attribute(5:w5031, 6:w5030, 7:w5034) -> (3:w5029:waveform(dbl))  [unwired: 1 in, 2 out]
      n1075 = call "downsample 1D array - double.vi"("Ave N"=w5035, "Array In"=w5033) -> ("Array Out"=w5036:dbl[])  [unwired: 1 out]
      n1076 = To Time Stamp(1:w5038) -> (0:w5037:timestamp)
      n1077 = Bundle By Name(cluster=w5029, "t0"=w5037, "Y"=w5036, "dt"=w5028) -> (w5039:waveform(dbl))
    }
    n1078 = case "For computing FFTs for display" shown="True" "Compute FFT" {
      tunnel: w3870 -> [_ w5923]
      frame #0 {
      }
      frame #1 {
        n1079 = Build Array("FFT 1 Choice 1", "FFT 1 Choice 2", "FFT 2 Choice 1", "FFT 2 Choice 2") -> (w5916:u16[])
        n1080 = Array Size(array=w5923) -> (size(s)=w5922:i32)
        n1081 = feedback #8(u16[] [100, 100, 100, 100]) -> (w5917:u16[])
        n1082 = feedback #9("# Spectra to Ave.") -> (w5914:dbl)
        n1083 = Not Equal?(x="# Spectra to Ave.", y=w5914) -> (x != y?=w5913:bool)
        n1084 = Not Equal?(x=w5916, y=w5917) -> (x != y?=w5915:bool)
        n1085 = feedback #10(1.0) -> (w5900:dbl)
        n1086 = Compound Arithmetic op=OR("Reset FFT", w5915, w5913) -> (w5898:bool)
        n1087 = Select(t=1.0, s=w5898, f=w5900) -> (s? t:f=w5902:dbl)
        n1088 = Greater?(x=w5902, y="# Spectra to Ave.") -> (0:w5921:bool)
        n1089 = Increment(x=w5902) -> (x+1=w5901:dbl)
        n1090 = local read "DMA Update Period (s)"() -> (w5896:dbl)
        n1091 = Multiply(x="# Spectra to Ave.", y=w5896) -> (x*y=→"Ave. Time (s)":dbl)
        n1092 = Build Array(cluster{"f0":dbl, "df":dbl, "magnitude":dbl[]} {"f0"=0.0, "df"=0.0, "magnitude"=[]} ("PSD")) -> (w5905:cluster{"f0":dbl, "df":dbl, "magnitude":dbl[]}[])
        n1093 = Build Array(w5905, w5905, w5905, w5905) -> (w5907:T36)
        n1094 = feedback #11(w5907) -> (w5912:T36)
        n1095 = for {
          N: 4 -> [_]
          tunnel: w5916 -> [w5945] mode=indexing
          tunnel: w5923 -> [w5946]
          tunnel: w5922 -> [w5948]
          tunnel: w5898 -> [w5941]
          tunnel: w5921 -> [w5940]
          tunnel: "# Spectra to Ave." -> [w5939]
          tunnel: [w5938] -> w5911 mode=indexing
          tunnel: w5912 -> [w5943] mode=indexing
          tunnel: [w5942] -> w5899 mode=indexing
          tunnel: w5902 -> [w5937]
          n1096 = Less?(x=w5945, y=w5948) -> (x < y?=w5947:bool)
          n1097 = Index Array(array=w5946, index=w5945) -> (element=w5944:waveform(dbl))
          n1098 = case shown="True" w5947 {
            tunnel: w5944 -> [_ w5965]
            tunnel: w5943 -> [w5950 w5963]
            tunnel: [w5950 w5951] -> w5942
            tunnel: w5941 -> [_ w5962]
            tunnel: w5940 -> [_ w5955]
            tunnel: w5939 -> [_ w5954]
            tunnel: [cluster{"f0":dbl, "df":dbl, "magnitude":dbl[]} {"f0"=0.0, "df"=0.0, "magnitude"=[]} ("PSD") w5956] -> w5938
            tunnel: w5937 -> [_ w5953]
            frame #0 {
            }
            frame #1 {
              n1099 = call <vilib>:"Std Deviation and Variance.vi"("X"=w5965) -> ("mean"=w5966:dbl)  [unwired: 1 in, 2 out]
              n1100 = Subtract(x=w5965, y=w5966) -> (x-y=w5964:waveform(dbl))
              n1101 = xnode "Spectral Measurements"("Signals"=w5964) -> ("PSD"=w5958:cluster{"f0":dbl, "df":dbl, "magnitude":dbl[]})  [unwired: 1 in, 1 out]
              n1102 = case shown="False" w5962 {
                tunnel: w5963 -> [w5975 _]
                tunnel: [w5971 w5980] -> w5951
                tunnel: w5958 -> [w5974 w5981]
                tunnel: w5955 -> [w5973 _]
                frame #0 {
                  n1103 = Build Array (concatenate)(w5975, w5974) -> (w5972:cluster{"f0":dbl, "df":dbl, "magnitude":dbl[]}[])
                  n1104 = case shown="True" w5973 {
                    tunnel: w5972 -> [w5976 w5979]
                    tunnel: [w5976 w5977] -> w5971
                    frame #0 {
                    }
                    frame #1 {
                      n1105 = Delete From Array(array=w5979, index=0) -> (array with subset deleted=w5977:cluster{"f0":dbl, "df":dbl, "magnitude":dbl[]}[])  [unwired: 1 in, 1 out]
                    }
                  }
                }
                frame #1 {
                  n1106 = Build Array(w5981) -> (w5980:cluster{"f0":dbl, "df":dbl, "magnitude":dbl[]}[])
                }
              }
              n1107 = for {
                tunnel: w5951 -> [w5970] mode=indexing
                tunnel: [w5969] -> w5961 mode=indexing
                n1108 = Unbundle By Name(w5970) -> ("magnitude"=w5969:dbl[])
              }
              n1109 = Transpose 2D Array(2D array=w5961) -> (transposed array=w5960:dbl[][])
              n1110 = for {
                tunnel: w5960 -> [w5968] mode=indexing
                tunnel: [w5967] -> w5959 mode=indexing
                n1111 = Add Array Elements(numeric array=w5968) -> (sum=w5967:dbl)
              }
              n1112 = Select(t=w5954, s=w5955, f=w5953) -> (s? t:f=w5952:dbl)
              n1113 = Divide(x=w5959, y=w5952) -> (x/y=w5957:dbl[])
              n1114 = Bundle By Name(cluster=w5958, "magnitude"=w5957) -> (w5956:cluster{"f0":dbl, "df":dbl, "magnitude":dbl[]})
            }
          }
        }
        n1115 = case shown="True" w5898 {
          tunnel: w5899 -> [w5930 w5936]
          tunnel: [w5930 w5931] -> w5897
          frame #0 {
          }
          frame #1 {
            n1116 = Array Subset(array=w5936, index (row)=0 ("index"), length (row)=4 ("length"), index (col)=0 ("index"), length (col)=1 ("length")) -> (w5931:T36)
          }
        }
        n1117 = Split 1D Array(array=w5911, index=2) -> (first subarray=→"FFT 1":cluster{"f0":dbl, "df":dbl, "magnitude":dbl[]}[], second subarray=→"FFT 2":cluster{"f0":dbl, "df":dbl, "magnitude":dbl[]}[])
      }
    }
    n1118 = Reciprocal(x=w3846) -> (1/x=→"Trap Disp. Freq. (Hz)":dbl)
    n1119 = case shown="True" w3875 {
      tunnel: w3870 -> [_ w4129]
      frame #0 {
      }
      frame #1 {
        n1120 = Index Array(array=w4129, index="High Res. Display") -> (element=w4130:waveform(dbl))
        n1121 = call <vilib>:"Std Deviation and Variance.vi"("X"=w4130) -> ("mean"=w4137:dbl, "standard deviation"=w4142:dbl)  [unwired: 1 in, 1 out]
        "Mean Intensity" <- w4137
        "Sigma" <- w4142
        n1122 = Subtract(x=w4130, y=w4137) -> (x-y=w4136:waveform(dbl))
        n1123 = Select(t=w4136, s="Subtract mean", f=w4130) -> (s? t:f=→"1 Channel":waveform(dbl))
        n1124 = Divide(x=w4142, y=w4137) -> (x/y=→"Sigma/Mean":dbl)
        n1125 = feedback #12(1) -> (w4131:i32)
        n1126 = Greater Or Equal?(x=w4131, y="Slow mean N ave.") -> (x >= y?=w4144:bool)
        n1127 = Increment(x=w4131) -> (x+1=w4146:i32)
        n1128 = Select(t=1, s=w4144, f=w4146) -> (s? t:f=w4133:i32)
        n1129 = feedback #13() -> (w4134:waveform(dbl))  [unwired: 1 out]
        n1130 = case shown="Default" w4131 {
          tunnel: [w4149 w4152] -> w4135
          tunnel: w4134 -> [w4151 _]
          tunnel: w4130 -> [w4150 w4152]
          frame #0 {
            n1131 = call-poly <vilib>:"Append Waveforms.vi"("waveform B"=w4150, "waveform A"=w4151) -> ("waveform out"=w4149:waveform(dbl))  [unwired: 1 in, 8 out]
          }
          frame #1 {
          }
        }
        n1132 = case shown="True" w4144 {
          tunnel: w4135 -> [_ w4148]
          frame #0 {
          }
          frame #1 {
            n1133 = call <vilib>:"Mean.vi"("X"=w4148) -> ("mean"=→"Slow mean":dbl)  [unwired: 1 out]
          }
        }
      }
    }
    n1134 = Bundle("APD 1", "APD 2") -> (w3997:cluster{string, string})  [unwired: 1 out]
    n1135 = Cluster To Array(cluster=w3997) -> (array=w3994:string[])
    n1136 = for {
      tunnel: w3965 -> [w4959] mode=indexing
      tunnel: w4000 -> [w4968]
      tunnel: w3890 -> [w4967]
      tunnel: [w4963] -> w3998 mode=indexing
      tunnel: "APD Disp. Scale" -> [w4964]
      tunnel: w3871 -> [w4962]
      tunnel: w3994 -> [w4961] mode=indexing
      tunnel: "APD Disp. Downsample" -> [w4957]
      tunnel: [w4960] -> w3993
      n1137 = call "integrate 1D array interval - double.vi"("Ave N"=w4957, "Array In"=w4959) -> ("Array Out"=w4958:dbl[])  [unwired: 1 out]
      n1138 = Multiply(x=w4967, y=w4957) -> (x*y=w4960:dbl)
      n1139 = Divide(x=w4958, y=w4964) -> (x/y=w4965:dbl[])
      n1140 = To Time Stamp(1:w4968) -> (0:w4969:timestamp)
      n1141 = Bundle By Name("t0"=w4969, "Y"=w4965, "dt"=w4960) -> (w4966:waveform(dbl))  [unwired: 1 out]
      n1142 = Set Waveform Attribute(5:w4961, 6:w4962, 7:w4966) -> (3:w4963:waveform(dbl))  [unwired: 1 in, 2 out]
    }
    "APD Display Period (s)" <- w3993
    n1143 = Reciprocal(x=w3993) -> (1/x=→"APD Display Freq. (Hz)":dbl)
    n1144 = feedback #14(w3863) -> (w3963:u32[])
    n1145 = Build Array (concatenate)(w3963, w3863) -> (w3960:u32[])
    n1146 = Array Size(array=w3960) -> (size(s)=w3957:i32)
    n1147 = Array Size(array=w3863) -> (size(s)=w3959:i32)
    n1148 = Build Array (concatenate)(w3998, w3999) -> (w3892:waveform(dbl)[])
    "All Signals" <- w3892
    n1149 = case "For plotting results of scanning MCL" shown="True" w3968 {
      tunnel: w3967 -> [_ w4549]
      tunnel: w3862 -> [_ w4585]
      tunnel: w3976 -> [_ _]
      tunnel: w3892 -> [_ w4524]
      frame #0 {
      }
      frame #1 {
        n1150 = Index Array(array=w4524, index=13) -> (element=w4528:waveform(dbl))
        n1151 = Index Array(array=w4524, index=12) -> (element=w4532:waveform(dbl))
        n1152 = Index Array(array=w4524, index="Channel") -> (element=w4526:waveform(dbl))
        n1153 = Unbundle By Name(w4528) -> ("Y"=w4527:dbl[])
        n1154 = Unbundle By Name(w4532) -> ("Y"=w4531:dbl[])
        n1155 = Unbundle By Name(w4526) -> ("Y"=w4523:dbl[])
        n1156 = feedback #15(w4585) -> (w4586:dbl[])
        n1157 = Build Array (concatenate)(w4586, w4585) -> (w4534:dbl[])
        n1158 = Select(t=w4585, s=w4549, f=w4534) -> (s? t:f=w4543:dbl[])
        n1159 = feedback #16(w4531) -> (w4550:dbl[])
        n1160 = Build Array (concatenate)(w4550, w4531) -> (w4530:dbl[])
        n1161 = feedback #17(w4523) -> (w4583:dbl[])
        n1162 = Build Array (concatenate)(w4583, w4523) -> (w4582:dbl[])
        n1163 = feedback #18(w4527) -> (w4559:dbl[])
        n1164 = Build Array (concatenate)(w4559, w4527) -> (w4560:dbl[])
        n1165 = Select(t=w4531, s=w4549, f=w4530) -> (s? t:f=w4552:dbl[])
        n1166 = Select(t=w4523, s=w4549, f=w4582) -> (s? t:f=w4580:dbl[])
        n1167 = Select(t=w4527, s=w4549, f=w4560) -> (s? t:f=w4562:dbl[])
        n1168 = local read "N APD Samp/step"() -> (w4542:dbl)
        n1169 = Array Size(array=w4552) -> (size(s)=w4553:i32)
        n1170 = Array Size(array=w4580) -> (size(s)=w4579:i32)
        n1171 = Array Size(array=w4562) -> (size(s)=w4563:i32)
        n1172 = local read "Scan steps (MCL)"() -> (w4535:u64)
        n1173 = call "integrate 1D array interval - double.vi"("Ave N"=w4542, "Array In"=w4543) -> ("Array Out"=w4541:dbl[])  [unwired: 1 out]
        n1174 = local read "Scan lines"() -> (w4536:u64)
        n1175 = Array Size(array=w4541) -> (size(s)=w4548:i32)
        n1176 = Divide(x=w4553, y=w4548) -> (x/y=w4554:dbl)
        n1177 = call "downsample 1D array - double.vi"("Ave N"=w4554, "Array In"=w4552) -> ("Array Out"=w4556:dbl[])  [unwired: 1 out]
        n1178 = Divide(x=w4579, y=w4548) -> (x/y=w4578:dbl)
        n1179 = call "downsample 1D array - double.vi"("Ave N"=w4578, "Array In"=w4580) -> ("Array Out"=w4571:dbl[])  [unwired: 1 out]
        n1180 = Divide(x=w4563, y=w4548) -> (x/y=w4564:dbl)
        n1181 = call "downsample 1D array - double.vi"("Ave N"=w4564, "Array In"=w4562) -> ("Array Out"=w4566:dbl[])  [unwired: 1 out]
        n1182 = Multiply(x=w4535, y=u64 2) -> (x*y=w4546:u64)
        n1183 = Multiply(x=w4536, y=w4546) -> (x*y=w4576:u64)
        n1184 = Subtract(x=w4576, y=w4548) -> (x-y=w4547:u64)
        n1185 = call <vilib>:"Mean.vi"("X"=w4541) -> ("mean"=w4575:dbl)  [unwired: 1 out]
        n1186 = call <vilib>:"Mean.vi"("X"=w4556) -> ("mean"=w4555:dbl)  [unwired: 1 out]
        n1187 = call <vilib>:"Mean.vi"("X"=w4571) -> ("mean"=w4572:dbl)  [unwired: 1 out]
        n1188 = call <vilib>:"Mean.vi"("X"=w4566) -> ("mean"=w4565:dbl)  [unwired: 1 out]
        n1189 = Initialize Array(w4575, w4547) -> (w4574:dbl[])
        n1190 = Initialize Array(w4555, w4547) -> (w4557:dbl[])
        n1191 = Initialize Array(w4572, w4547) -> (w4570:dbl[])
        n1192 = Initialize Array(w4565, w4547) -> (w4567:dbl[])
        n1193 = Build Array (concatenate)(w4541, w4574) -> (w4573:dbl[])
        n1194 = Build Array (concatenate)(w4556, w4557) -> (w4558:dbl[])
        n1195 = Build Array (concatenate)(w4571, w4570) -> (w4569:dbl[])
        n1196 = Build Array (concatenate)(w4566, w4567) -> (w4568:dbl[])
        n1197 = Reshape Array(w4573, w4536, w4546) -> (w4539:dbl[][])
        n1198 = Reshape Array(w4558, w4536, w4546) -> (w4551:dbl[][])
        n1199 = Reshape Array(w4569, w4536, w4546) -> (w4581:dbl[][])
        n1200 = Reshape Array(w4568, w4536, w4546) -> (w4561:dbl[][])
        n1201 = Transpose 2D Array(2D array=w4551) -> (transposed array=→"PSD Y map":dbl[][])
        n1202 = Transpose 2D Array(2D array=w4581) -> (transposed array=→"Data map":dbl[][])
        n1203 = Transpose 2D Array(2D array=w4561) -> (transposed array=→"PSD X map":dbl[][])
        n1204 = Transpose 2D Array(2D array=w4539) -> (transposed array=→"APD 1 map":dbl[][])
        n1205 = Index Array(array=w4539, index (row)=0) -> (element=→"Waveform Graph":dbl[])  [unwired: 1 in]
      }
    }
    n1206 = local read "APD Integration Time (s)"() -> (w3823:dbl)
    n1207 = Multiply(x=w3959, y="APD Ave N") -> (x*y=w3958:dbl)
    n1208 = Greater?(x=w3957, y=w3958) -> (0:w3961:bool)
    n1209 = Index Array(array=w3892, index=0) -> (element=w3950:waveform(dbl))
    n1210 = case shown="True" w3961 {
      tunnel: w3960 -> [w4517 w4522]
      tunnel: [w4517 w4518] -> w3897
      tunnel: w3958 -> [_ w4520]
      tunnel: w3957 -> [_ w4521]
      frame #0 {
      }
      frame #1 {
        n1211 = Subtract(x=w4521, y=w4520) -> (x-y=w4519:dbl)
        n1212 = Array Subset(array=w4522, index=w4519, length=w4520) -> (w4518:u32[])
      }
    }
    n1213 = Multiply(x="APD Disp. Scale", y=w3950) -> (x*y=w3825:waveform(dbl))
    n1214 = Multiply(x="APD Disp. Downsample", y=w3823) -> (x*y=w3820:dbl)
    n1215 = Divide(x=w3825, y=w3820) -> (x/y=→"APD 1 Chart":waveform(dbl))
    n1216 = Index Array(array=w3892, index=3) -> (element=w3909:waveform(dbl))
    n1217 = Index Array(array=w3892, index=6) -> (element=w3906:waveform(dbl))
    n1218 = Array Size(array=w3897) -> (size(s)=w3955:i32)
    n1219 = Add Array Elements(numeric array=w3897) -> (sum=w3966:u32)
    n1220 = call <vilib>:"Std Deviation and Variance.vi"("X"=w3897) -> ("standard deviation"=w3896:dbl)  [unwired: 1 in, 2 out]
    n1221 = Divide(x="T1 offset_x (mV)", y=1000.0) -> (x/y=w3910:dbl)
    n1222 = Multiply(x=w3890, y=w3955) -> (x*y=w3956:dbl)
    "Int. Time (s)" <- w3956
    n1223 = Divide(x=w3966, y=w3956) -> (x/y=w3894:dbl)
    "APD 1 Rate (Hz)" <- w3894
    n1224 = Divide(x=w3896, y=w3890) -> (x/y=w3895:dbl)
    "Rate sigma (Hz)" <- w3895
    n1225 = Divide(x=w3895, y=w3894) -> (x/y=→"sigma/mean":dbl)
    n1226 = Divide(x="T2 offset_x (mV)", y=1000.0) -> (x/y=w3908:dbl)
    n1227 = case shown="0, Default" "Calibration" {
      tunnel: "T1 alpha_x (nm/V)" -> [_ w4494 w4515]
      tunnel: "T1 kappa_x (pN/nm)" -> [_ _ w4505]
      tunnel: "T2 alpha_x (nm/V)" -> [_ w4493 w4513]
      tunnel: "T2 kappa_x (pN/nm)" -> [_ _ w4506]
      tunnel: w3909 -> [w4476 w4491 w4511]
      tunnel: w3906 -> [w4475 w4489 w4509]
      tunnel: [w4476 w4488 w4508] -> w3939
      tunnel: [w4475 w4487 w4507] -> w3938
      tunnel: ["T1 X (V)" ("Label.Text") "T1 X (nm)" ("Label.Text") "T1 X (pN)" ("Label.Text")] -> w3927
      tunnel: ["T2 X (V)" ("Label.Text") "T2 X (nm)" ("Label.Text") "T2 X (pN)" ("Label.Text")] -> w3926
      tunnel: ["Position (V)" ("Label.Text") "Position (nm)" ("Label.Text") "Force (pN)" ("Label.Text")] -> w3928
      tunnel: w3908 -> [_ w4479 w4498]
      tunnel: w3910 -> [_ w4482 w4500]
      tunnel: ["Mean (V)" ("Label.Text") "Mean (nm)" ("Label.Text") "Mean (pN)" ("Label.Text")] -> w3923
      tunnel: ["Difference (V)" ("Label.Text") "Difference (nm)" ("Label.Text") "Difference (pN)" ("Label.Text")] -> w3826
      frame #0 {
      }
      frame #1 {
        n1228 = Unbundle By Name(w4491) -> ("Y"=w4495:dbl[])
        n1229 = Unbundle By Name(w4489) -> ("Y"=w4480:dbl[])
        n1230 = Subtract(x=w4495, y=w4482) -> (x-y=w4483:dbl[])
        n1231 = Subtract(x=w4480, y=w4479) -> (x-y=w4481:dbl[])
        n1232 = Multiply(x=w4481, y=w4493) -> (x*y=w4490:dbl[])
        n1233 = Multiply(x=w4494, y=w4483) -> (x*y=w4492:dbl[])
        n1234 = Bundle By Name(cluster=w4489, "Y"=w4490) -> (w4487:waveform(dbl))
        n1235 = Bundle By Name(cluster=w4491, "Y"=w4492) -> (w4488:waveform(dbl))
      }
      frame #2 {
        n1236 = Unbundle By Name(w4511) -> ("Y"=w4516:dbl[])
        n1237 = Unbundle By Name(w4509) -> ("Y"=w4514:dbl[])
        n1238 = Subtract(x=w4514, y=w4498) -> (x-y=w4499:dbl[])
        n1239 = Subtract(x=w4516, y=w4500) -> (x-y=w4501:dbl[])
        n1240 = Compound Arithmetic op=MULTIPLY(w4499, w4513, w4506) -> (w4510:dbl[])
        n1241 = Compound Arithmetic op=MULTIPLY(w4505, w4515, w4501) -> (w4512:dbl[])
        n1242 = Bundle By Name(cluster=w4509, "Y"=w4510) -> (w4507:waveform(dbl))
        n1243 = Bundle By Name(cluster=w4511, "Y"=w4512) -> (w4508:waveform(dbl))
      }
    }
    n1244 = feedback #19(u16 1 ("Calibration")) -> (w3930:u16)
    n1245 = case shown="True" "Read Lateness and Rel Phase" {
      tunnel: w3867 -> [w4162 w4180]
      tunnel: w3866 -> [w4163 w4179]
      tunnel: [w4162 w4178] -> w3900
      tunnel: [w4163 w4177] -> w3899
      frame #0 {
      }
      frame #1 {
        n1246 = xnode "Read/Write Control"("FPGA VI Reference In"=w4180, "error in"=w4179) -> ("FPGA VI Reference Out"=w4178:T13, "error out"=w4177:errorcluster, "GI Relative phase"=→"GI relative phase":i16, "Relative phase"=→"Relative phase (AI1)":i16, "AI Late Counter"=→"Late Counter (AI1)":u32, "GI Late Counter"=→"GI Late Counter":u32, "MCL Late Counter"=→"MCL Late Counter":u32, "MCL Relative Phase"=→"Relative Phase (MCL)":i16, "APD Acq Relative Phase"=→"APD Acq Relative Phase":i16, "APD Gate Relative Phase"=→"APD Gate Relative Phase":i16, "APD Acq Late Counter"=→"APD Acq Late Counter":u32, "APD Gate Late Counter"=→"APD Gate Late Counter":u32, "Green FB Relative Phase"=→"Relative phase (Green FB)":i16, "GI Relative phase 2"=→"GI relative phase 2":i16, "GI Late Counter 2"=→"GI Late Counter 2":u32)
      }
    }
    n1247 = Not Equal?(x=w3930, y="Calibration") -> (x != y?=w3873:bool)
    n1248 = Unbundle By Name(w3909) -> ("Y"=w3912:dbl[])
    n1249 = Unbundle By Name(w3906) -> ("Y"=w3915:dbl[])
    n1250 = Subtract(x=w3912, y=w3910) -> (x-y=w3913:dbl[])
    n1251 = Subtract(x=w3915, y=w3908) -> (x-y=w3914:dbl[])
    n1252 = Multiply(x=w3914, y="T2 alpha_x (nm/V)") -> (x*y=w3905:dbl[])
    n1253 = Multiply(x="T1 alpha_x (nm/V)", y=w3913) -> (x*y=w3904:dbl[])
    n1254 = Multiply(x=w3938, y=-1.0) -> (x*y=w3917:waveform(dbl))
    n1255 = Subtract(x=w3905, y=w3904) -> (x-y=w3902:dbl[])
    n1256 = Unbundle By Name(w3938) -> ("Y"=w3854:dbl[])
    n1257 = Unbundle By Name(w3939) -> ("Y"=w3855:dbl[])
    n1258 = Build Array(w3939, w3917) -> (→"Force":waveform(dbl)[])
    n1259 = Subtract(x=w3902, y="Offset (nm)") -> (x-y=w3852:dbl[])
    n1260 = call <vilib>:"Mean.vi"("X"=w3854) -> ("mean"=w3830:dbl)  [unwired: 1 out]
    "T2 X" <- w3830
    n1261 = Absolute Value(x=w3855) -> (abs(x)=w3856:dbl[])
    n1262 = Absolute Value(x=w3854) -> (abs(x)=w3857:dbl[])
    n1263 = call <vilib>:"Mean.vi"("X"=w3855) -> ("mean"=w3831:dbl)  [unwired: 1 out]
    "T1 X" <- w3831
    n1264 = Add(x=w3856, y=w3857) -> (x+y=w3858:dbl[])
    n1265 = Bundle By Name(cluster=w3909, "Y"=w3852) -> (→"Bead Separation":waveform(dbl))
    n1266 = Divide(x=w3858, y=2.0) -> (x/y=→"Vec Mean of T1 T2":dbl[])
    n1267 = case shown="True" w3873 {
      tunnel: w3928 -> [_ w4469]
      tunnel: w3927 -> [_ w4468]
      tunnel: w3926 -> [_ w4467]
      tunnel: w3923 -> [_ w4466]
      tunnel: w3826 -> [_ w4465]
      frame #0 {
      }
      frame #1 {
        n1268 = property on="Force" class="WFChart (strict)"("YScale.NameLbl.Text"=w4469) -> ()  [unwired: 2 in, 2 out]
        n1269 = property on="T2 X" class="DigNum (strict)"("Caption.Text"=w4467) -> ()  [unwired: 2 in, 2 out]
        n1270 = property on="T1 X" class="DigNum (strict)"("Caption.Text"=w4468) -> ()  [unwired: 2 in, 2 out]
        n1271 = property on="Mean" class="DigNum (strict)"("Caption.Text"=w4466) -> ()  [unwired: 2 in, 2 out]
        n1272 = property on="Difference" class="DigNum (strict)"("Caption.Text"=w4465) -> ()  [unwired: 2 in, 2 out]
      }
    }
    n1273 = local read "Tether"() -> (w3861:bool)
    n1274 = Absolute Value(x=w3831) -> (abs(x)=w3828:dbl)
    n1275 = Absolute Value(x=w3830) -> (abs(x)=w3827:dbl)
    n1276 = local read "Display Period (s)"() -> (w3845:dbl)
    n1277 = Add(x=w3828, y=w3827) -> (x+y=w3925:dbl)
    n1278 = Subtract(x=w3828, y=w3827) -> (x-y=→"Difference":dbl)
    n1279 = feedback #20(w3852) -> (w3851:dbl[])
    n1280 = Divide(x=w3925, y=2.0) -> (x/y=w3860:dbl)
    "Mean" <- w3860
    n1281 = case shown="True" w3861 {
      tunnel: w3860 -> [_ w4118]
      frame #0 {
      }
      frame #1 {
        n1282 = Greater?(x="Lost Tether Alarm Threshold (pN)", y=w4118) -> (0:w4116:bool)
        n1283 = case shown="True" w4116 {
          frame #0 {
          }
          frame #1 {
            n1284 = local read "Time tether formed"() -> (w4124:timestamp)
            n1285 = Get Date/Time In Seconds() -> (seconds since 1Jan1904=w4125:timestamp)
            n1286 = Subtract(x=w4125, y=w4124) -> (x-y=w4123:dbl)
            n1287 = Number To Decimal String(number=w4123) -> (decimal integer string=w4120:string)  [unwired: 1 out]
            n1288 = local read "Messages"() -> (w4127:string)
            n1289 = call <vilib>:"Beep.vi"() -> ()  [unwired: 3 in, 9 out]
            n1290 = Concatenate Strings("Lost tether (" ("Message to add"), w4120, " s)." ("string")) -> (w4122:string)
            n1291 = local write "Tether"(FALSE ("Tether")) -> ()
            n1292 = call "Update messages.vi"("Message to add"=w4122, "Old message string"=w4127) -> ("New message string"=w4126:string)
            n1293 = local write "Messages"(w4126) -> ()
          }
        }
      }
    }
    n1294 = Build Array (concatenate)(w3852, w3851) -> (w3850:dbl[])
    n1295 = Divide(x="Bead Sep. Int. Time (s)", y=w3845) -> (x/y=w3844:dbl)
    n1296 = Split 1D Array(array=w3850, index=w3844) -> (first subarray=w3843:dbl[])  [unwired: 1 out]
    n1297 = xnode "Read/Write Control"("FPGA VI Reference In"=w3900, "error in"=w3899) -> ("FPGA VI Reference Out"=w4029:T13, "error out"=w4023:errorcluster, "AI2 Y Sum Set 1"=w4019:i16, "AI2 Y Sum Set 2"=w4018:i16, "Scanning"=→"AOD Scanning":bool, "Scan I"=→"AOD Scan I":u64, "Scanning MCL"=w4021:bool, "Scan I (MCL)"=→"MCL Scan I":u64, "Green FB Signals"=w3948:T31)  [unwired: 1 out]
    "MCL Scanning" <- w4021
    n1298 = call <vilib>:"Mean.vi"("X"=w3843) -> ("mean"=w3842:dbl)  [unwired: 1 out]
    "Bead Mean (nm)" <- w3842
    n1299 = Subtract(x=w3843, y=w3842) -> (x-y=w3841:dbl[])
    n1300 = Square(x=w3841) -> (x^2=w3840:dbl[])
    n1301 = call <vilib>:"Mean.vi"("X"=w3840) -> ("mean"=w3839:dbl)  [unwired: 1 out]
    n1302 = Square Root(x=w3839) -> (sqrt(x)=w3838:dbl)
    n1303 = Multiply(x=10.0, y=w3838) -> (x*y=→"RMS (Ang)":dbl)
    n1304 = flat-sequence "To save data" {
      tunnel: [w6364] -> w4042
      tunnel: [w6365] -> w4041
      tunnel: w3982 -> [w6358]
      tunnel: w3848 -> [w6362]
      tunnel: ["Save Calibration"] -> w4010
      tunnel: w4005 -> [w6361]
      tunnel: [w6354] -> w4004
      tunnel: [w6351] -> w4002
      tunnel: [w6348] -> w4001
      tunnel: w3981 -> [w6350]
      tunnel: w3869 -> [w6343]
      tunnel: [w6343] -> w3868
      tunnel: w4042 -> [w6551]
      tunnel: w4041 -> [w6550]
      tunnel: w4040 -> [w6549]
      tunnel: w4010 -> [w6548]
      tunnel: w4004 -> [w6546]
      tunnel: w4002 -> [w6545]
      tunnel: w4001 -> [w6544]
      tunnel: w3832 -> [w6543]
      tunnel: w3891 -> [w6542]
      tunnel: w3868 -> [w6541]
      frame #0 {
        n1305 = Or(x="Save N Sets", y="Start Saving") -> (x .or. y?=w6345:bool)
        n1306 = To Double Precision Float(number=w6361) -> (double precision float=w6355:dbl)
        n1307 = Build Array(w6345, "Save Calibration", w6358, w6350) -> (w6360:bool[])
        n1308 = Compound Arithmetic op=OR("Save Calibration", w6358, w6345, w6350) -> (w6363:bool)
        n1309 = Boolean Array To Number(Boolean array=w6360) -> (number=w6357:u32)
        n1310 = feedback #21(refnum<k0> refnum) -> (w6366:refnum<file>)
        n1311 = feedback #22(FALSE ("Save APD Data\nwith Trap Data")) -> (w6349:bool)
        n1312 = feedback #23(refnum<k0> refnum) -> (w6352:refnum<file>)
        n1313 = feedback #24(0) -> (w6368:i32)
        n1314 = feedback #25() -> (w6356:u32)  [unwired: 1 out]
        n1315 = case shown="True" w6363 {
          tunnel: [w6373 1] -> w6364
          tunnel: w6368 -> [w6375 _]
          tunnel: [w6374 w6388] -> w6365
          tunnel: w6366 -> [w6374 _]
          tunnel: w6362 -> [_ w6408]
          tunnel: w6355 -> [_ w6406]
          tunnel: w6357 -> [_ w6409]
          tunnel: [w6372 w6387] -> w6354
          tunnel: w6356 -> [w6372 _]
          tunnel: [w6371 w6384] -> w6351
          tunnel: w6352 -> [w6371 _]
          tunnel: [w6370 w6383] -> w6348
          tunnel: w6349 -> [w6370 _]
          tunnel: "Start Saving" -> [_ w6381]
          tunnel: w6343 -> [_ w6380]
          frame #0 {
            n1316 = Increment(x=w6375) -> (x+1=w6373:i32)
          }
          frame #1 {
            w6376 = FALSE ("Start Saving")
            w6382 = 9.0  # File Version
            w6391 = FALSE ("prepend array or string size? (T)")
            w6389 = T19."big-endian, network order" ("byte order (0:big-endian, network order)")
            n1317 = Array Size(array=w6380) -> (size(s)=w6379:i32)
            n1318 = local read "BD 1 Frequency 1 (MHz)"() -> (w6405:dbl)
            n1319 = local read "BD 2 Frequency 1 (MHz)"() -> (w6404:dbl)
            n1320 = local read "BD 1 Frequency 2 (MHz)"() -> (w6403:dbl)
            n1321 = local read "BD 2 Frequency 2 (MHz)"() -> (w6402:dbl)
            n1322 = local read "BD 1 Frequency 3 (MHz)"() -> (w6401:dbl)
            n1323 = local read "BD 2 Frequency 3 (MHz)"() -> (w6400:dbl)
            n1324 = To Double Precision Float(number=w6379) -> (double precision float=w6378:dbl)
            n1325 = local write "Start Saving"(w6376) -> ()
            n1326 = local write "Save Calibration"(w6376) -> ()
            n1327 = Build Array(w6405, w6404, w6403, w6402, w6401, w6400) -> (w6399:dbl[])
            n1328 = case shown="2" w6409 {
              tunnel: w6408 -> [w6453 w6467 w6482 w6519]
              tunnel: w6378 -> [w6458 w6474 w6502 w6538]
              tunnel: w6406 -> [w6457 w6473 w6501 w6537]
              tunnel: [w6454 w6469 w6493 w6529] -> w6397
              tunnel: [w6443 "Cal sets to save" w6483 w6520] -> w6387
              tunnel: w6399 -> [w6455 w6470 w6495 w6531]
              tunnel: "Save APD Data\nwith Trap Data" -> [w6452 _ w6478 w6516]
              tunnel: [w6452 w6463 w6478 w6516] -> w6383
              tunnel: w6382 -> [w6446 w6461 w6476 w6514]
              tunnel: w6381 -> [w6445 _ _ _]
              frame #0 {
                w6449 = 0.0 ("f")
                # "timeseries"
                n1329 = local read "Save ave N"() -> (w6460:dbl)
                n1330 = Multiply(x=w6460, y=w6453) -> (x*y=w6459:dbl)
                n1331 = Boolean To (0,1)(Boolean=w6452) -> (0, 1=w6451:i16)
                n1332 = To Double Precision Float(number=w6451) -> (double precision float=w6450:dbl)
                n1333 = Build Array(w6446, w6453, w6459, w6458, w6457, 0.0 ("f")) -> (w6456:dbl[])
                n1334 = Build Array(w6450, w6449, w6449, w6449, w6449) -> (w6447:dbl[])
                n1335 = Select(t=u32 4000000000, s=w6445, f="N sets to save") -> (s? t:f=w6443:u32)
                n1336 = Build Array (concatenate)(w6456, w6455, w6447) -> (w6454:dbl[])
              }
              frame #1 {
                w6464 = 0.0 ("f")
                w6463 = FALSE ("Save APD Data\nwith Trap Data")
                # "calibration"
                n1337 = Boolean To (0,1)(Boolean=w6463) -> (0, 1=w6466:i16)
                n1338 = To Double Precision Float(number=w6466) -> (double precision float=w6465:dbl)
                n1339 = Build Array(w6465, w6464, w6464, w6464, w6464) -> (w6462:dbl[])
                n1340 = Build Array(w6461, w6467, w6467, w6474, w6473, 1.0 ("t")) -> (w6471:dbl[])
                n1341 = Build Array (concatenate)(w6471, w6470, w6462) -> (w6469:dbl[])
                "Calibrating Trap..." <- TRUE ("Calibrating...")
              }
              frame #2 {
                w6479 = 0.0 ("f")
                # "scan dir (x/y = 0/1)"
                # "cycles/step"
                # "n scans (f/b)"
                # "steps"
                # "freq. range"
                # "AOD raster scan"
                n1342 = local read "Number of F/B Scans (AOD)"() -> (w6487:u16)
                n1343 = local read "Cycles/step (AOD)"() -> (w6489:u64)
                n1344 = local read "Scan Range (MHz)"() -> (w6492:dbl)
                n1345 = local read "Scan steps (AOD)"() -> (w6491:u64)
                n1346 = local read "Scan BD"() -> (w6499:bool)
                n1347 = local read "Save ave N"() -> (w6504:dbl)
                n1348 = Boolean To (0,1)(Boolean=w6499) -> (0, 1=w6498:i16)
                n1349 = To Double Precision Float(number=w6487) -> (double precision float=w6486:dbl)
                n1350 = To Double Precision Float(number=w6491) -> (double precision float=w6490:dbl)
                n1351 = To Double Precision Float(number=w6489) -> (double precision float=w6488:dbl)
                n1352 = To Double Precision Float(number=w6498) -> (double precision float=w6497:dbl)
                n1353 = Boolean To (0,1)(Boolean=w6478) -> (0, 1=w6481:i16)
                n1354 = Multiply(x=w6504, y=w6482) -> (x*y=w6503:dbl)
                n1355 = To Double Precision Float(number=w6481) -> (double precision float=w6480:dbl)
                n1356 = Build Array(w6480, w6479, w6479, w6479, w6479) -> (w6477:dbl[])
                n1357 = local read "N sets should be saved"() -> (w6484:dbl)
                n1358 = Build Array(w6497, w6492, w6490, w6488, w6486) -> (w6494:dbl[])
                n1359 = Build Array(w6476, w6482, w6503, w6502, w6501, 2.0 ("t")) -> (w6496:dbl[])
                n1360 = Round Toward +Infinity(x=w6484) -> (ceil(x): smallest int >= x=w6485:dbl)
                n1361 = Build Array (concatenate)(w6496, w6495, w6477, w6494) -> (w6493:dbl[])
                n1362 = To Unsigned Long Integer(number=w6485) -> (unsigned 32bit integer=w6483:u32)
              }
              frame #3 {
                w6511 = 0.0 ("f")
                # "MCL raster scan"
                n1363 = local read "Number of scans (MCL)"() -> (w6506:u64)
                n1364 = local read "2D or 1D Scan"() -> (w6508:bool)
                n1365 = local read "Scan lines"() -> (w6505:u64)
                n1366 = local read "Fast Scan Dir"() -> (w6535:bool)
                n1367 = local read "Cycles/step (MCL)"() -> (w6525:u64)
                n1368 = Select(t=w6505, s=w6508, f=w6506) -> (s? t:f=w6507:u64)
                n1369 = local read "Scan steps (MCL)"() -> (w6527:u64)
                n1370 = local read "Scan Range (V)"() -> (w6528:dbl)
                n1371 = Boolean To (0,1)(Boolean=w6508) -> (0, 1=w6510:i16)
                n1372 = local read "Save ave N"() -> (w6540:dbl)
                n1373 = local read "Initial X"() -> (w6513:dbl)
                n1374 = local read "Initial Y"() -> (w6512:dbl)
                n1375 = To Double Precision Float(number=w6510) -> (double precision float=w6509:dbl)
                n1376 = Boolean To (0,1)(Boolean=w6535) -> (0, 1=w6534:i16)
                n1377 = To Double Precision Float(number=w6507) -> (double precision float=w6523:dbl)
                n1378 = To Double Precision Float(number=w6527) -> (double precision float=w6526:dbl)
                n1379 = To Double Precision Float(number=w6525) -> (double precision float=w6524:dbl)
                n1380 = To Double Precision Float(number=w6534) -> (double precision float=w6533:dbl)
                n1381 = Boolean To (0,1)(Boolean=w6516) -> (0, 1=w6518:i16)
                n1382 = Multiply(x=w6540, y=w6519) -> (x*y=w6539:dbl)
                n1383 = To Double Precision Float(number=w6518) -> (double precision float=w6517:dbl)
                n1384 = local read "N sets should be saved (MCL)"() -> (w6521:dbl)
                n1385 = Build Array(w6517, w6509, w6511, w6511, w6511) -> (w6515:dbl[])
                n1386 = Build Array(w6533, w6528, w6526, w6524, w6523, w6513, w6512) -> (w6530:dbl[])
                n1387 = Build Array(w6514, w6519, w6539, w6538, w6537, 3.0 ("t")) -> (w6532:dbl[])
                n1388 = Round Toward +Infinity(x=w6521) -> (ceil(x): smallest int >= x=w6522:dbl)
                n1389 = Build Array (concatenate)(w6532, w6531, w6515, w6530) -> (w6529:dbl[])
                n1390 = To Unsigned Long Integer(number=w6522) -> (unsigned 32bit integer=w6520:u32)
              }
            }
            n1391 = local read "Index"() -> (w6414:dbl)
            n1392 = call "Create new save file.vi"("Insert"="", "Ext"=".dat", "Index In"=w6414) -> ("Path Out"=w6385:path, "Index Out"=w6386:dbl)
            n1393 = local write "Index"(w6386) -> ()
            n1394 = local write "Save file name"(w6385) -> ()
            n1395 = local write "Save index"(w6386) -> ()
            n1396 = Array Size(array=w6397) -> (size(s)=w6398:i32)
            n1397 = Open/Create/Replace File(file path (use dialog)=w6385, operation (0:open)=T20."create", access (0:read/write)=enum16{"read/write", "read-only", "write-only"}."write-only") -> (refnum out=w6411:refnum<file>)  [unwired: 1 in, 4 out]
            n1398 = local write "Saving..."(TRUE ("Saving...")) -> ()
            n1399 = To Double Precision Float(number=w6398) -> (double precision float=w6396:dbl)
            n1400 = String Length(string="Comment (data description)") -> (length=w6394:i32)
            n1401 = To Double Precision Float(number=w6394) -> (double precision float=w6393:dbl)
            n1402 = Deny Access(7:w6411) -> (3:w6410:refnum<file>)  [unwired: 1 in, 2 out]
            n1403 = Build Array (concatenate)(w6396, w6397, w6393) -> (w6395:dbl[])
            n1404 = case "If fluorescence data to be saved" shown="True" w6383 {
              tunnel: w6385 -> [_ w6441]
              tunnel: [refnum<k0> refnum w6421] -> w6384
              frame #0 {
              }
              frame #1 {
                w6420 = 0.0
                n1405 = local read "APD Integration Time (s)"() -> (w6426:dbl)
                n1406 = local read "N APD Samp/step"() -> (w6419:dbl)
                n1407 = Path To String(path=w6441) -> (string=w6440:string)
                n1408 = String Length(string=w6440) -> (length=w6439:i32)
                n1409 = Subtract(x=w6439, y=4) -> (x-y=w6437:i32)
                n1410 = String Subset(string=w6440, length (rest)=w6437) -> (substring=w6436:string)  [unwired: 1 out]
                n1411 = Build Array(w6426, w6419, w6420, w6420, w6420, w6420, w6420, w6420) -> (w6423:dbl[])
                n1412 = Concatenate Strings(w6436, "_fl.dat" ("string")) -> (w6434:string)
                n1413 = Array Size(array=w6423) -> (size(s)=w6425:i32)
                n1414 = String To Path(string=w6434) -> (path=w6430:path)
                n1415 = Open/Create/Replace File(file path (use dialog)=w6430, operation (0:open)=T20."create", access (0:read/write)=enum16{"read/write", "read-only", "write-only"}."write-only") -> (refnum out=w6431:refnum<file>)  [unwired: 1 in, 4 out]
                n1416 = Deny Access(7:w6431) -> (3:w6427:refnum<file>)  [unwired: 1 in, 2 out]
                n1417 = To Double Precision Float(number=w6425) -> (double precision float=w6424:dbl)
                n1418 = Build Array (concatenate)(w6424, w6423) -> (w6422:dbl[])
                n1419 = Write to Binary File(file (use dialog)=w6427, data=w6422, 5:FALSE ("prepend array or string size? (T)"), 9:T19."big-endian, network order" ("byte order (0:big-endian, network order)")) -> (refnum out=w6421:refnum<file>)  [unwired: 1 in, 3 out]
              }
            }
            n1420 = Write to Binary File(file (use dialog)=w6410, data=w6395, 5:w6391, 9:w6389) -> (refnum out=w6392:refnum<file>)  [unwired: 1 in, 3 out]
            n1421 = Write to Binary File(file (use dialog)=w6392, data="Comment (data description)", 5:w6391, 9:w6389) -> (refnum out=w6388:refnum<file>)  [unwired: 1 in, 3 out]
          }
        }
      }
      frame #1 {
        n1422 = local read "Saving..."() -> (w6547:bool)
        n1423 = case shown="True" w6547 {
          tunnel: w6551 -> [_ w6555]
          tunnel: w6550 -> [_ w6569]
          tunnel: w6549 -> [_ w6565]
          tunnel: w6548 -> [_ w6564]
          tunnel: w6546 -> [_ w6563]
          tunnel: w6545 -> [_ w6558]
          tunnel: w6544 -> [_ w6557]
          tunnel: w6543 -> [_ w6556]
          tunnel: w6542 -> [_ w6554]
          tunnel: w6541 -> [_ w6552]
          frame #0 {
          }
          frame #1 {
            n1424 = Multiply(x=w6555, y=w6554) -> (x*y=→"Time (s)":dbl)
            n1425 = Less Or Equal?(x=w6555, y=w6563) -> (x <= y?=w6567:bool)
            n1426 = Or(x="Stop Saving", y="Abort save 2") -> (x .or. y?=w6559:bool)
            n1427 = Not(x=w6559) -> (.not. x?=w6568:bool)
            n1428 = And(x=w6567, y=w6568) -> (x .and. y?=w6566:bool)
            n1429 = case shown="True" w6566 {
              tunnel: w6569 -> [w6574 w6590]
              tunnel: [0.0 w6593] -> w6562
              tunnel: w6555 -> [_ w6591]
              tunnel: w6563 -> [_ w6592]
              tunnel: w6565 -> [_ w6587]
              tunnel: w6564 -> [_ _]
              tunnel: w6558 -> [w6571 w6578]
              tunnel: w6557 -> [w6570 w6579]
              tunnel: w6556 -> [_ w6577]
              tunnel: w6552 -> [_ w6576]
              frame #0 {
                w6572 = FALSE
                n1430 = Close File(refnum=w6574) -> ()  [unwired: 1 in, 2 out]
                n1431 = case shown="True" w6570 {
                  tunnel: w6571 -> [_ w6575]
                  frame #0 {
                  }
                  frame #1 {
                    n1432 = Close File(refnum=w6575) -> ()  [unwired: 1 in, 2 out]
                  }
                }
                n1433 = local write "Raster Scanning..."(w6572) -> ()
                n1434 = local write "Calibrating Trap..."(w6572) -> ()
                n1435 = call <vilib>:"Beep.vi"() -> ()  [unwired: 3 in, 9 out]
                "Saving..." <- w6572
              }
              frame #1 {
                n1436 = local read "Calibrating Trap..."() -> (w6580:bool)
                n1437 = case shown="True" w6579 {
                  tunnel: w6578 -> [_ w6597]
                  tunnel: w6577 -> [_ w6596]
                  frame #0 {
                  }
                  frame #1 {
                    n1438 = Write to Binary File(file (use dialog)=w6597, data=w6596, 5:FALSE ("prepend array or string size? (T)"), 9:T19."big-endian, network order" ("byte order (0:big-endian, network order)")) -> ()  [unwired: 1 in, 4 out]
                  }
                }
                n1439 = Greater?(x="Save ave N", y=1.0) -> (0:w6583:bool)
                n1440 = Not(x=w6580) -> (.not. x?=w6582:bool)
                n1441 = And(x=w6582, y=w6583) -> (x .and. y?=w6584:bool)
                n1442 = case shown="True" w6584 {
                  tunnel: w6587 -> [w6600 w6612]
                  tunnel: [w6600 w6603] -> w6581
                  tunnel: "Save ave N" -> [_ w6604]
                  tunnel: w6576 -> [_ w6602]
                  frame #0 {
                  }
                  frame #1 {
                    n1443 = Array Size(array=w6612) -> (size(s)=w6605:i32)
                    n1444 = Array Size(array=w6602) -> (size(s)=w6601:i32)
                    n1445 = Divide(x=w6605, y=w6601) -> (x/y=w6610:dbl)
                    n1446 = Reshape Array(w6612, w6610, w6601) -> (w6611:i16[][])
                    n1447 = Transpose 2D Array(2D array=w6611) -> (transposed array=w6609:i16[][])
                    n1448 = for {
                      tunnel: w6609 -> [w6615] mode=indexing
                      tunnel: [w6614] -> w6608 mode=indexing
                      tunnel: w6604 -> [w6613]
                      n1449 = call "downsample 1D array - I16.vi"("Ave N"=w6613, "Array In"=w6615) -> ("Array Out"=w6614:i16[])  [unwired: 1 out]
                    }
                    n1450 = Transpose 2D Array(2D array=w6608) -> (transposed array=w6607:i16[][])
                    n1451 = Divide(x=w6605, y=w6604) -> (x/y=w6606:dbl)
                    n1452 = Reshape Array(w6607, w6606) -> (w6603:i16[])
                  }
                }
                n1453 = Write to Binary File(file (use dialog)=w6590, data=w6581, 5:FALSE ("prepend array or string size? (T)"), 9:T19."big-endian, network order" ("byte order (0:big-endian, network order)")) -> ()  [unwired: 1 in, 4 out]
                n1454 = Divide(x=w6591, y=w6592) -> (x/y=w6594:dbl)
                n1455 = Multiply(x=w6594, y=100.0) -> (x*y=w6593:dbl)
              }
            }
            "Progress" <- w6562
            "Progress 2" <- w6562
          }
        }
      }
    }
    n1456 = local read "AI2 (V)"() -> (w4020:cluster{"Set 1":dbl, "Set 2":dbl})
    n1457 = Bundle By Name(cluster=w4020, "Set 1"=w4019, "Set 2"=w4018) -> (w4016:cluster{"Set 1":dbl, "Set 2":dbl})
    n1458 = Divide(x=w4016, y=3276.7) -> (x/y=w4015:cluster{"Set 1":dbl, "Set 2":dbl})
    n1459 = local write "AI2 (V)"(w4015) -> ()
    n1460 = Divide(x=w3948, y=3276.7) -> (x/y=w3944:T37)
    n1461 = Unbundle By Name(w3944) -> ("Green FB Ch 0"=w3947:dbl, "Green FB Ch 1"=w3946:dbl, "Green FB Ch 2"=w3945:dbl)
    n1462 = Divide(x=w3947, y=w3945) -> (x/y=w3943:dbl)
    n1463 = Divide(x=w3946, y=w3945) -> (x/y=w3942:dbl)
    n1464 = Bundle By Name(cluster=w3944, "Green FB Ch 0"=w3943, "Green FB Ch 1"=w3942) -> (w3922:T37)
    "Green FB Signals (V)" <- w3922
    n1465 = Unbundle By Name(w3922) -> ("Green FB Ch 2"=→"Green FB Plot":dbl)
    n1466 = local read "wait to reset values"() -> (w4024:bool)
    n1467 = Not(x=w4021) -> (.not. x?=w4025:bool)
    n1468 = And(x=w4025, y=w4024) -> (x .and. y?=w4026:bool)
    n1469 = case "Part of MCL raster scanning: returns to initial positions after scan done" shown="True" w4026 {
      tunnel: w4029 -> [w5310 w5317]
      tunnel: [w5310 w5316] -> w4028
      tunnel: w4023 -> [w5309 w5315]
      tunnel: [w5309 w5314] -> w4022
      frame #0 {
      }
      frame #1 {
        w5325 = 10.0 ("y")
        w5324 = 32767.0 ("y")
        # "to return scan values\nafter a synchronous \nAOM scan"
        n1470 = local read "AO2"() -> (w5318:dbl)
        n1471 = local read "AO1"() -> (w5319:dbl)
        n1472 = Multiply(x=w5319, y=w5324) -> (x*y=w5321:dbl)
        n1473 = Multiply(x=w5318, y=w5324) -> (x*y=w5323:dbl)
        n1474 = local write "wait to reset values"(FALSE ("wait to reset values")) -> ()
        n1475 = Divide(x=w5321, y=w5325) -> (x/y=w5320:dbl)
        n1476 = Divide(x=w5323, y=w5325) -> (x/y=w5322:dbl)
        n1477 = To Word Integer(number=w5320) -> (16bit integer=w5326:i16)
        n1478 = To Word Integer(number=w5322) -> (16bit integer=w5327:i16)
        n1479 = local read "Total Counts (ticks)"() -> (w5311:u32)
        n1480 = xnode "Read/Write Control"("FPGA VI Reference In"=w5317, "error in"=w5315, "AO1"=w5326, "AO2"=w5327, "MCL count"=w5311) -> ("FPGA VI Reference Out"=w5316:T13, "error out"=w5314:errorcluster)
        n1481 = local read "Scan Range (V)"() -> (w5312:dbl)
        n1482 = property on="Scan Range (V)" class="DigNum (strict)"("Val(Sgnl)"=w5312) -> ()  [unwired: 2 in, 2 out]
      }
    }
    n1483 = node-c288() -> ()  [unwired: 2 out]
  }
  n1484 = timed-loop "Oscillate AOD (debugging)" {
    tunnel: w73 -> [w6689]
    tunnel: [w6688] -> w13
    timing: w6 -> [_]
    timing-out: [_] -> w5
    stop <- w6688 stop-if-true
    n1485 = node-c288() -> ()  [unwired: 2 out]
    n1486 = event shown="[0] \"Oscillate Set 1\", \"Fish for Tether\": Value Change" {
      selector: _ -> [_ _ _]
      dyn-events: _ -> [_ _ _]
      timeout: _ -> [_ _ _]
      tunnel: w6689 -> [w6696 _ _]
      tunnel: [FALSE ("Stop All") _ w6879] -> w6688
      event #0 {
        n1487 = event-data() -> ()  [unwired: 6 out]
        n1488 = local read "Oscillate Set 1"() -> (w6695:bool)
        n1489 = Or(x=w6695, y="Fish for Tether") -> (x .or. y?=w6693:bool)
        n1490 = case shown="True" w6693 {
          tunnel: w6696 -> [_ w6698]
          tunnel: "Fish for Tether" -> [_ w6697]
          frame #0 {
          }
          frame #1 {
            n1491 = case shown="True" w6697 {
              frame #0 {
              }
              frame #1 {
                n1492 = local write "Scan axis 2"(TRUE) -> ()
                n1493 = local write "Tether"(FALSE ("Tether")) -> ()
              }
            }
            n1494 = node-c288() -> (w6700:T16)  [unwired: 4 out]
            n1495 = timed-loop "Oscillate AOD" {
              timing: w6700 -> [_]
              timing-out: [_] -> w6699
              tunnel: w6698 -> [w6710]
              tunnel: w6697 -> [w6709]
              i -> [w6712]
              stop <- w6708 stop-if-true
              n1496 = node-c288() -> (w6711:i64)  [unwired: 1 out]
              n1497 = flat-sequence {
                tunnel: w6712 -> [w6739]
                tunnel: w6711 -> [w6738]
                tunnel: w6710 -> [w6717]
                tunnel: w6709 -> [w6720]
                tunnel: [w6720] -> w6707
                tunnel: [w6719] -> w6706
                tunnel: [w6716] -> w6705
                tunnel: [w6713] -> w6703
                tunnel: w6707 -> [w6775]
                tunnel: w6706 -> [w6773]
                tunnel: w6705 -> [w6772]
                tunnel: [w6771] -> w6704
                tunnel: w6703 -> [w6770]
                tunnel: [w6802] -> w6708
                tunnel: w6704 -> [w6801]
                frame #0 {
                  n1498 = Divide(x=w6738, y=i64 1000) -> (x/y=w6733:dbl)
                  n1499 = Multiply(x=w6733, y=w6739) -> (x*y=w6735:dbl)
                  n1500 = local read "BD 1 Frequency 2 (MHz)"() -> (w6718:dbl)
                  n1501 = Multiply(x="Osc. freq. (Hz)", y=6.283185307179586) -> (x*y=w6736:dbl)
                  n1502 = Multiply(x=w6736, y=w6735) -> (x*y=w6715:dbl)
                  n1503 = local read "BD 1 Frequency 1 (MHz)"() -> (w6723:dbl)
                  n1504 = case shown="True" w6720 {
                    tunnel: w6715 -> [w6745 w6750]
                    tunnel: w6723 -> [_ w6761]
                    tunnel: w6718 -> [_ w6762]
                    tunnel: [w6742 w6756] -> w6721
                    tunnel: [FALSE w6753] -> w6716
                    tunnel: [0.0 w6746] -> w6713
                    frame #0 {
                      n1505 = Sine(x=w6745) -> (sin(x)=w6743:dbl)
                      n1506 = Multiply(x=w6743, y="Osc. amp. (MHz)") -> (x*y=w6742:dbl)
                    }
                    frame #1 {
                      n1507 = Cosine(x=w6750) -> (cos(x)=w6765:dbl)
                      n1508 = Subtract(x=w6762, y=w6761) -> (x-y=w6760:dbl)
                      n1509 = Decrement(x=w6765) -> (x-1=w6764:dbl)
                      n1510 = Subtract(x=w6760, y="Closest Delta (MHz)") -> (x-y=w6757:dbl)
                      n1511 = Divide(x=w6764, y=-2.0) -> (x/y=w6758:dbl)
                      n1512 = Multiply(x=w6758, y=w6757) -> (x*y=w6756:dbl)
                      n1513 = local read "Vec Mean of T1 T2"() -> (w6752:dbl[])
                      n1514 = Greater?(x=w6752, y="Stop F (pN)") -> (0:w6754:bool[])
                      n1515 = Or Array Elements(Boolean array=w6754) -> (logical OR=w6753:bool)
                      n1516 = Divide(x=w6750, y=6.283185307179586) -> (x/y=w6749:dbl)
                      n1517 = Round Toward +Infinity(x=w6749) -> (ceil(x): smallest int >= x=w6746:dbl)
                      "Attempts" <- w6746
                      n1518 = Greater?(x=w6746, y="Attempt Limit") -> (0:w6748:bool)
                      n1519 = case shown="True" w6748 {
                        frame #0 {
                        }
                        frame #1 {
                          n1520 = call <vilib>:"Beep.vi"() -> ()  [unwired: 3 in, 9 out]
                          n1521 = local write "Fish for Tether"(FALSE ("Fish for Tether")) -> ()
                          n1522 = local read "Messages"() -> (w6767:string)
                          n1523 = call "Update messages.vi"("Message to add"="Tether fishing timeout." ("Messages"), "Old message string"=w6767) -> ("New message string"=→"Messages":string)
                        }
                      }
                    }
                  }
                  n1524 = local read "BD 2 Frequency 1 (MHz)"() -> (w6722:dbl)
                  n1525 = Select(t=w6723, s="Scan axis 2", f=w6722) -> (s? t:f=w6726:dbl)
                  n1526 = Add(x=w6721, y=w6726) -> (x+y=w6719:dbl)
                  n1527 = Select(t=w6719, s="Scan axis 2", f=w6723) -> (s? t:f=w6729:dbl)
                  n1528 = Select(t=w6722, s="Scan axis 2", f=w6719) -> (s? t:f=w6728:dbl)
                  n1529 = local read "Y RF Frequency Limits (MHz)"() -> (w6724:T11)
                  n1530 = local read "X RF Frequency Limits (MHz)"() -> (w6725:T11)
                  n1531 = local read "BD 1 Frequency 3 (MHz)"() -> (w6732:dbl)
                  n1532 = local read "BD 2 Frequency 2 (MHz)"() -> (w6731:dbl)
                  n1533 = local read "BD 2 Frequency 3 (MHz)"() -> (w6730:dbl)
                  n1534 = call "set RF board frequency - interlace.vi"("Board 2 Frequency Limits"=w6724, "Board 1 Frequency Limits"=w6725, "FPGA VI Reference In"=w6717, "Board 2 Frequency 3 (MHz)"=w6730, "Board 1 Frequency 3 (MHz)"=w6732, "Board 2 Frequency 2 (MHz)"=w6731, "Board 2 Frequency 1 (MHz)"=w6728, "Board 1 Frequency 2 (MHz)"=w6718, "Board 1 Frequency 1  (MHz)"=w6729) -> ()  [unwired: 1 in, 2 out]
                }
                frame #1 {
                  n1535 = And(x=w6775, y=w6772) -> (x .and. y?=w6774:bool)
                  n1536 = case "Only if were fishing and now formed tether" shown="True" w6774 {
                    tunnel: w6773 -> [w6777 w6790]
                    tunnel: [w6776 w6789] -> w6771
                    tunnel: w6770 -> [_ w6785]
                    frame #0 {
                      n1537 = local read "Fish for Tether"() -> (w6776:bool)
                      n1538 = case shown="False" w6776 {
                        tunnel: w6777 -> [w6778 _]
                        frame #0 {
                          n1539 = property on="BD 1 Frequency 1 (MHz)" class="DigNum (strict)"("Val(Sgnl)"=w6778) -> ()  [unwired: 2 in, 2 out]
                        }
                        frame #1 {
                        }
                      }
                    }
                    frame #1 {
                      w6789 = FALSE ("Fish for Tether")
                      n1540 = call <vilib>:"Beep.vi"() -> ()  [unwired: 3 in, 9 out]
                      n1541 = Number To Decimal String(number=w6785, width (-)=i16 1) -> (decimal integer string=w6783:string)
                      n1542 = case shown="\"2\", \"3\"" "Then..." {
                        selector: "Then..." -> [_ w6793]
                        tunnel: w6790 -> [w6792 _]
                        frame #0 {
                          n1543 = property on="BD 1 Frequency 1 (MHz)" class="DigNum (strict)"("Val(Sgnl)"=w6792) -> ()  [unwired: 2 in, 2 out]
                        }
                        frame #1 {
                          n1544 = flat-sequence {
                            tunnel: w6793 -> [w6795]
                            frame #0 {
                              n1545 = property on="Trap Delta (MHz)" class="DigNum (strict)"("Val(Sgnl)"="Move to Delta (MHz)") -> ()  [unwired: 2 in, 2 out]
                            }
                            frame #1 {
                              n1546 = case shown="\"3\"" w6795 {
                                frame #0 {
                                n1547 = flat-sequence {
                                frame #0 {
                                n1548 = property on="Green Laser ON/Interlacing" class="Bool (strict)"("Val(Sgnl)"=TRUE ("Value (Signaling)")) -> ()  [unwired: 2 in, 2 out]
                                }
                                frame #1 {
                                n1549 = Multiply(x="Wait Before Save (s)", y=u32 1000 ("x")) -> (x*y=w6798:u32)
                                n1550 = Wait (ms)(milliseconds to wait=w6798) -> ()  [unwired: 1 out]
                                }
                                frame #2 {
                                n1551 = property on="Start Saving" class="Bool (strict)"("Value"=TRUE ("Start Saving")) -> ()  [unwired: 2 in, 2 out]
                                }
                                }
                                }
                                frame #1 {
                                }
                              }
                            }
                          }
                        }
                      }
                      n1552 = Concatenate Strings("Formed tether in ", w6783, " attempt(s)." ("string")) -> (w6780:string)
                      n1553 = local read "Messages"() -> (w6787:string)
                      n1554 = local write "Fish for Tether"(w6789) -> ()
                      n1555 = call "Update messages.vi"("Message to add"=w6780, "Old message string"=w6787) -> ("New message string"=w6786:string)
                      n1556 = local write "Messages"(w6786) -> ()
                      n1557 = Get Date/Time In Seconds() -> (seconds since 1Jan1904=→"Time tether formed":timestamp)
                      "Tether" <- "Tether Alarm?"
                    }
                  }
                }
                frame #2 {
                  n1558 = local read "Oscillate Set 1"() -> (w6806:bool)
                  n1559 = Or(x=w6806, y=w6801) -> (x .or. y?=w6803:bool)
                  n1560 = local read "Stop All"() -> (w6804:bool)
                  n1561 = Not(x=w6803) -> (.not. x?=w6805:bool)
                  n1562 = Compound Arithmetic op=OR(w6804, w6805) -> (w6802:bool)
                }
              }
              n1563 = node-c288() -> ()  [unwired: 2 out]
            }
            n1564 = node-c288(w6699) -> ()  [unwired: 1 out]
          }
        }
      }
      event #1 {
        n1565 = event-data() -> ()  [unwired: 7 out]
        n1566 = case shown="True" "Fl. Triggered..." {
          frame #0 {
          }
          frame #1 {
            n1567 = node-c288() -> (w6815:T16)  [unwired: 4 out]
            n1568 = timed-loop {
              timing: w6815 -> [_]
              timing-out: [_] -> w6814
              tunnel: "Action" -> [w6816]
              stop <- w6817 stop-if-true
              n1569 = node-c288() -> ()  [unwired: 2 out]
              n1570 = flat-sequence {
                tunnel: w6816 -> [w6820]
                tunnel: [w6870] -> w6817
                frame #0 {
                  n1571 = local read "APD 1 Rate (Hz)"() -> (w6823:dbl)
                  n1572 = Multiply(x="Fl. Threshold (kHz)", y=1000.0) -> (x*y=w6819:dbl)
                  n1573 = Greater?(x=w6823, y=w6819) -> (0:w6821:bool)
                  n1574 = case shown="True" w6821 {
                    tunnel: w6820 -> [_ w6826]
                    frame #0 {
                    }
                    frame #1 {
                      n1575 = flat-sequence {
                        tunnel: w6828 -> [w6831]
                        tunnel: [w6831] -> w6827
                        tunnel: w6826 -> [w6830]
                        tunnel: [w6830] -> w6825
                        tunnel: [w6829] -> w6824
                        tunnel: w6827 -> [w6838]
                        tunnel: w6825 -> [w6837]
                        tunnel: w6824 -> [w6836]
                        frame #0 {
                          n1576 = call <vilib>:"Beep.vi"() -> ()  [unwired: 3 in, 9 out]
                          n1577 = case shown="\"Alarm\", Default" w6830 {
                            frame #0 {
                              n1578 = property on="Confocal Image" class="Bool (strict)"("Val(Sgnl)"=TRUE ("Value (Signaling)")) -> ()  [unwired: 2 in, 2 out]
                            }
                            frame #1 {
                            }
                            frame #2 {
                              n1579 = property on="BD 1 Frequency 1 (MHz)" class="DigNum (strict)"("Val(Sgnl)"="Yank to Freq. (MHz)") -> ()  [unwired: 2 in, 2 out]
                            }
                          }
                          n1580 = local write "Waiting"(FALSE ("Waiting")) -> ()
                          n1581 = local read "Time (s)"() -> (w6829:dbl)
                          "Fl. High" <- TRUE ("Yanking")
                        }
                        frame #1 {
                          n1582 = node-c288() -> (w6840:T16)  [unwired: 4 out]
                          n1583 = timed-loop {
                            timing: w6840 -> [_]
                            timing-out: [_] -> w6839
                            tunnel: w6838 -> [w6850]
                            tunnel: w6837 -> [w6848]
                            tunnel: w6836 -> [w6847]
                            stop <- w6849 stop-if-true
                            n1584 = node-c288() -> ()  [unwired: 2 out]
                            n1585 = local read "Fl. Threshold (kHz)"() -> (w6842:dbl)
                            n1586 = local read "Fl. Triggered..."() -> (w6851:bool)
                            n1587 = local read "APD 1 Rate (Hz)"() -> (w6852:dbl)
                            n1588 = local read "Stop All"() -> (w6845:bool)
                            n1589 = Not(x=w6851) -> (.not. x?=w6846:bool)
                            n1590 = Multiply(x=w6842, y=1000.0) -> (x*y=w6843:dbl)
                            n1591 = Less?(x=w6852, y=w6843) -> (x < y?=w6844:bool)
                            n1592 = Compound Arithmetic op=OR(w6844, w6845, w6846) -> (w6849:bool)
                            n1593 = case shown="True" w6849 {
                              tunnel: w6850 -> [_ w6863]
                              tunnel: w6848 -> [_ w6862]
                              tunnel: w6847 -> [_ w6860]
                              frame #0 {
                              }
                              frame #1 {
                                n1594 = case shown="\"Yank\"" w6862 {
                                tunnel: w6863 -> [_ w6864]
                                frame #0 {
                                }
                                frame #1 {
                                n1595 = property on="BD 1 Frequency 1 (MHz)" class="DigNum (strict)"("Val(Sgnl)"=w6864) -> ()  [unwired: 2 in, 2 out]
                                }
                                }
                                n1596 = local read "Time (s)"() -> (w6861:dbl)
                                n1597 = Subtract(x=w6861, y=w6860) -> (x-y=w6857:dbl)
                                "Duration (s)" <- w6857
                                n1598 = Number To Decimal String(number=w6857, width (-)=i16 0) -> (decimal integer string=w6855:string)
                                n1599 = Concatenate Strings(w6855, " s fluorescence event." ("string")) -> (w6853:string)
                                n1600 = local read "Messages"() -> (w6859:string)
                                n1601 = call "Update messages.vi"("Message to add"=w6853, "Old message string"=w6859) -> ("New message string"=w6858:string)
                                n1602 = call <vilib>:"Beep.vi"() -> ()  [unwired: 3 in, 9 out]
                                n1603 = local write "Messages"(w6858) -> ()
                              }
                            }
                            n1604 = node-c288() -> ()  [unwired: 2 out]
                          }
                          n1605 = node-c288(w6839) -> ()  [unwired: 1 out]
                        }
                        frame #2 {
                          n1606 = local write "Fl. High"(FALSE ("Yanking")) -> ()
                        }
                      }
                      n1607 = local read "BD 1 Frequency 1 (MHz)"() -> (w6828:dbl)
                    }
                  }
                }
                frame #1 {
                  n1608 = local read "Stop All"() -> (w6873:bool)
                  n1609 = local read "Fl. Triggered..."() -> (w6871:bool)
                  n1610 = Not(x=w6871) -> (.not. x?=w6872:bool)
                  n1611 = Or(x=w6872, y=w6873) -> (x .or. y?=w6870:bool)
                  n1612 = Not(x=w6870) -> (.not. x?=→"Waiting":bool)
                }
              }
              n1613 = node-c288() -> ()  [unwired: 2 out]
            }
            n1614 = node-c288(w6814) -> ()  [unwired: 1 out]
          }
        }
      }
      event #2 {
        n1615 = event-data() -> ()  [unwired: 7 out]
        n1616 = local read "Stop All"() -> (w6879:bool)
      }
    }
    n1617 = node-c288() -> ()  [unwired: 2 out]
  }
  n1618 = timed-loop {
    shift-right: [w6891] -> w54
    shift-left: w56 -> [w6908]
    shift-right: [w6890] -> w53
    shift-left: w55 -> [w6907]
    tunnel: w52 -> [w6892]
    timing: w10 -> [_]
    timing-out: [_] -> w9
    shift-right: ["Dump Beads"] -> _
    shift-left: FALSE ("Dump Beads") -> [w6883]
    stop <- w6909 stop-if-true
    (unwired) T11 {"Minimum"=0.0, "Maximum"=0.0, "Increment"=0.0}  # Y Limits
    (unwired) T11 {"Minimum"=0.0, "Maximum"=0.0, "Increment"=0.0}  # X Limits
    n1619 = node-c288() -> ()  [unwired: 2 out]
    n1620 = local read "Stop All"() -> (w6909:bool)
    n1621 = call "Read Stage Position.vi"("error in"=w6907, "VISA resource name in"=w6908) -> ("Current Position"=w6893:cluster{dbl, dbl, dbl}, "error out"=w6900:errorcluster, "VISA resource name out"=w6901:refnum<visa-resource-name>)  [unwired: 1 out]
    "Current Stage  Position" <- w6893
    n1622 = Or(x="Move to Position 3", y="Data Acq. Spot") -> (x .or. y?=w6886:bool)
    n1623 = Or(x="Lower Cap.", y=w6883) -> (x .or. y?=w6882:bool)
    n1624 = Or(x="Move to Position 1", y="Upper Cap.") -> (x .or. y?=w6889:bool)
    n1625 = Compound Arithmetic op=OR(w6882, "Move to Position 2") -> (w6888:bool)
    n1626 = Or(x="Dump Beads", y="Move to Position 4") -> (x .or. y?=w6885:bool)
    n1627 = Build Array(w6889, w6888, w6886, w6885) -> (w6899:bool[])
    n1628 = Or Array Elements(Boolean array=w6899) -> (logical OR=w6902:bool)
    n1629 = case shown="True" w6902 {
      tunnel: w6901 -> [w6954 w6962]
      tunnel: w6900 -> [w6953 w6961]
      tunnel: [w6954 w6965] -> w6898
      tunnel: [w6953 w6964] -> w6897
      tunnel: w6899 -> [_ w6963]
      tunnel: "Dump Beads" -> [_ w6958]
      tunnel: w6882 -> [_ w6957]
      tunnel: "Upper Cap." -> [_ w6956]
      tunnel: "Data Acq. Spot" -> [_ w6955]
      frame #0 {
      }
      frame #1 {
        n1630 = flat-sequence {
          tunnel: w6963 -> [w6973]
          tunnel: w6962 -> [w6968]
          tunnel: w6961 -> [w6967]
          tunnel: [w6976] -> w6960
          tunnel: [w6975] -> w6959
          tunnel: [w6982] -> w6964
          tunnel: [w6983] -> w6965
          tunnel: w6960 -> [w6983]
          tunnel: w6959 -> [w6982]
          tunnel: w6958 -> [w6980]
          tunnel: w6957 -> [w6979]
          tunnel: w6956 -> [w6978]
          tunnel: w6955 -> [w6977]
          frame #0 {
            n1631 = Boolean Array To Number(Boolean array=w6973) -> (number=w6974:u32)
            n1632 = local read "Saved Stage Positions"() -> (w6972:T3)
            n1633 = Logarithm Base 2(1:w6974) -> (0:w6970:dbl)
            n1634 = Cluster To Array(cluster=w6972) -> (array=w6971:cluster{dbl, dbl, dbl}[])
            n1635 = Index Array(array=w6971, index=w6970) -> (element=w6969:cluster{dbl, dbl, dbl})
            n1636 = call "Set Stage Position.vi"("Position"=w6969, "error in"=w6967, "VISA resource name in"=w6968) -> ("error out"=w6975:errorcluster, "VISA resource name out"=w6976:refnum<visa-resource-name>)  [unwired: 1 out]
            "Stage Moving" <- TRUE ("Stage Moving")
          }
          frame #1 {
            n1637 = local write "Stage Moving"(FALSE ("Stage Moving")) -> ()
            n1638 = case shown="True" w6980 {
              frame #0 {
              }
              frame #1 {
                w6998 = FALSE ("Value (Signaling)")
                n1639 = property on="Green Laser ON/Interlacing" class="Bool (strict)"("Val(Sgnl)"=w6998) -> ()  [unwired: 2 in, 2 out]
                n1640 = property on="Trap 1 (ON/OFF)" class="Bool (strict)"("Val(Sgnl)"=w6998) -> ()  [unwired: 2 in, 2 out]
                n1641 = property on="Trap 2 (ON/OFF)" class="Bool (strict)"("Val(Sgnl)"=w6998) -> ()  [unwired: 2 in, 2 out]
              }
            }
            n1642 = call <vilib>:"Beep.vi"() -> ()  [unwired: 3 in, 9 out]
            n1643 = case shown="True" w6978 {
              selector: w6978 -> [_ w6996]
              frame #0 {
              }
              frame #1 {
                n1644 = property on="Trap 2 (ON/OFF)" class="Bool (strict)"("Val(Sgnl)"=w6996) -> ()  [unwired: 2 in, 2 out]
              }
            }
            n1645 = case shown="True" w6977 {
              selector: w6977 -> [_ w6984]
              frame #0 {
              }
              frame #1 {
                n1646 = flat-sequence {
                  tunnel: w6984 -> [w6985]
                  frame #0 {
                    n1647 = property on="Save Calibration" class="Bool (strict)"("Val(Sgnl)"=w6985) -> ()  [unwired: 2 in, 2 out]
                  }
                  frame #1 {
                    n1648 = Wait (ms)(milliseconds to wait=u32 2000) -> ()  [unwired: 1 out]
                  }
                  frame #2 {
                    n1649 = while {
                      stop <- w6987 stop-if-true
                      n1650 = local read "Saving..."() -> (w6988:bool)
                      n1651 = Wait (ms)(milliseconds to wait=u32 1000) -> ()  [unwired: 1 out]
                      n1652 = Not(x=w6988) -> (.not. x?=w6987:bool)
                    }
                  }
                  frame #3 {
                    n1653 = Multiply(x="Cal read wait (s)", y=u32 1000 ("milliseconds to wait")) -> (x*y=w6991:u32)
                    n1654 = Wait (ms)(milliseconds to wait=w6991) -> ()  [unwired: 1 out]
                  }
                  frame #4 {
                    n1655 = property on="Read Cal" class="Bool (strict)"("Val(Sgnl)"=TRUE ("Value (Signaling)")) -> ()  [unwired: 2 in, 2 out]
                  }
                  frame #5 {
                    n1656 = Wait (ms)(milliseconds to wait=u32 2000) -> ()  [unwired: 1 out]
                  }
                  frame #6 {
                    n1657 = property on="Fish for Tether" class="Bool (strict)"("Val(Sgnl)"=TRUE ("Value (Signaling)")) -> ()  [unwired: 2 in, 2 out]
                  }
                }
              }
            }
            n1658 = case shown="True" w6979 {
              selector: w6979 -> [_ w6997]
              frame #0 {
              }
              frame #1 {
                n1659 = property on="Trap 1 (ON/OFF)" class="Bool (strict)"("Val(Sgnl)"=w6997) -> ()  [unwired: 2 in, 2 out]
              }
            }
          }
        }
      }
    }
    n1660 = Or(x="+z", y="-z") -> (x .or. y?=w6896:bool)
    n1661 = case shown="True" w6896 {
      tunnel: w6898 -> [w6913 w6917]
      tunnel: w6897 -> [w6912 w6916]
      tunnel: [w6913 w6920] -> w6891
      tunnel: [w6912 w6919] -> w6890
      tunnel: "+z" -> [_ w6923]
      tunnel: "-z" -> [_ w6922]
      tunnel: w6893 -> [_ w6921]
      tunnel: w6892 -> [_ w6918]
      frame #0 {
      }
      frame #1 {
        n1662 = flat-sequence {
          tunnel: w6923 -> [w6949]
          tunnel: w6922 -> [w6948]
          tunnel: w6921 -> [w6944]
          tunnel: w6918 -> [w6929]
          tunnel: w6917 -> [w6926]
          tunnel: w6916 -> [w6925]
          tunnel: [w6936] -> w6915
          tunnel: [w6935] -> w6914
          tunnel: [w6951] -> w6919
          tunnel: [w6952] -> w6920
          tunnel: w6915 -> [w6952]
          tunnel: w6914 -> [w6951]
          frame #0 {
            n1663 = Boolean To (0,1)(Boolean=w6949) -> (0, 1=w6947:i16)
            n1664 = Boolean To (0,1)(Boolean=w6948) -> (0, 1=w6946:i16)
            n1665 = Unbundle(w6944) -> (w6943:dbl, w6942:dbl, w6938:dbl)
            n1666 = Divide(x="z nudge increment (um)", y=1000.0) -> (x/y=w6932:dbl)
            n1667 = Multiply(x=w6947, y=w6932) -> (x*y=w6940:dbl)
            n1668 = Multiply(x=w6946, y=w6932) -> (x*y=w6945:dbl)
            n1669 = Negate(x=w6945) -> (-x=w6941:dbl)
            n1670 = Add(x=w6940, y=w6941) -> (x+y=w6939:dbl)
            n1671 = local write "Stage Moving"(TRUE ("Stage Moving")) -> ()
            n1672 = Add(x=w6939, y=w6938) -> (x+y=w6931:dbl)
            n1673 = Unbundle(w6929) -> ("Minimum"=w6928:dbl, "Maximum"=w6927:dbl)  [unwired: 1 out]
            n1674 = In Range and Coerce(upper limit=w6927, x=w6931, lower limit=w6928) -> (coerced(x)=w6930:dbl)  [unwired: 1 out]
            n1675 = Bundle(cluster=w6944, w6943, w6942, w6930) -> (w6937:cluster{dbl, dbl, dbl})
            n1676 = call "Set Stage Position.vi"("Position"=w6937, "error in"=w6925, "VISA resource name in"=w6926) -> ("error out"=w6935:errorcluster, "VISA resource name out"=w6936:refnum<visa-resource-name>)  [unwired: 1 out]
          }
          frame #1 {
            n1677 = local write "Stage Moving"(FALSE ("Stage Moving")) -> ()
          }
        }
      }
    }
    n1678 = node-c288() -> ()  [unwired: 2 out]
  }
  n1679 = for "Create Greyscale map" {
    N: 256 -> [_]
    tunnel: [w7000] -> w183 mode=indexing
    i -> [w7003]
    n1680 = To Unsigned Byte Integer(number=w7003) -> (unsigned 8bit integer=w6999:u8)
    n1681 = Join Numbers(hi=w6999, lo=w6999) -> ((hi.lo)=w7002:u16)
    n1682 = Join Numbers(hi=w6999, lo=w6999) -> ((hi.lo)=w7001:u16)
    n1683 = Join Numbers(hi=w7002, lo=w7001) -> ((hi.lo)=w7000:u32)
  }
  n1684 = node-c288(w3) -> ()  [unwired: 1 out]
  n1685 = node-c288(w7) -> ()  [unwired: 1 out]
  n1686 = node-c288(w11) -> ()  [unwired: 1 out]
  n1687 = node-c288(w9) -> ()  [unwired: 1 out]
  n1688 = VISA Close(VISA resource name=w54, error in (no error)=w53) -> (error out=w58:errorcluster)
  n1689 = call <vilib>:"Simple Error Handler.vi"("error in (no error)"=w58) -> ()  [unwired: 1 in, 8 out]
  n1690 = node-c288(w5) -> ()  [unwired: 1 out]
  n1691 = node-c288(w122) -> ()  [unwired: 1 out]
  n1692 = flat-sequence {
    tunnel: w224 -> [w7007]
    tunnel: w226 -> [w7008]
    tunnel: [w7006] -> w204
    tunnel: [w7005] -> w203
    tunnel: w179 -> [_]
    tunnel: w177 -> [_]
    tunnel: w130 -> [_]
    tunnel: w13 -> [_]
    tunnel: w204 -> [w7066]
    tunnel: w203 -> [w7067]
    frame #0 {
      w7004 = FALSE ("AI to FIFO")
      n1693 = xnode "Read/Write Control"("FPGA VI Reference In"=w7008, "error in"=w7007, "AI to FIFO"=w7004, "APD to FIFO"=w7004) -> ("FPGA VI Reference Out"=w7006:T13, "error out"=w7005:errorcluster)
    }
    frame #1 {
      n1694 = xnode "Close FPGA VI Reference"("FPGA VI Reference In"=w7066, "error in"=w7067) -> ("error out"=→"error out":errorcluster)
    }
  }
